vi "HandleObservationSync_001.vi"(8 "error in (no error)":errorcluster, 11 "S4ACS_GUI in":refnum<class "S4GUI.lvclass">) -> (0 "error out":errorcluster, 3 "S4ACS_GUI out":refnum<class "S4GUI.lvclass">)   [LabVIEW 2018, in "S4GUI.lvclass"]
uses:
  S4GUI.lvclass
  S4GUI.lvclass/S4GUI.ctl
  Instrument/Instrument.lvclass/Instrument.ctl
  Device/Optics/Optics.lvclass/Optics.ctl
  Server/Server.lvclass/Server.ctl
  Interface/Interface.lvclass/Interface.ctl
  Device/Optics/Opt_Selector/Opt_Selector.lvclass
  C:/Users/observer/Desktop/Sparc4GUI/SPARC4_GUI/Device/Optics/Optics.lvclass
  Acquisition/Acquisition.lvclass
  C:/Users/observer/Desktop/Sparc4GUI/SPARC4_GUI/Server/Server.lvclass
  SyncBox/Sync Box.lvclass
  Instrument/Instrument.lvclass
  Device/Optics/Opt_Continuous/Opt_Continuous.lvclass
  StateMachine/State Machine.lvclass
  Trigger/Trigger.lvclass
  Channel/Channel.lvclass
  Interface/Interface.lvclass
  Device/Optics/Optics.lvclass
  Server/Server.lvclass
panel:
  out "delay 3-4":u32
  out "time4":u32
  out "time3":u32
  out "time 2":u32
  out "time1":u32
  # "WAVEPLATE DURATION"
  # "ACS SETUP"
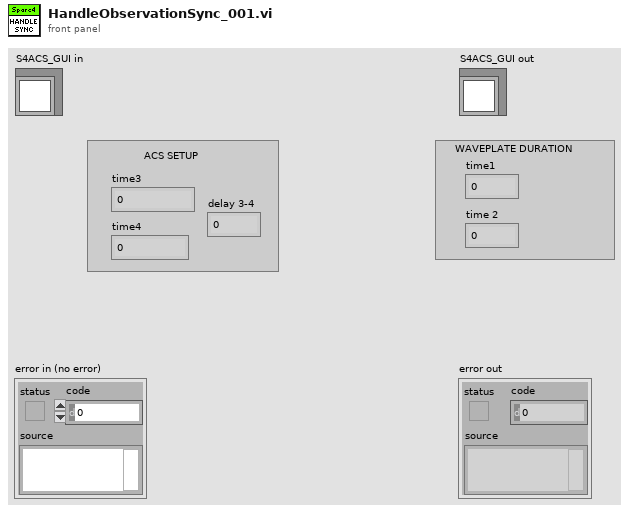
[diagram p1: front panel]
types:
  T1 = cluster{"ACQUISITION_MODE":u8, "TRIGGER_MODE":u8, "READ_MODE":u8, "PREAMP":u8, "READOUT_RATE":u8, "VERTICAL_SHIFT_SPEED":u8, "EM_MODE":u8, "EM_GAIN":u16, "SHUTTER_MODE":u8, "SHUTTER_TTL":u8, "SHUTTER_OPENING_TIME":u16, "SHUTTER_CLOSING_TIME":u16, "VBIN":u16, "HBIN":u16, "INITIAL_LINE":u16, "INITIAL_COLUMN":u16, "FINAL_LINE":u16, "FINAL_COLUMN":u16, "FRAME_TRANSFER":bool, "VERTICAL_CLOCK_VOLTAGE":u8, "AD_CHANNEL":u32}
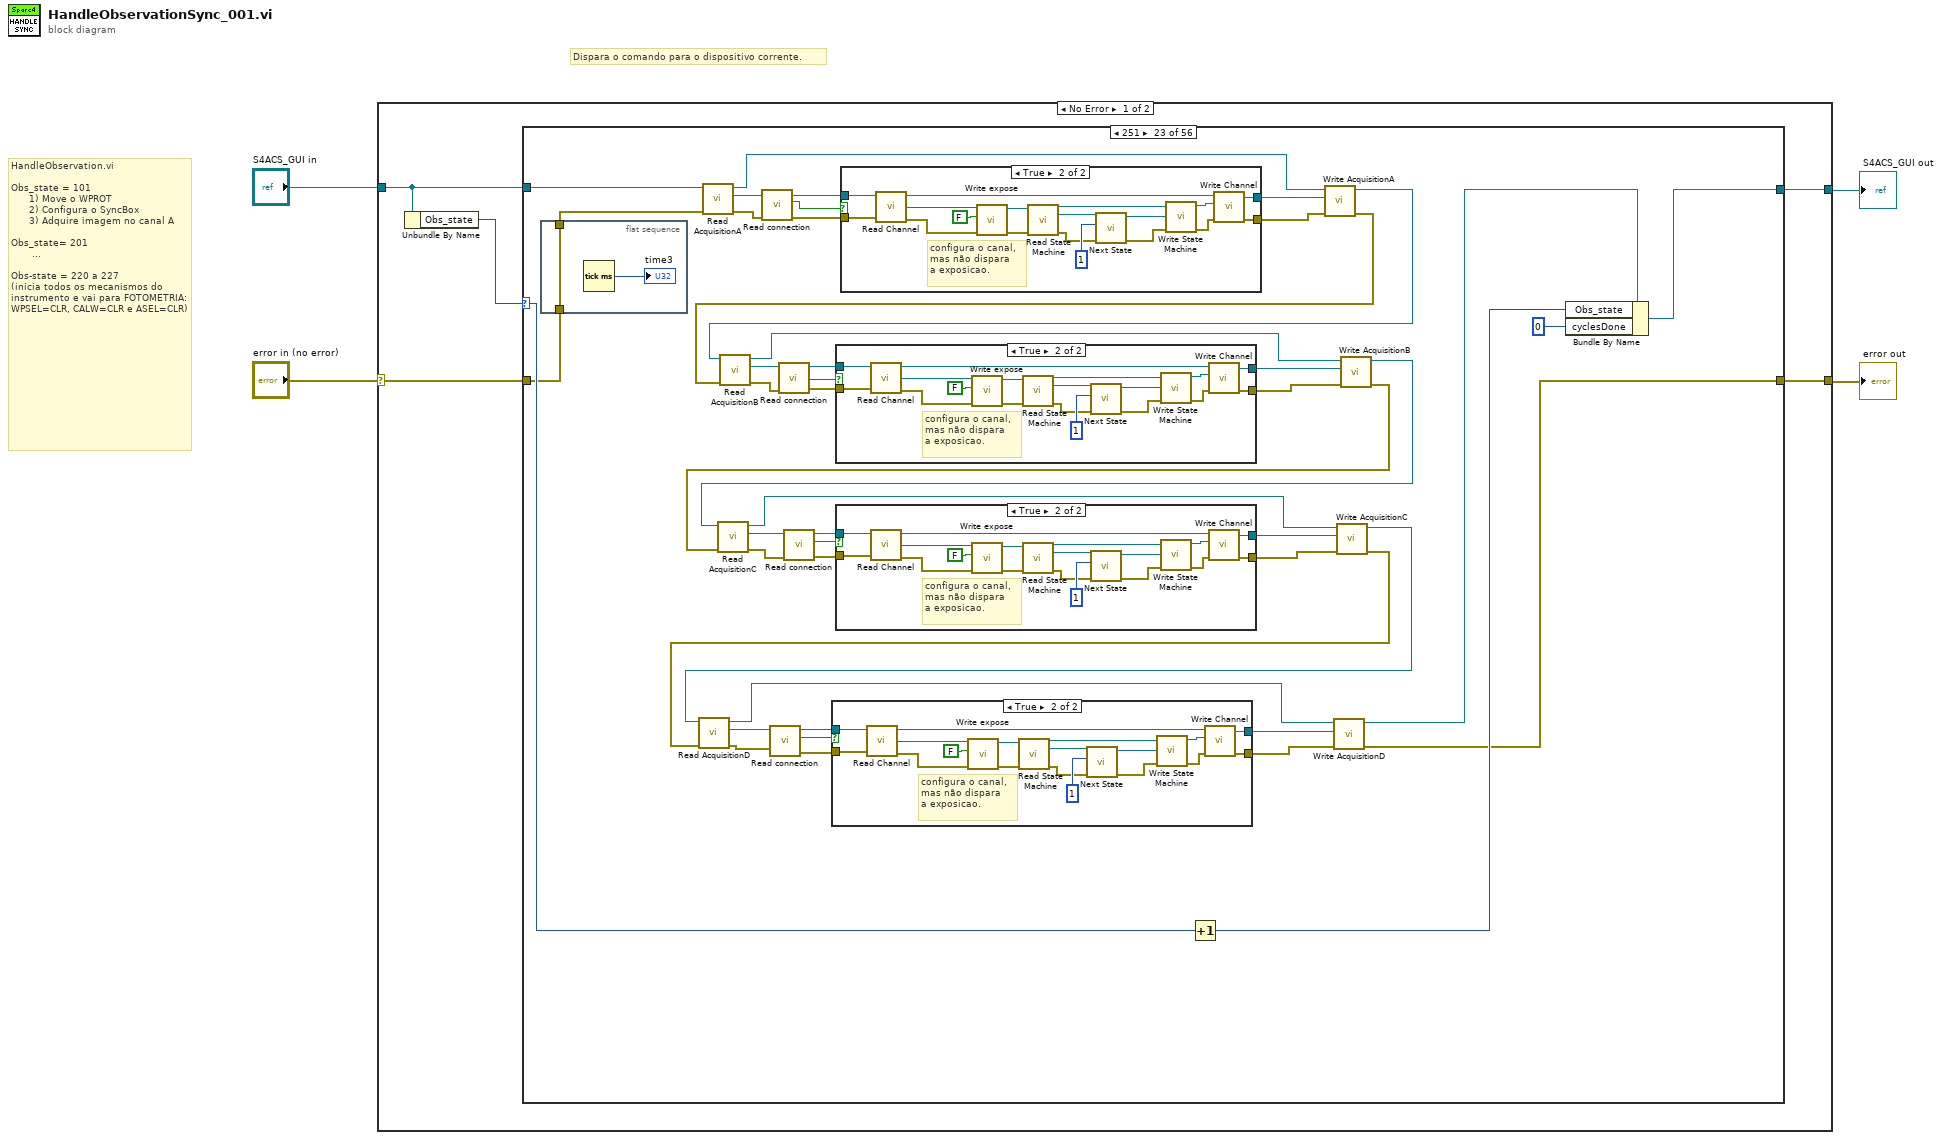
[diagram p0: block diagram]
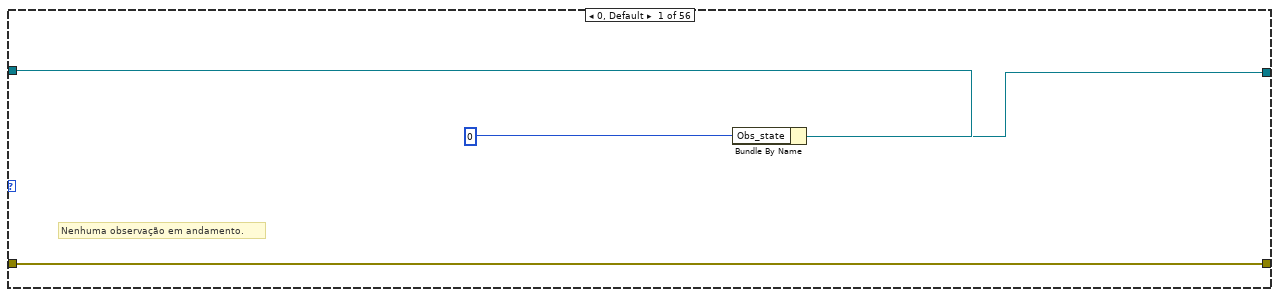
[diagram p2: hidden frame]
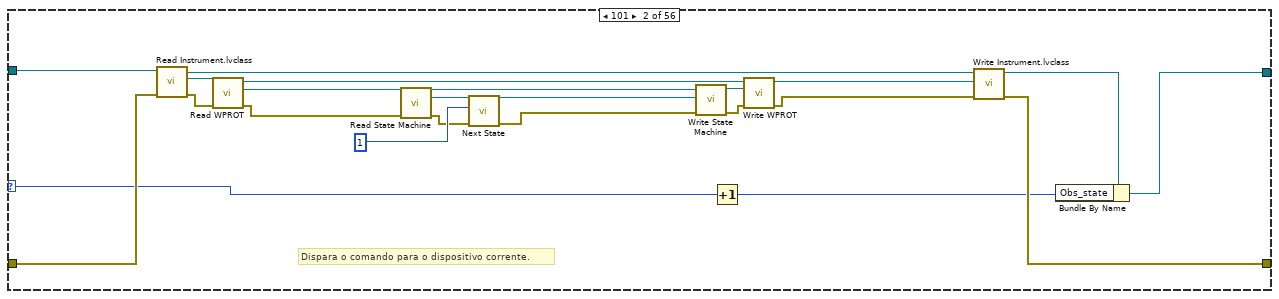
[diagram p3: hidden frame]
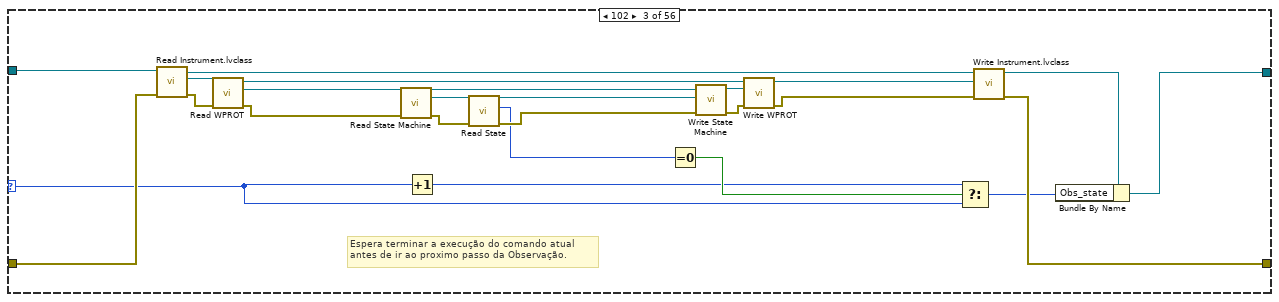
[diagram p4: hidden frame]
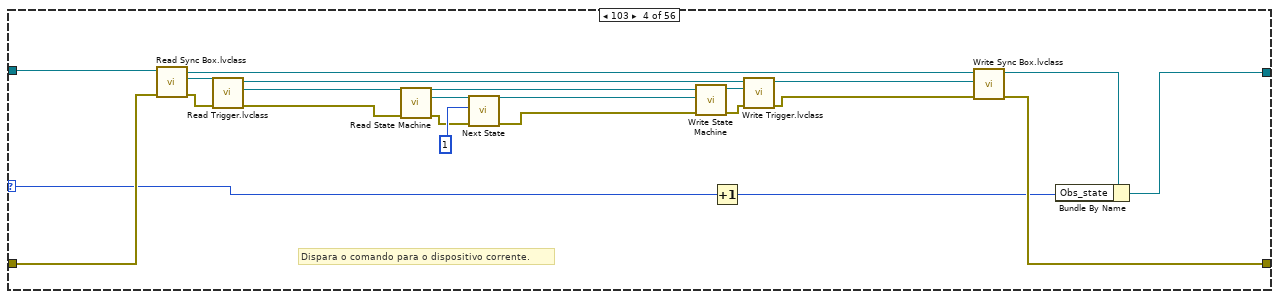
[diagram p5: hidden frame]
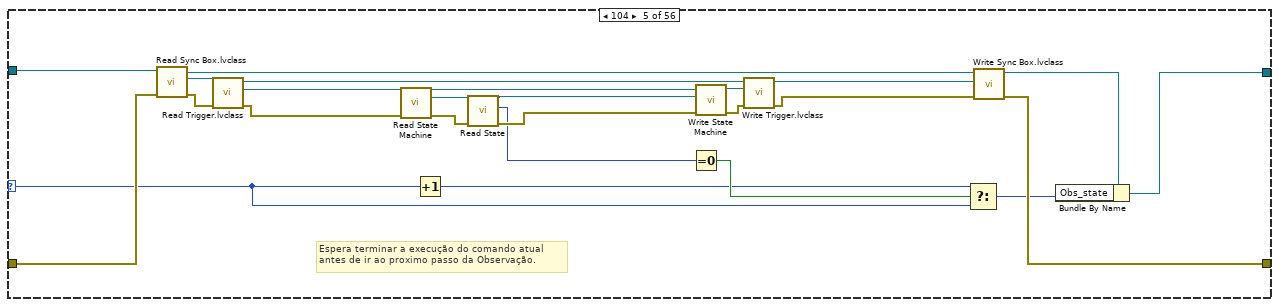
[diagram p6: hidden frame]
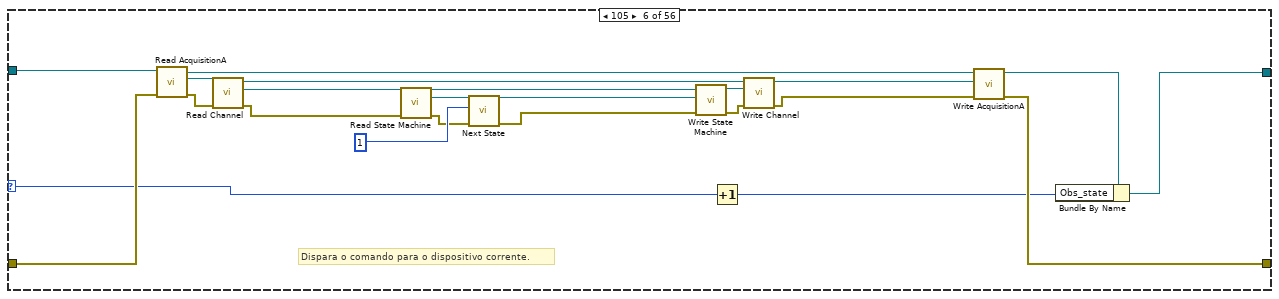
[diagram p7: hidden frame]
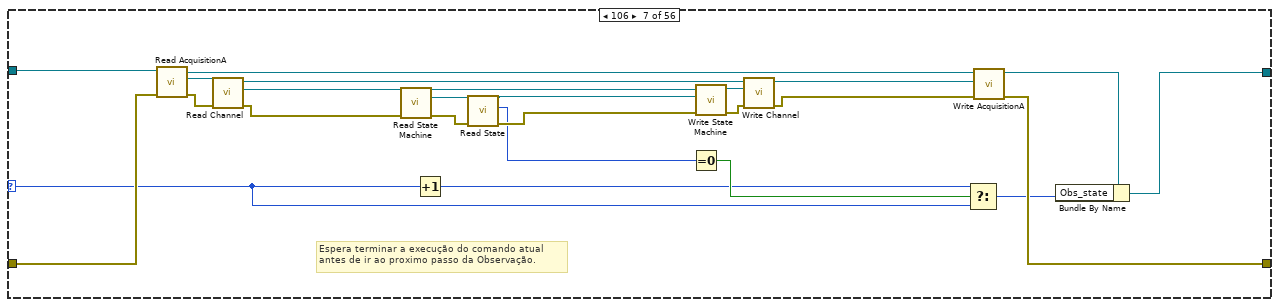
[diagram p8: hidden frame]
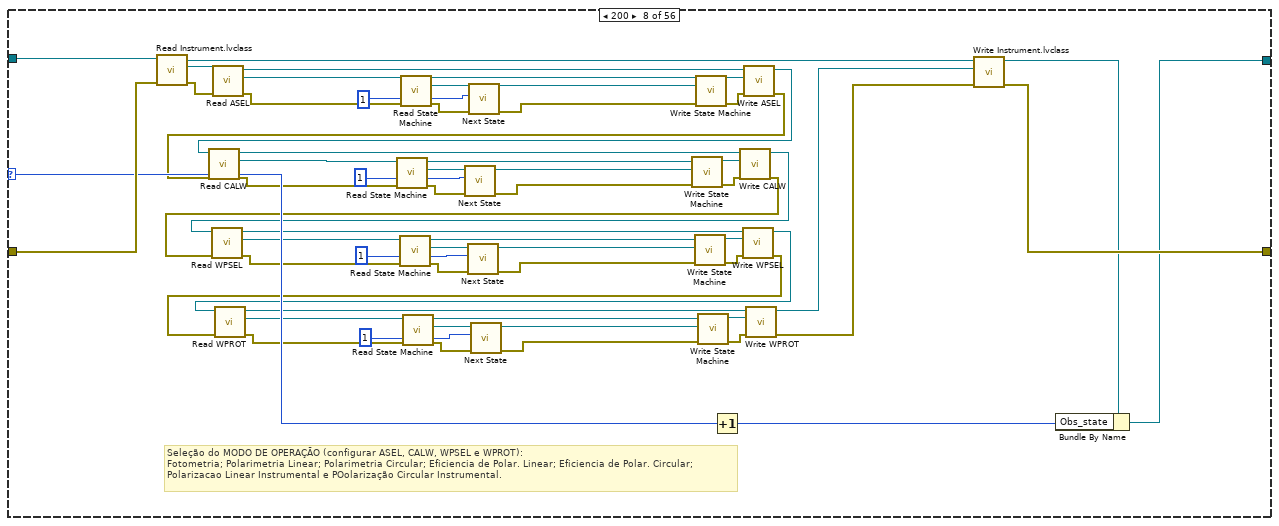
[diagram p9: hidden frame]
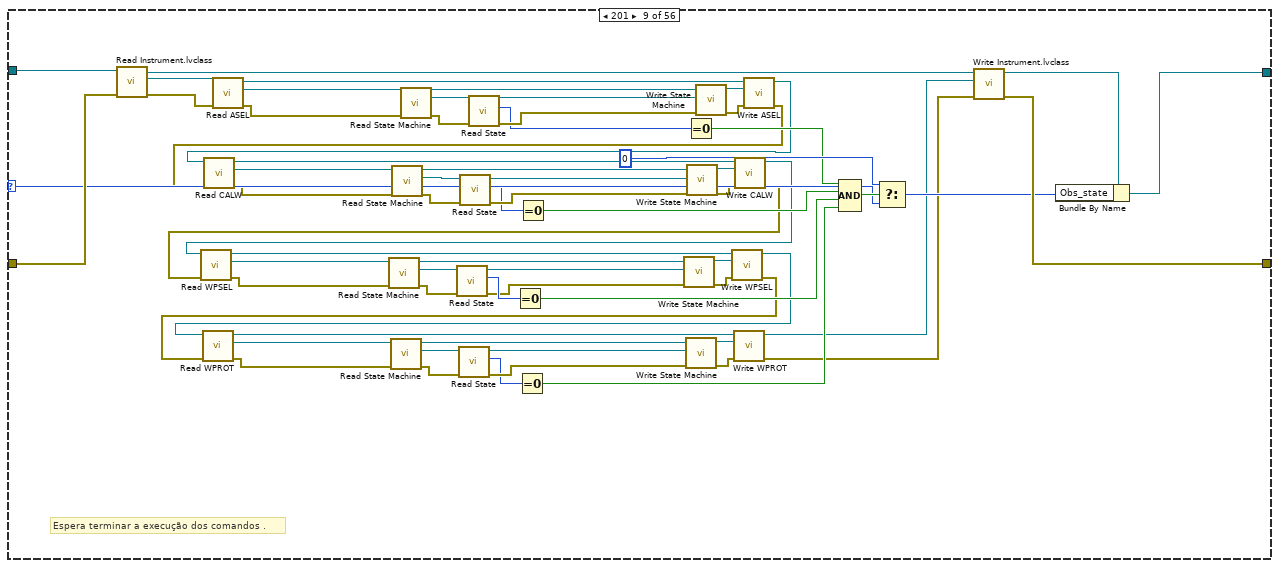
[diagram p10: hidden frame]
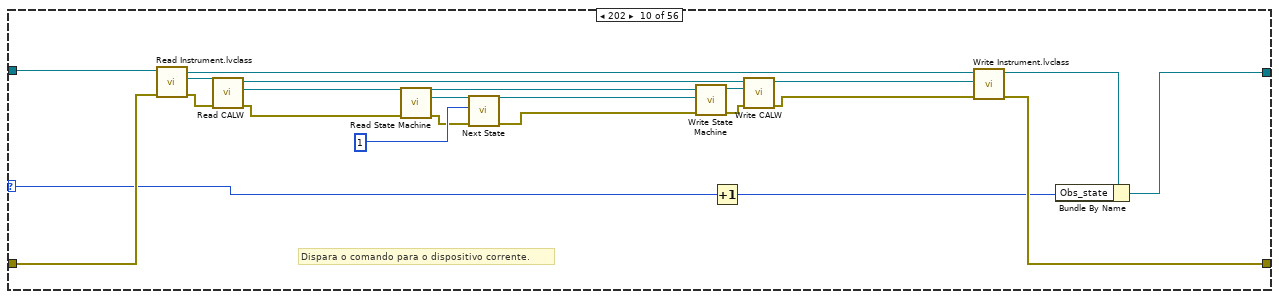
[diagram p11: hidden frame]
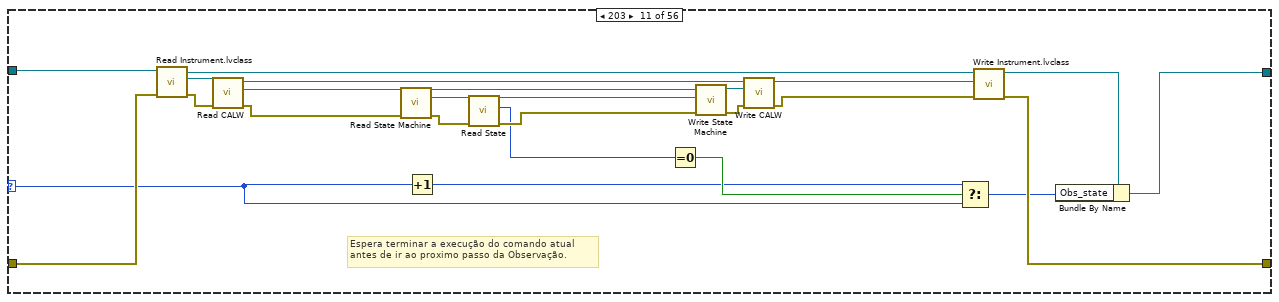
[diagram p12: hidden frame]
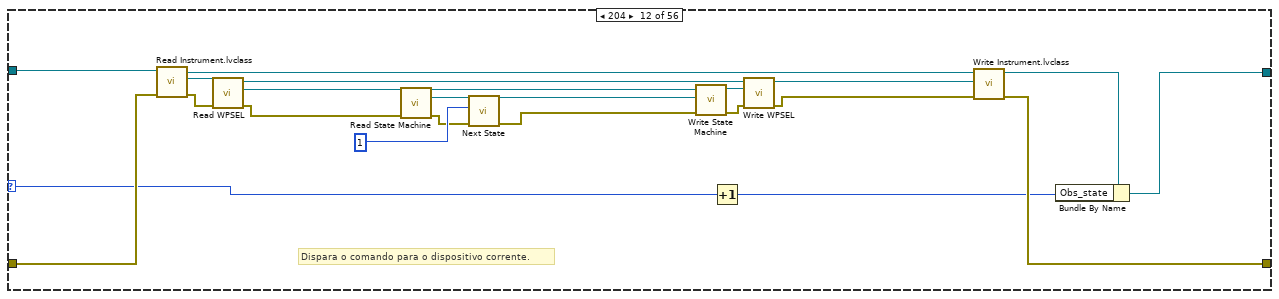
[diagram p13: hidden frame]
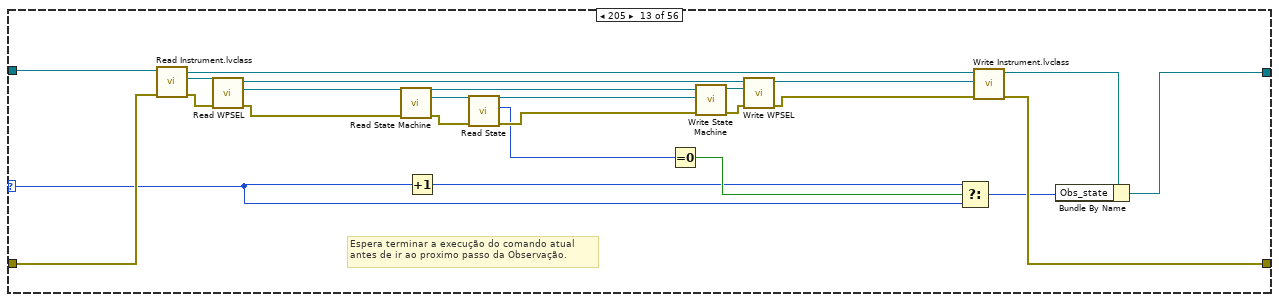
[diagram p14: hidden frame]
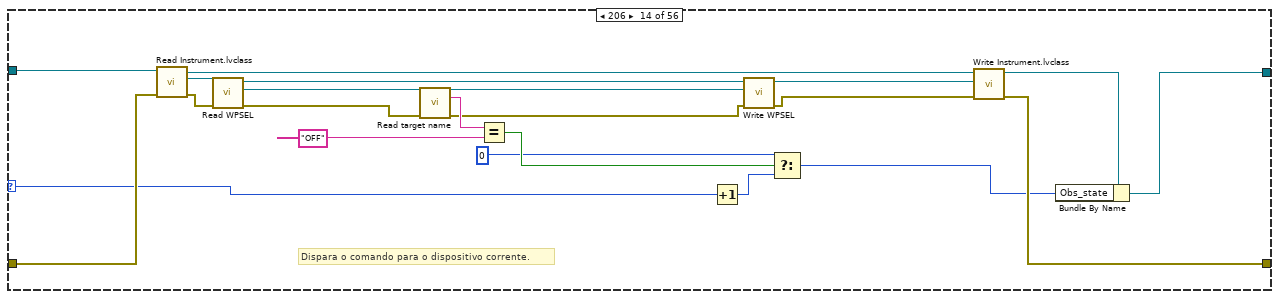
[diagram p15: hidden frame]
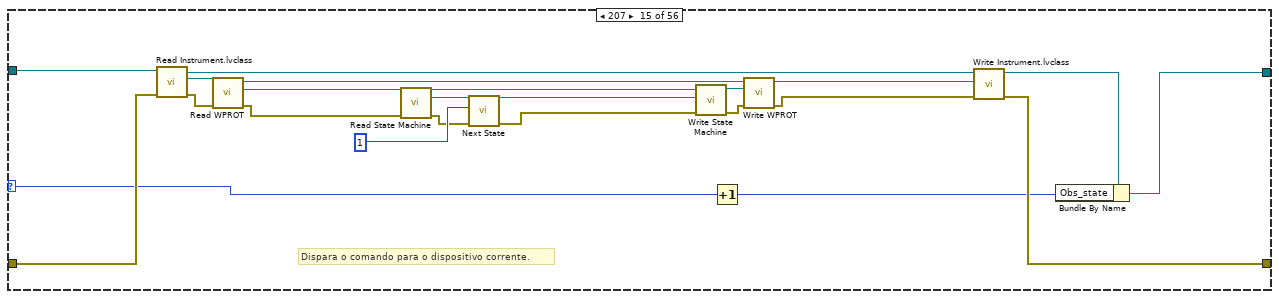
[diagram p16: hidden frame]
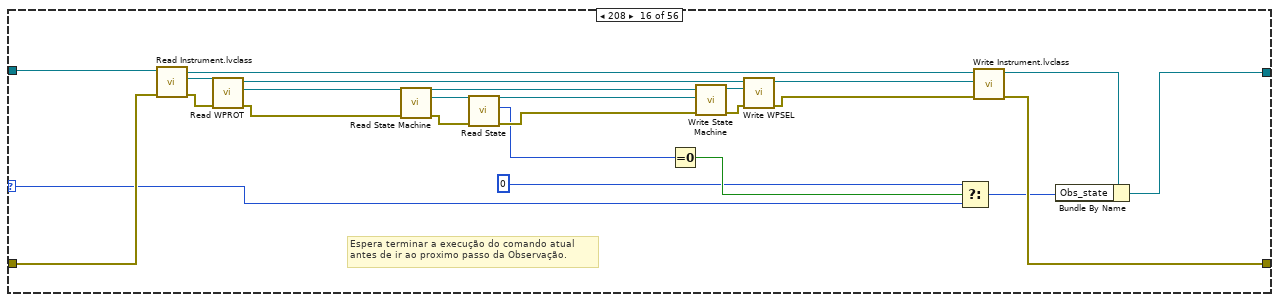
[diagram p17: hidden frame]
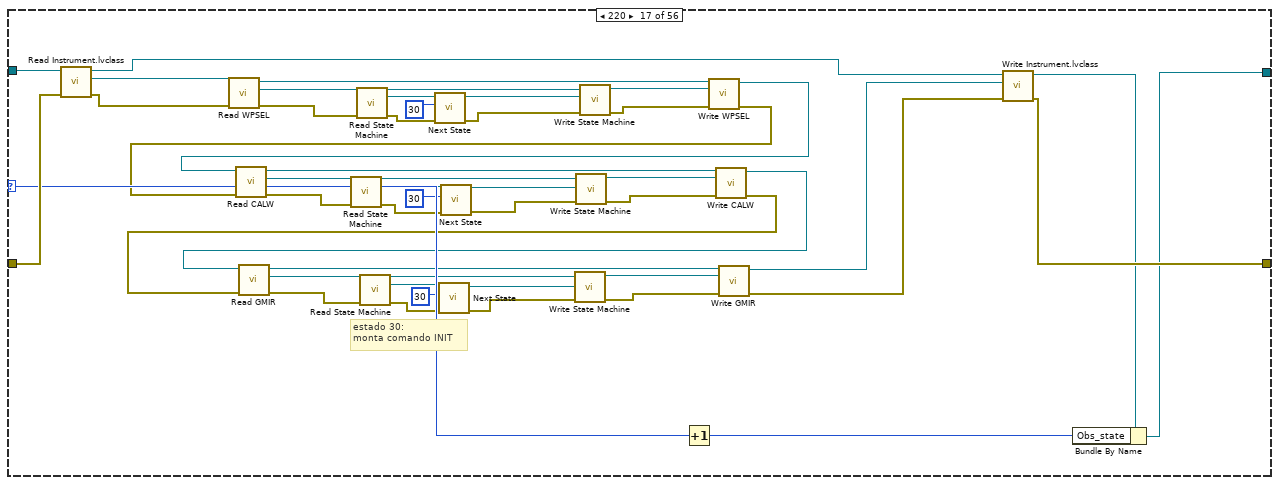
[diagram p18: hidden frame]
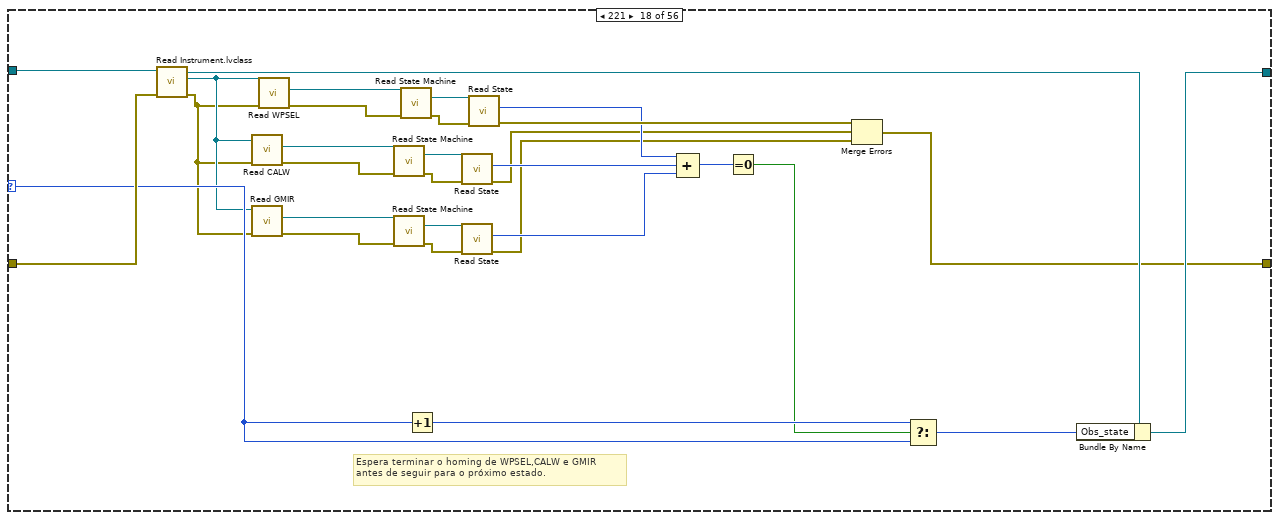
[diagram p19: hidden frame]
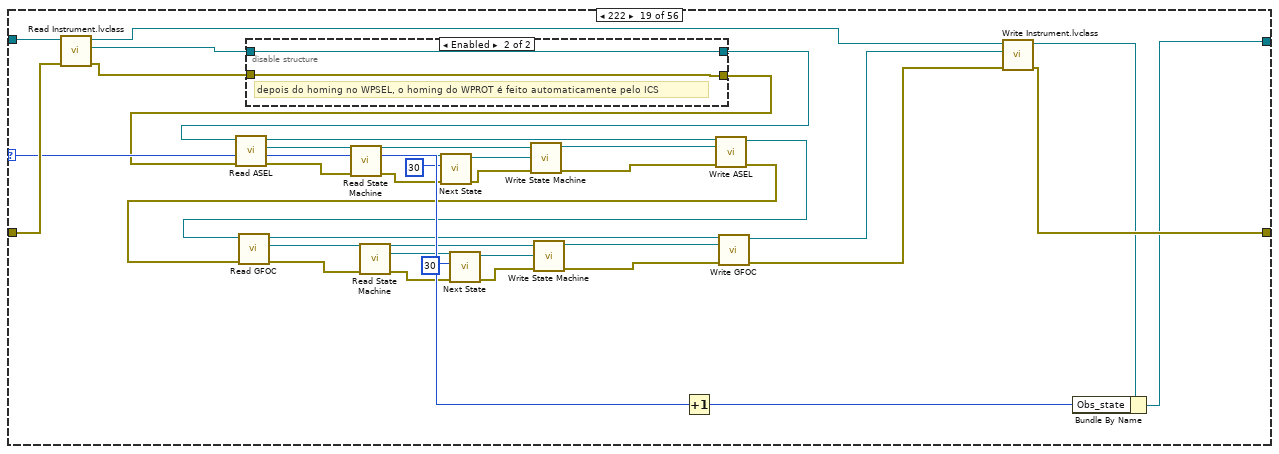
[diagram p20: hidden frame]
diagram:
  # "Dispara o comando para o dispositivo corrente."
  # "HandleObservation.vi\n\nObs_state = 101\n      1) Move o WPROT\n      2) Configura o SyncBox\n      3) Adquire imagem no canal A\n\nObs_state= 201\n       ...\n\nObs-state = 220 a 227 \n(inicia todos os mecanismos do instrumento e vai para FOTOMETRIA: WPSEL=CLR, CALW=CLR e ASEL=CLR)"
  n1 = case shown="No Error" "error in (no error)" {
    selector: "error in (no error)" -> [w8 w2964]
    tunnel: [w7 w2964] -> w3
    tunnel: [w9 w2963] -> w1
    tunnel: "S4ACS_GUI in" -> [w6 w2963]
    frame No Error {
      n2 = Unbundle By Name(w6) -> ("Obs_state"=w5:u32)
      n3 = case shown="251" w5 {
        selector: w5 -> [_ w16 w38 w64 w86 w112 w134 w202 w265 w290 w312 w338 w360 w395 w408 w430 w492 w524 w563 w609 w689 w721 w767 w904 w1029 w1032 w1067 w1103 w1175 w1179 w1210 w1246 w1318 w1322 w1353 w1385 w1455 w1459 _ w1536 w1581 w1653 w1733 w1867 w2024 _ _ w2263 _ w2411 w2523 w2620 w2770 w2841 _ _]
        tunnel: w6 -> [w12 w30 w55 w78 w103 w126 w151 w216 w283 w304 w329 w352 w377 w399 w422 w447 w501 w532 w569 w613 w698 w729 w773 w908 w1022 w1050 w1071 w1120 w1168 w1196 w1214 w1263 w1311 w1339 w1357 w1402 w1448 w1476 w1496 w1539 w1603 w1655 w1774 w1871 w2022 w2062 w2194 w2272 w2361 w2370 w2527 w2624 w2783 w2803 w2931 w2962]
        tunnel: [w10 w14 w42 w62 w94 w110 w142 w200 w270 w288 w316 w336 w364 w394 w406 w434 w496 w526 w564 w611 w693 w723 w772 w907 w1027 w1041 w1065 w1111 w1173 w1187 w1208 w1254 w1316 w1330 w1351 w1393 w1453 w1467 w1495 w1534 w1584 w1651 w1772 w1865 w2030 w2100 w2191 w2270 w2357 w2409 w2525 w2618 w2776 w2842 w2928 w2962] -> w9
        tunnel: w8 -> [w13 w29 w54 w77 w102 w125 w150 w215 w282 w303 w328 w351 w376 w398 w421 w446 w500 w531 w568 w612 w697 w728 w748 w890 w1023 w1049 w1070 w1119 w1169 w1195 w1213 w1262 w1312 w1338 w1356 w1401 w1449 w1475 w1486 w1504 w1594 w1654 w1773 w1870 w2020 w2101 w2193 w2271 w2360 w2369 w2526 w2623 w2782 w2843 w2930 w2961]
        tunnel: [w13 w28 w53 w76 w101 w124 w149 w214 w281 w302 w327 w350 w375 w397 w420 w445 w499 w505 w567 w590 w696 w703 w750 w892 w1020 w1048 w1069 w1118 w1166 w1194 w1212 w1261 w1309 w1337 w1355 w1400 w1446 w1474 w1487 w1538 w1580 w1635 w1755 w1869 w2012 w2083 w2192 w2245 w2359 w2367 w2505 w2622 w2765 w2824 w2929 w2961] -> w7
        frame 0, Default {
          # "Nenhuma observação em andamento."
          n4 = Bundle By Name(cluster=w12, "Obs_state"=u32 0) -> (w10:refnum<class "S4GUI.lvclass">)
        }
        frame 101 {
          # "Dispara o comando para o dispositivo corrente."
          n5 = call "Read Instrument.lvclass.vi"("error in (no error)"=w29, "S4ACS_GUI in"=w30) -> ("error out"=w35:errorcluster, "Instrument.lvclass"=w36:refnum<class "Instrument.lvclass">, "S4ACS_GUI out"=w32:refnum<class "S4GUI.lvclass">)  [unwired: 7 in]
          n6 = call "Read WPROT.vi"("error in (no error)"=w35, "Instrument in"=w36) -> ("error out"=w22:errorcluster, "Opt_Selector.lvclass"=w21:refnum<class "Opt_Selector.lvclass">, "Instrument out"=w34:refnum<class "Instrument.lvclass">)  [unwired: 7 in]
          n7 = call-dynamic "Read State Machine.vi"("error in (no error)"=w22, "Device in"=w21) -> ("error out"=w25:errorcluster, "State Machine.lvclass"=w27:refnum<class "State Machine.lvclass">, "Device out"=w19:refnum<class "Opt_Selector.lvclass">)  [unwired: 7 in]
          n8 = call "Next State.vi"("error in (no error)"=w25, "New_State"=1, "State Machine in"=w27) -> ("error out"=w24:errorcluster, "State Machine out"=w23:refnum<class "State Machine.lvclass">)  [unwired: 7 in]
          n9 = call-dynamic "Write State Machine.vi"("error in (no error)"=w24, "State Machine.lvclass"=w23, "Device in"=w19) -> ("error out"=w18:errorcluster, "Device out"=w20:refnum<class "Opt_Selector.lvclass">)  [unwired: 7 in]
          n10 = Increment(x=w16) -> (x+1=w15:u32)
          n11 = call "Write WPROT.vi"("error in (no error)"=w18, "Opt_Selector.lvclass"=w20, "Instrument in"=w34) -> ("error out"=w31:errorcluster, "Instrument out"=w33:refnum<class "Instrument.lvclass">)  [unwired: 7 in]
          n12 = call "Write Instrument.lvclass.vi"("error in (no error)"=w31, "Instrument.lvclass"=w33, "S4ACS_GUI in"=w32) -> ("error out"=w28:errorcluster, "S4ACS_GUI out"=w17:refnum<class "S4GUI.lvclass">)  [unwired: 7 in]
          n13 = Bundle By Name(cluster=w17, "Obs_state"=w15) -> (w14:refnum<class "S4GUI.lvclass">)
        }
        frame 102 {
          # "Espera terminar a execução do comando atual \nantes de ir ao proximo passo da Observação."
          n14 = call "Read Instrument.lvclass.vi"("error in (no error)"=w54, "S4ACS_GUI in"=w55) -> ("error out"=w60:errorcluster, "Instrument.lvclass"=w61:refnum<class "Instrument.lvclass">, "S4ACS_GUI out"=w57:refnum<class "S4GUI.lvclass">)  [unwired: 7 in]
          n15 = call "Read WPROT.vi"("error in (no error)"=w60, "Instrument in"=w61) -> ("error out"=w48:errorcluster, "Opt_Selector.lvclass"=w47:refnum<class "Opt_Selector.lvclass">, "Instrument out"=w59:refnum<class "Instrument.lvclass">)  [unwired: 7 in]
          n16 = call-dynamic "Read State Machine.vi"("error in (no error)"=w48, "Device in"=w47) -> ("error out"=w51:errorcluster, "State Machine.lvclass"=w52:refnum<class "State Machine.lvclass">, "Device out"=w45:refnum<class "Opt_Selector.lvclass">)  [unwired: 7 in]
          n17 = Increment(x=w38) -> (x+1=w37:u32)
          n18 = call-dynamic "Read State.vi"("error in (no error)"=w51, "State Machine in"=w52) -> ("error out"=w50:errorcluster, "State"=w40:i32, "State Machine out"=w49:refnum<class "State Machine.lvclass">)  [unwired: 7 in]
          n19 = Equal To 0?(x=w40) -> (x = 0?=w41:bool)
          n20 = call-dynamic "Write State Machine.vi"("error in (no error)"=w50, "State Machine.lvclass"=w49, "Device in"=w45) -> ("error out"=w44:errorcluster, "Device out"=w46:refnum<class "Opt_Selector.lvclass">)  [unwired: 7 in]
          n21 = call "Write WPROT.vi"("error in (no error)"=w44, "Opt_Selector.lvclass"=w46, "Instrument in"=w59) -> ("error out"=w56:errorcluster, "Instrument out"=w58:refnum<class "Instrument.lvclass">)  [unwired: 7 in]
          n22 = Select(t=w37, s=w41, f=w38) -> (s? t:f=w39:u32)
          n23 = call "Write Instrument.lvclass.vi"("error in (no error)"=w56, "Instrument.lvclass"=w58, "S4ACS_GUI in"=w57) -> ("error out"=w53:errorcluster, "S4ACS_GUI out"=w43:refnum<class "S4GUI.lvclass">)  [unwired: 7 in]
          n24 = Bundle By Name(cluster=w43, "Obs_state"=w39) -> (w42:refnum<class "S4GUI.lvclass">)
        }
        frame 103 {
          # "Dispara o comando para o dispositivo corrente."
          n25 = call-dynamic "Read Sync Box.lvclass.vi"("error in (no error)"=w77, "SPARC4_AC in"=w78) -> ("error out"=w83:errorcluster, "Sync Box.lvclass"=w84:refnum<class "Sync Box.lvclass">, "SPARC4_AC out"=w80:refnum<class "S4GUI.lvclass">)  [unwired: 7 in]
          n26 = call-dynamic "Read Trigger.lvclass.vi"("error in (no error)"=w83, "Sync Box in"=w84) -> ("error out"=w70:errorcluster, "Trigger.lvclass"=w69:refnum<class "Trigger.lvclass">, "Sync Box out"=w82:refnum<class "Sync Box.lvclass">)  [unwired: 7 in]
          n27 = call-dynamic "Read State Machine.vi"("error in (no error)"=w70, "Device in"=w69) -> ("error out"=w73:errorcluster, "State Machine.lvclass"=w75:refnum<class "State Machine.lvclass">, "Device out"=w67:refnum<class "Trigger.lvclass">)  [unwired: 7 in]
          n28 = call "Next State.vi"("error in (no error)"=w73, "New_State"=1, "State Machine in"=w75) -> ("error out"=w72:errorcluster, "State Machine out"=w71:refnum<class "State Machine.lvclass">)  [unwired: 7 in]
          n29 = call-dynamic "Write State Machine.vi"("error in (no error)"=w72, "State Machine.lvclass"=w71, "Device in"=w67) -> ("error out"=w66:errorcluster, "Device out"=w68:refnum<class "Trigger.lvclass">)  [unwired: 7 in]
          n30 = Increment(x=w64) -> (x+1=w63:u32)
          n31 = call-dynamic "Write Trigger.lvclass.vi"("error in (no error)"=w66, "Trigger.lvclass"=w68, "Sync Box in"=w82) -> ("error out"=w79:errorcluster, "Sync Box out"=w81:refnum<class "Sync Box.lvclass">)  [unwired: 7 in]
          n32 = call-dynamic "Write Sync Box.lvclass.vi"("error in (no error)"=w79, "Sync Box.lvclass"=w81, "SPARC4_AC in"=w80) -> ("error out"=w76:errorcluster, "SPARC4_AC out"=w65:refnum<class "S4GUI.lvclass">)  [unwired: 7 in]
          n33 = Bundle By Name(cluster=w65, "Obs_state"=w63) -> (w62:refnum<class "S4GUI.lvclass">)
        }
        frame 104 {
          # "Espera terminar a execução do comando atual \nantes de ir ao proximo passo da Observação."
          n34 = call-dynamic "Read Sync Box.lvclass.vi"("error in (no error)"=w102, "SPARC4_AC in"=w103) -> ("error out"=w108:errorcluster, "Sync Box.lvclass"=w109:refnum<class "Sync Box.lvclass">, "SPARC4_AC out"=w105:refnum<class "S4GUI.lvclass">)  [unwired: 7 in]
          n35 = call-dynamic "Read Trigger.lvclass.vi"("error in (no error)"=w108, "Sync Box in"=w109) -> ("error out"=w100:errorcluster, "Trigger.lvclass"=w99:refnum<class "Trigger.lvclass">, "Sync Box out"=w107:refnum<class "Sync Box.lvclass">)  [unwired: 7 in]
          n36 = call-dynamic "Read State Machine.vi"("error in (no error)"=w100, "Device in"=w99) -> ("error out"=w91:errorcluster, "State Machine.lvclass"=w93:refnum<class "State Machine.lvclass">, "Device out"=w97:refnum<class "Trigger.lvclass">)  [unwired: 7 in]
          n37 = Increment(x=w86) -> (x+1=w88:u32)
          n38 = call-dynamic "Read State.vi"("error in (no error)"=w91, "State Machine in"=w93) -> ("error out"=w90:errorcluster, "State"=w85:i32, "State Machine out"=w92:refnum<class "State Machine.lvclass">)  [unwired: 7 in]
          n39 = Equal To 0?(x=w85) -> (x = 0?=w89:bool)
          n40 = call-dynamic "Write State Machine.vi"("error in (no error)"=w90, "State Machine.lvclass"=w92, "Device in"=w97) -> ("error out"=w96:errorcluster, "Device out"=w98:refnum<class "Trigger.lvclass">)  [unwired: 7 in]
          n41 = call-dynamic "Write Trigger.lvclass.vi"("error in (no error)"=w96, "Trigger.lvclass"=w98, "Sync Box in"=w107) -> ("error out"=w104:errorcluster, "Sync Box out"=w106:refnum<class "Sync Box.lvclass">)  [unwired: 7 in]
          n42 = Select(t=w88, s=w89, f=w86) -> (s? t:f=w87:u32)
          n43 = call-dynamic "Write Sync Box.lvclass.vi"("error in (no error)"=w104, "Sync Box.lvclass"=w106, "SPARC4_AC in"=w105) -> ("error out"=w101:errorcluster, "SPARC4_AC out"=w95:refnum<class "S4GUI.lvclass">)  [unwired: 7 in]
          n44 = Bundle By Name(cluster=w95, "Obs_state"=w87) -> (w94:refnum<class "S4GUI.lvclass">)
        }
        frame 105 {
          # "Dispara o comando para o dispositivo corrente."
          n45 = call-dynamic "Read AcquisitionA.vi"("error in (no error)"=w125, "S4ACS_GUI in"=w126) -> ("error out"=w131:errorcluster, "Acquisition.lvclass"=w132:refnum<class "Acquisition.lvclass">, "S4ACS_GUI out"=w128:refnum<class "S4GUI.lvclass">)  [unwired: 7 in]
          n46 = call-dynamic "Read Channel.vi"("error in (no error)"=w131, "Acquisition in"=w132) -> ("error out"=w118:errorcluster, "Channel.lvclass"=w117:refnum<class "Channel.lvclass">, "Acquisition out"=w130:refnum<class "Acquisition.lvclass">)  [unwired: 7 in]
          n47 = call-dynamic "Read State Machine.vi"("error in (no error)"=w118, "Device in"=w117) -> ("error out"=w121:errorcluster, "State Machine.lvclass"=w123:refnum<class "State Machine.lvclass">, "Device out"=w115:refnum<class "Channel.lvclass">)  [unwired: 7 in]
          n48 = call "Next State.vi"("error in (no error)"=w121, "New_State"=1, "State Machine in"=w123) -> ("error out"=w120:errorcluster, "State Machine out"=w119:refnum<class "State Machine.lvclass">)  [unwired: 7 in]
          n49 = call-dynamic "Write State Machine.vi"("error in (no error)"=w120, "State Machine.lvclass"=w119, "Device in"=w115) -> ("error out"=w114:errorcluster, "Device out"=w116:refnum<class "Channel.lvclass">)  [unwired: 7 in]
          n50 = Increment(x=w112) -> (x+1=w111:u32)
          n51 = call-dynamic "Write Channel.vi"("error in (no error)"=w114, "Channel.lvclass"=w116, "Acquisition in"=w130) -> ("error out"=w127:errorcluster, "Acquisition out"=w129:refnum<class "Acquisition.lvclass">)  [unwired: 7 in]
          n52 = call-dynamic "Write AcquisitionA.vi"("error in (no error)"=w127, "Acquisition.lvclass"=w129, "S4ACS_GUI in"=w128) -> ("error out"=w124:errorcluster, "S4ACS_GUI out"=w113:refnum<class "S4GUI.lvclass">)  [unwired: 7 in]
          n53 = Bundle By Name(cluster=w113, "Obs_state"=w111) -> (w110:refnum<class "S4GUI.lvclass">)
        }
        frame 106 {
          # "Espera terminar a execução do comando atual \nantes de ir ao proximo passo da Observação."
          n54 = call-dynamic "Read AcquisitionA.vi"("error in (no error)"=w150, "S4ACS_GUI in"=w151) -> ("error out"=w156:errorcluster, "Acquisition.lvclass"=w157:refnum<class "Acquisition.lvclass">, "S4ACS_GUI out"=w153:refnum<class "S4GUI.lvclass">)  [unwired: 7 in]
          n55 = call-dynamic "Read Channel.vi"("error in (no error)"=w156, "Acquisition in"=w157) -> ("error out"=w148:errorcluster, "Channel.lvclass"=w147:refnum<class "Channel.lvclass">, "Acquisition out"=w155:refnum<class "Acquisition.lvclass">)  [unwired: 7 in]
          n56 = call-dynamic "Read State Machine.vi"("error in (no error)"=w148, "Device in"=w147) -> ("error out"=w139:errorcluster, "State Machine.lvclass"=w141:refnum<class "State Machine.lvclass">, "Device out"=w145:refnum<class "Channel.lvclass">)  [unwired: 7 in]
          n57 = Increment(x=w134) -> (x+1=w136:u32)
          n58 = call-dynamic "Read State.vi"("error in (no error)"=w139, "State Machine in"=w141) -> ("error out"=w138:errorcluster, "State"=w133:i32, "State Machine out"=w140:refnum<class "State Machine.lvclass">)  [unwired: 7 in]
          n59 = Equal To 0?(x=w133) -> (x = 0?=w137:bool)
          n60 = call-dynamic "Write State Machine.vi"("error in (no error)"=w138, "State Machine.lvclass"=w140, "Device in"=w145) -> ("error out"=w144:errorcluster, "Device out"=w146:refnum<class "Channel.lvclass">)  [unwired: 7 in]
          n61 = call-dynamic "Write Channel.vi"("error in (no error)"=w144, "Channel.lvclass"=w146, "Acquisition in"=w155) -> ("error out"=w152:errorcluster, "Acquisition out"=w154:refnum<class "Acquisition.lvclass">)  [unwired: 7 in]
          n62 = Select(t=w136, s=w137, f=w134) -> (s? t:f=w135:u32)
          n63 = call-dynamic "Write AcquisitionA.vi"("error in (no error)"=w152, "Acquisition.lvclass"=w154, "S4ACS_GUI in"=w153) -> ("error out"=w149:errorcluster, "S4ACS_GUI out"=w143:refnum<class "S4GUI.lvclass">)  [unwired: 7 in]
          n64 = Bundle By Name(cluster=w143, "Obs_state"=w135) -> (w142:refnum<class "S4GUI.lvclass">)
        }
        frame 200 {
          # "Seleção do MODO DE OPERAÇÃO (configurar ASEL, CALW, WPSEL e WPROT): \nFotometria; Polarimetria Linear; Polarimetria Circular; Eficiencia de Polar. Linear; Eficiencia de Polar. Circular;\nPolarizacao Linear Instrumental e POolarização Circular Instrumental."
          n65 = call "Read Instrument.lvclass.vi"("error in (no error)"=w215, "S4ACS_GUI in"=w216) -> ("error out"=w219:errorcluster, "Instrument.lvclass"=w179:refnum<class "Instrument.lvclass">, "S4ACS_GUI out"=w217:refnum<class "S4GUI.lvclass">)  [unwired: 7 in]
          n66 = call "Read ASEL.vi"("error in (no error)"=w219, "Instrument in"=w179) -> ("error out"=w208:errorcluster, "Opt_Selector.lvclass"=w207:refnum<class "Opt_Selector.lvclass">, "Instrument out"=w218:refnum<class "Instrument.lvclass">)  [unwired: 7 in]
          n67 = call-dynamic "Read State Machine.vi"("error in (no error)"=w208, "Device in"=w207) -> ("error out"=w211:errorcluster, "State Machine.lvclass"=w213:refnum<class "State Machine.lvclass">, "Device out"=w205:refnum<class "Opt_Selector.lvclass">)  [unwired: 7 in]
          n68 = call "Next State.vi"("error in (no error)"=w211, "New_State"=1, "State Machine in"=w213) -> ("error out"=w210:errorcluster, "State Machine out"=w209:refnum<class "State Machine.lvclass">)  [unwired: 7 in]
          n69 = call-dynamic "Write State Machine.vi"("error in (no error)"=w210, "State Machine.lvclass"=w209, "Device in"=w205) -> ("error out"=w204:errorcluster, "Device out"=w206:refnum<class "Opt_Selector.lvclass">)  [unwired: 7 in]
          n70 = Increment(x=w202) -> (x+1=w201:u32)
          n71 = call "Write ASEL.vi"("error in (no error)"=w204, "Opt_Selector.lvclass"=w206, "Instrument in"=w218) -> ("error out"=w160:errorcluster, "Instrument out"=w178:refnum<class "Instrument.lvclass">)  [unwired: 7 in]
          n72 = call "Read CALW.vi"("error in (no error)"=w160, "Instrument in"=w178) -> ("error out"=w195:errorcluster, "Opt_Selector.lvclass"=w196:refnum<class "Opt_Selector.lvclass">, "Instrument out"=w177:refnum<class "Instrument.lvclass">)  [unwired: 7 in]
          n73 = call-dynamic "Read State Machine.vi"("error in (no error)"=w195, "Device in"=w196) -> ("error out"=w192:errorcluster, "State Machine.lvclass"=w190:refnum<class "State Machine.lvclass">, "Device out"=w198:refnum<class "Opt_Selector.lvclass">)  [unwired: 7 in]
          n74 = call "Next State.vi"("error in (no error)"=w192, "New_State"=1, "State Machine in"=w190) -> ("error out"=w193:errorcluster, "State Machine out"=w194:refnum<class "State Machine.lvclass">)  [unwired: 7 in]
          n75 = call-dynamic "Write State Machine.vi"("error in (no error)"=w193, "State Machine.lvclass"=w194, "Device in"=w198) -> ("error out"=w199:errorcluster, "Device out"=w197:refnum<class "Opt_Selector.lvclass">)  [unwired: 7 in]
          n76 = call "Write CALW.vi"("error in (no error)"=w199, "Opt_Selector.lvclass"=w197, "Instrument in"=w177) -> ("error out"=w159:errorcluster, "Instrument out"=w176:refnum<class "Instrument.lvclass">)  [unwired: 7 in]
          n77 = call "Read WPSEL.vi"("error in (no error)"=w159, "Instrument in"=w176) -> ("error out"=w184:errorcluster, "Opt_Selector.lvclass"=w183:refnum<class "Opt_Selector.lvclass">, "Instrument out"=w175:refnum<class "Instrument.lvclass">)  [unwired: 7 in]
          n78 = call-dynamic "Read State Machine.vi"("error in (no error)"=w184, "Device in"=w183) -> ("error out"=w187:errorcluster, "State Machine.lvclass"=w189:refnum<class "State Machine.lvclass">, "Device out"=w181:refnum<class "Opt_Selector.lvclass">)  [unwired: 7 in]
          n79 = call "Next State.vi"("error in (no error)"=w187, "New_State"=1, "State Machine in"=w189) -> ("error out"=w186:errorcluster, "State Machine out"=w185:refnum<class "State Machine.lvclass">)  [unwired: 7 in]
          n80 = call-dynamic "Write State Machine.vi"("error in (no error)"=w186, "State Machine.lvclass"=w185, "Device in"=w181) -> ("error out"=w180:errorcluster, "Device out"=w182:refnum<class "Opt_Selector.lvclass">)  [unwired: 7 in]
          n81 = call "Write WPSEL.vi"("error in (no error)"=w180, "Opt_Selector.lvclass"=w182, "Instrument in"=w175) -> ("error out"=w158:errorcluster, "Instrument out"=w164:refnum<class "Instrument.lvclass">)  [unwired: 7 in]
          n82 = call "Read WPROT.vi"("error in (no error)"=w158, "Instrument in"=w164) -> ("error out"=w170:errorcluster, "Opt_Selector.lvclass"=w171:refnum<class "Opt_Selector.lvclass">, "Instrument out"=w163:refnum<class "Instrument.lvclass">)  [unwired: 7 in]
          n83 = call-dynamic "Read State Machine.vi"("error in (no error)"=w170, "Device in"=w171) -> ("error out"=w167:errorcluster, "State Machine.lvclass"=w165:refnum<class "State Machine.lvclass">, "Device out"=w173:refnum<class "Opt_Selector.lvclass">)  [unwired: 7 in]
          n84 = call "Next State.vi"("error in (no error)"=w167, "New_State"=1, "State Machine in"=w165) -> ("error out"=w168:errorcluster, "State Machine out"=w169:refnum<class "State Machine.lvclass">)  [unwired: 7 in]
          n85 = call-dynamic "Write State Machine.vi"("error in (no error)"=w168, "State Machine.lvclass"=w169, "Device in"=w173) -> ("error out"=w174:errorcluster, "Device out"=w172:refnum<class "Opt_Selector.lvclass">)  [unwired: 7 in]
          n86 = call "Write WPROT.vi"("error in (no error)"=w174, "Opt_Selector.lvclass"=w172, "Instrument in"=w163) -> ("error out"=w161:errorcluster, "Instrument out"=w162:refnum<class "Instrument.lvclass">)  [unwired: 7 in]
          n87 = call "Write Instrument.lvclass.vi"("error in (no error)"=w161, "Instrument.lvclass"=w162, "S4ACS_GUI in"=w217) -> ("error out"=w214:errorcluster, "S4ACS_GUI out"=w203:refnum<class "S4GUI.lvclass">)  [unwired: 7 in]
          n88 = Bundle By Name(cluster=w203, "Obs_state"=w201) -> (w200:refnum<class "S4GUI.lvclass">)
        }
        frame 201 {
          # "Espera terminar a execução dos comandos ."
          n89 = call "Read Instrument.lvclass.vi"("error in (no error)"=w282, "S4ACS_GUI in"=w283) -> ("error out"=w286:errorcluster, "Instrument.lvclass"=w287:refnum<class "Instrument.lvclass">, "S4ACS_GUI out"=w284:refnum<class "S4GUI.lvclass">)  [unwired: 7 in]
          n90 = call "Read ASEL.vi"("error in (no error)"=w286, "Instrument in"=w287) -> ("error out"=w276:errorcluster, "Opt_Selector.lvclass"=w275:refnum<class "Opt_Selector.lvclass">, "Instrument out"=w285:refnum<class "Instrument.lvclass">)  [unwired: 7 in]
          n91 = call-dynamic "Read State Machine.vi"("error in (no error)"=w276, "Device in"=w275) -> ("error out"=w279:errorcluster, "State Machine.lvclass"=w280:refnum<class "State Machine.lvclass">, "Device out"=w273:refnum<class "Opt_Selector.lvclass">)  [unwired: 7 in]
          n92 = call-dynamic "Read State.vi"("error in (no error)"=w279, "State Machine in"=w280) -> ("error out"=w278:errorcluster, "State"=w269:i32, "State Machine out"=w277:refnum<class "State Machine.lvclass">)  [unwired: 7 in]
          n93 = Equal To 0?(x=w269) -> (x = 0?=w264:bool)
          n94 = call-dynamic "Write State Machine.vi"("error in (no error)"=w278, "State Machine.lvclass"=w277, "Device in"=w273) -> ("error out"=w272:errorcluster, "Device out"=w274:refnum<class "Opt_Selector.lvclass">)  [unwired: 7 in]
          n95 = call "Write ASEL.vi"("error in (no error)"=w272, "Opt_Selector.lvclass"=w274, "Instrument in"=w285) -> ("error out"=w226:errorcluster, "Instrument out"=w227:refnum<class "Instrument.lvclass">)  [unwired: 7 in]
          n96 = call "Read CALW.vi"("error in (no error)"=w226, "Instrument in"=w227) -> ("error out"=w259:errorcluster, "Opt_Selector.lvclass"=w260:refnum<class "Opt_Selector.lvclass">, "Instrument out"=w230:refnum<class "Instrument.lvclass">)  [unwired: 7 in]
          n97 = call-dynamic "Read State Machine.vi"("error in (no error)"=w259, "Device in"=w260) -> ("error out"=w256:errorcluster, "State Machine.lvclass"=w255:refnum<class "State Machine.lvclass">, "Device out"=w262:refnum<class "Opt_Selector.lvclass">)  [unwired: 7 in]
          n98 = call-dynamic "Read State.vi"("error in (no error)"=w256, "State Machine in"=w255) -> ("error out"=w257:errorcluster, "State"=w254:i32, "State Machine out"=w258:refnum<class "State Machine.lvclass">)  [unwired: 7 in]
          n99 = Equal To 0?(x=w254) -> (x = 0?=w253:bool)
          n100 = call-dynamic "Write State Machine.vi"("error in (no error)"=w257, "State Machine.lvclass"=w258, "Device in"=w262) -> ("error out"=w263:errorcluster, "Device out"=w261:refnum<class "Opt_Selector.lvclass">)  [unwired: 7 in]
          n101 = call "Write CALW.vi"("error in (no error)"=w263, "Opt_Selector.lvclass"=w261, "Instrument in"=w230) -> ("error out"=w224:errorcluster, "Instrument out"=w225:refnum<class "Instrument.lvclass">)  [unwired: 7 in]
          n102 = call "Read WPSEL.vi"("error in (no error)"=w224, "Instrument in"=w225) -> ("error out"=w247:errorcluster, "Opt_Selector.lvclass"=w246:refnum<class "Opt_Selector.lvclass">, "Instrument out"=w229:refnum<class "Instrument.lvclass">)  [unwired: 7 in]
          n103 = call-dynamic "Read State Machine.vi"("error in (no error)"=w247, "Device in"=w246) -> ("error out"=w250:errorcluster, "State Machine.lvclass"=w251:refnum<class "State Machine.lvclass">, "Device out"=w244:refnum<class "Opt_Selector.lvclass">)  [unwired: 7 in]
          n104 = call-dynamic "Read State.vi"("error in (no error)"=w250, "State Machine in"=w251) -> ("error out"=w249:errorcluster, "State"=w252:i32, "State Machine out"=w248:refnum<class "State Machine.lvclass">)  [unwired: 7 in]
          n105 = Equal To 0?(x=w252) -> (x = 0?=w232:bool)
          n106 = call-dynamic "Write State Machine.vi"("error in (no error)"=w249, "State Machine.lvclass"=w248, "Device in"=w244) -> ("error out"=w243:errorcluster, "Device out"=w245:refnum<class "Opt_Selector.lvclass">)  [unwired: 7 in]
          n107 = call "Write WPSEL.vi"("error in (no error)"=w243, "Opt_Selector.lvclass"=w245, "Instrument in"=w229) -> ("error out"=w222:errorcluster, "Instrument out"=w223:refnum<class "Instrument.lvclass">)  [unwired: 7 in]
          n108 = call "Read WPROT.vi"("error in (no error)"=w222, "Instrument in"=w223) -> ("error out"=w238:errorcluster, "Opt_Selector.lvclass"=w239:refnum<class "Opt_Selector.lvclass">, "Instrument out"=w228:refnum<class "Instrument.lvclass">)  [unwired: 7 in]
          n109 = call-dynamic "Read State Machine.vi"("error in (no error)"=w238, "Device in"=w239) -> ("error out"=w235:errorcluster, "State Machine.lvclass"=w234:refnum<class "State Machine.lvclass">, "Device out"=w241:refnum<class "Opt_Selector.lvclass">)  [unwired: 7 in]
          n110 = call-dynamic "Read State.vi"("error in (no error)"=w235, "State Machine in"=w234) -> ("error out"=w236:errorcluster, "State"=w233:i32, "State Machine out"=w237:refnum<class "State Machine.lvclass">)  [unwired: 7 in]
          n111 = Equal To 0?(x=w233) -> (x = 0?=w231:bool)
          n112 = call-dynamic "Write State Machine.vi"("error in (no error)"=w236, "State Machine.lvclass"=w237, "Device in"=w241) -> ("error out"=w242:errorcluster, "Device out"=w240:refnum<class "Opt_Selector.lvclass">)  [unwired: 7 in]
          n113 = call "Write WPROT.vi"("error in (no error)"=w242, "Opt_Selector.lvclass"=w240, "Instrument in"=w228) -> ("error out"=w220:errorcluster, "Instrument out"=w221:refnum<class "Instrument.lvclass">)  [unwired: 7 in]
          n114 = Compound Arithmetic op=AND(w264, w253, w232, w231) -> (w266:bool)
          n115 = Select(t=u32 0, s=w266, f=w265) -> (s? t:f=w268:u32)
          n116 = call "Write Instrument.lvclass.vi"("error in (no error)"=w220, "Instrument.lvclass"=w221, "S4ACS_GUI in"=w284) -> ("error out"=w281:errorcluster, "S4ACS_GUI out"=w271:refnum<class "S4GUI.lvclass">)  [unwired: 7 in]
          n117 = Bundle By Name(cluster=w271, "Obs_state"=w268) -> (w270:refnum<class "S4GUI.lvclass">)
        }
        frame 202 {
          # "Dispara o comando para o dispositivo corrente."
          n118 = call "Read Instrument.lvclass.vi"("error in (no error)"=w303, "S4ACS_GUI in"=w304) -> ("error out"=w309:errorcluster, "Instrument.lvclass"=w310:refnum<class "Instrument.lvclass">, "S4ACS_GUI out"=w306:refnum<class "S4GUI.lvclass">)  [unwired: 7 in]
          n119 = call "Read CALW.vi"("error in (no error)"=w309, "Instrument in"=w310) -> ("error out"=w296:errorcluster, "Opt_Selector.lvclass"=w295:refnum<class "Opt_Selector.lvclass">, "Instrument out"=w308:refnum<class "Instrument.lvclass">)  [unwired: 7 in]
          n120 = call-dynamic "Read State Machine.vi"("error in (no error)"=w296, "Device in"=w295) -> ("error out"=w299:errorcluster, "State Machine.lvclass"=w301:refnum<class "State Machine.lvclass">, "Device out"=w293:refnum<class "Opt_Selector.lvclass">)  [unwired: 7 in]
          n121 = call "Next State.vi"("error in (no error)"=w299, "New_State"=1, "State Machine in"=w301) -> ("error out"=w298:errorcluster, "State Machine out"=w297:refnum<class "State Machine.lvclass">)  [unwired: 7 in]
          n122 = call-dynamic "Write State Machine.vi"("error in (no error)"=w298, "State Machine.lvclass"=w297, "Device in"=w293) -> ("error out"=w292:errorcluster, "Device out"=w294:refnum<class "Opt_Selector.lvclass">)  [unwired: 7 in]
          n123 = Increment(x=w290) -> (x+1=w289:u32)
          n124 = call "Write CALW.vi"("error in (no error)"=w292, "Opt_Selector.lvclass"=w294, "Instrument in"=w308) -> ("error out"=w305:errorcluster, "Instrument out"=w307:refnum<class "Instrument.lvclass">)  [unwired: 7 in]
          n125 = call "Write Instrument.lvclass.vi"("error in (no error)"=w305, "Instrument.lvclass"=w307, "S4ACS_GUI in"=w306) -> ("error out"=w302:errorcluster, "S4ACS_GUI out"=w291:refnum<class "S4GUI.lvclass">)  [unwired: 7 in]
          n126 = Bundle By Name(cluster=w291, "Obs_state"=w289) -> (w288:refnum<class "S4GUI.lvclass">)
        }
        frame 203 {
          # "Espera terminar a execução do comando atual \nantes de ir ao proximo passo da Observação."
          n127 = call "Read Instrument.lvclass.vi"("error in (no error)"=w328, "S4ACS_GUI in"=w329) -> ("error out"=w334:errorcluster, "Instrument.lvclass"=w335:refnum<class "Instrument.lvclass">, "S4ACS_GUI out"=w331:refnum<class "S4GUI.lvclass">)  [unwired: 7 in]
          n128 = call "Read CALW.vi"("error in (no error)"=w334, "Instrument in"=w335) -> ("error out"=w322:errorcluster, "Opt_Selector.lvclass"=w321:refnum<class "Opt_Selector.lvclass">, "Instrument out"=w333:refnum<class "Instrument.lvclass">)  [unwired: 7 in]
          n129 = call-dynamic "Read State Machine.vi"("error in (no error)"=w322, "Device in"=w321) -> ("error out"=w325:errorcluster, "State Machine.lvclass"=w326:refnum<class "State Machine.lvclass">, "Device out"=w319:refnum<class "Opt_Selector.lvclass">)  [unwired: 7 in]
          n130 = Increment(x=w312) -> (x+1=w311:u32)
          n131 = call-dynamic "Read State.vi"("error in (no error)"=w325, "State Machine in"=w326) -> ("error out"=w324:errorcluster, "State"=w314:i32, "State Machine out"=w323:refnum<class "State Machine.lvclass">)  [unwired: 7 in]
          n132 = Equal To 0?(x=w314) -> (x = 0?=w315:bool)
          n133 = call-dynamic "Write State Machine.vi"("error in (no error)"=w324, "State Machine.lvclass"=w323, "Device in"=w319) -> ("error out"=w318:errorcluster, "Device out"=w320:refnum<class "Opt_Selector.lvclass">)  [unwired: 7 in]
          n134 = call "Write CALW.vi"("error in (no error)"=w318, "Opt_Selector.lvclass"=w320, "Instrument in"=w333) -> ("error out"=w330:errorcluster, "Instrument out"=w332:refnum<class "Instrument.lvclass">)  [unwired: 7 in]
          n135 = Select(t=w311, s=w315, f=w312) -> (s? t:f=w313:u32)
          n136 = call "Write Instrument.lvclass.vi"("error in (no error)"=w330, "Instrument.lvclass"=w332, "S4ACS_GUI in"=w331) -> ("error out"=w327:errorcluster, "S4ACS_GUI out"=w317:refnum<class "S4GUI.lvclass">)  [unwired: 7 in]
          n137 = Bundle By Name(cluster=w317, "Obs_state"=w313) -> (w316:refnum<class "S4GUI.lvclass">)
        }
        frame 204 {
          # "Dispara o comando para o dispositivo corrente."
          n138 = call "Read Instrument.lvclass.vi"("error in (no error)"=w351, "S4ACS_GUI in"=w352) -> ("error out"=w357:errorcluster, "Instrument.lvclass"=w358:refnum<class "Instrument.lvclass">, "S4ACS_GUI out"=w354:refnum<class "S4GUI.lvclass">)  [unwired: 7 in]
          n139 = call "Read WPSEL.vi"("error in (no error)"=w357, "Instrument in"=w358) -> ("error out"=w344:errorcluster, "Opt_Selector.lvclass"=w343:refnum<class "Opt_Selector.lvclass">, "Instrument out"=w356:refnum<class "Instrument.lvclass">)  [unwired: 7 in]
          n140 = call-dynamic "Read State Machine.vi"("error in (no error)"=w344, "Device in"=w343) -> ("error out"=w347:errorcluster, "State Machine.lvclass"=w349:refnum<class "State Machine.lvclass">, "Device out"=w341:refnum<class "Opt_Selector.lvclass">)  [unwired: 7 in]
          n141 = call "Next State.vi"("error in (no error)"=w347, "New_State"=1, "State Machine in"=w349) -> ("error out"=w346:errorcluster, "State Machine out"=w345:refnum<class "State Machine.lvclass">)  [unwired: 7 in]
          n142 = call-dynamic "Write State Machine.vi"("error in (no error)"=w346, "State Machine.lvclass"=w345, "Device in"=w341) -> ("error out"=w340:errorcluster, "Device out"=w342:refnum<class "Opt_Selector.lvclass">)  [unwired: 7 in]
          n143 = Increment(x=w338) -> (x+1=w337:u32)
          n144 = call "Write WPSEL.vi"("error in (no error)"=w340, "Opt_Selector.lvclass"=w342, "Instrument in"=w356) -> ("error out"=w353:errorcluster, "Instrument out"=w355:refnum<class "Instrument.lvclass">)  [unwired: 7 in]
          n145 = call "Write Instrument.lvclass.vi"("error in (no error)"=w353, "Instrument.lvclass"=w355, "S4ACS_GUI in"=w354) -> ("error out"=w350:errorcluster, "S4ACS_GUI out"=w339:refnum<class "S4GUI.lvclass">)  [unwired: 7 in]
          n146 = Bundle By Name(cluster=w339, "Obs_state"=w337) -> (w336:refnum<class "S4GUI.lvclass">)
        }
        frame 205 {
          # "Espera terminar a execução do comando atual \nantes de ir ao proximo passo da Observação."
          n147 = call "Read Instrument.lvclass.vi"("error in (no error)"=w376, "S4ACS_GUI in"=w377) -> ("error out"=w382:errorcluster, "Instrument.lvclass"=w383:refnum<class "Instrument.lvclass">, "S4ACS_GUI out"=w379:refnum<class "S4GUI.lvclass">)  [unwired: 7 in]
          n148 = call "Read WPSEL.vi"("error in (no error)"=w382, "Instrument in"=w383) -> ("error out"=w370:errorcluster, "Opt_Selector.lvclass"=w369:refnum<class "Opt_Selector.lvclass">, "Instrument out"=w381:refnum<class "Instrument.lvclass">)  [unwired: 7 in]
          n149 = call-dynamic "Read State Machine.vi"("error in (no error)"=w370, "Device in"=w369) -> ("error out"=w373:errorcluster, "State Machine.lvclass"=w374:refnum<class "State Machine.lvclass">, "Device out"=w367:refnum<class "Opt_Selector.lvclass">)  [unwired: 7 in]
          n150 = Increment(x=w360) -> (x+1=w359:u32)
          n151 = call-dynamic "Read State.vi"("error in (no error)"=w373, "State Machine in"=w374) -> ("error out"=w372:errorcluster, "State"=w362:i32, "State Machine out"=w371:refnum<class "State Machine.lvclass">)  [unwired: 7 in]
          n152 = Equal To 0?(x=w362) -> (x = 0?=w363:bool)
          n153 = call-dynamic "Write State Machine.vi"("error in (no error)"=w372, "State Machine.lvclass"=w371, "Device in"=w367) -> ("error out"=w366:errorcluster, "Device out"=w368:refnum<class "Opt_Selector.lvclass">)  [unwired: 7 in]
          n154 = call "Write WPSEL.vi"("error in (no error)"=w366, "Opt_Selector.lvclass"=w368, "Instrument in"=w381) -> ("error out"=w378:errorcluster, "Instrument out"=w380:refnum<class "Instrument.lvclass">)  [unwired: 7 in]
          n155 = Select(t=w359, s=w363, f=w360) -> (s? t:f=w361:u32)
          n156 = call "Write Instrument.lvclass.vi"("error in (no error)"=w378, "Instrument.lvclass"=w380, "S4ACS_GUI in"=w379) -> ("error out"=w375:errorcluster, "S4ACS_GUI out"=w365:refnum<class "S4GUI.lvclass">)  [unwired: 7 in]
          n157 = Bundle By Name(cluster=w365, "Obs_state"=w361) -> (w364:refnum<class "S4GUI.lvclass">)
        }
        frame 206 {
          # "Dispara o comando para o dispositivo corrente."
          n158 = call "Read Instrument.lvclass.vi"("error in (no error)"=w398, "S4ACS_GUI in"=w399) -> ("error out"=w404:errorcluster, "Instrument.lvclass"=w405:refnum<class "Instrument.lvclass">, "S4ACS_GUI out"=w401:refnum<class "S4GUI.lvclass">)  [unwired: 7 in]
          n159 = call "Read WPSEL.vi"("error in (no error)"=w404, "Instrument in"=w405) -> ("error out"=w392:errorcluster, "Opt_Selector.lvclass"=w393:refnum<class "Opt_Selector.lvclass">, "Instrument out"=w403:refnum<class "Instrument.lvclass">)  [unwired: 7 in]
          n160 = call "Read target name.vi"("error in (no error)"=w392, "Optics in"=w393) -> ("error out"=w386:errorcluster, "target name"=w391:string, "Optics out"=w385:refnum<class "Opt_Selector.lvclass">)  [unwired: 7 in]
          n161 = Equal?(x=w391, y="OFF") -> (x = y?=w389:bool)
          n162 = Increment(x=w395) -> (x+1=w387:u32)
          n163 = call "Write WPSEL.vi"("error in (no error)"=w386, "Opt_Selector.lvclass"=w385, "Instrument in"=w403) -> ("error out"=w400:errorcluster, "Instrument out"=w402:refnum<class "Instrument.lvclass">)  [unwired: 7 in]
          n164 = Select(t=u32 0, s=w389, f=w387) -> (s? t:f=w384:u32)
          n165 = call "Write Instrument.lvclass.vi"("error in (no error)"=w400, "Instrument.lvclass"=w402, "S4ACS_GUI in"=w401) -> ("error out"=w397:errorcluster, "S4ACS_GUI out"=w396:refnum<class "S4GUI.lvclass">)  [unwired: 7 in]
          n166 = Bundle By Name(cluster=w396, "Obs_state"=w384) -> (w394:refnum<class "S4GUI.lvclass">)
        }
        frame 207 {
          # "Dispara o comando para o dispositivo corrente."
          n167 = call "Read Instrument.lvclass.vi"("error in (no error)"=w421, "S4ACS_GUI in"=w422) -> ("error out"=w427:errorcluster, "Instrument.lvclass"=w428:refnum<class "Instrument.lvclass">, "S4ACS_GUI out"=w424:refnum<class "S4GUI.lvclass">)  [unwired: 7 in]
          n168 = call "Read WPROT.vi"("error in (no error)"=w427, "Instrument in"=w428) -> ("error out"=w414:errorcluster, "Opt_Selector.lvclass"=w413:refnum<class "Opt_Selector.lvclass">, "Instrument out"=w426:refnum<class "Instrument.lvclass">)  [unwired: 7 in]
          n169 = call-dynamic "Read State Machine.vi"("error in (no error)"=w414, "Device in"=w413) -> ("error out"=w417:errorcluster, "State Machine.lvclass"=w419:refnum<class "State Machine.lvclass">, "Device out"=w411:refnum<class "Opt_Selector.lvclass">)  [unwired: 7 in]
          n170 = call "Next State.vi"("error in (no error)"=w417, "New_State"=1, "State Machine in"=w419) -> ("error out"=w416:errorcluster, "State Machine out"=w415:refnum<class "State Machine.lvclass">)  [unwired: 7 in]
          n171 = call-dynamic "Write State Machine.vi"("error in (no error)"=w416, "State Machine.lvclass"=w415, "Device in"=w411) -> ("error out"=w410:errorcluster, "Device out"=w412:refnum<class "Opt_Selector.lvclass">)  [unwired: 7 in]
          n172 = Increment(x=w408) -> (x+1=w407:u32)
          n173 = call "Write WPROT.vi"("error in (no error)"=w410, "Opt_Selector.lvclass"=w412, "Instrument in"=w426) -> ("error out"=w423:errorcluster, "Instrument out"=w425:refnum<class "Instrument.lvclass">)  [unwired: 7 in]
          n174 = call "Write Instrument.lvclass.vi"("error in (no error)"=w423, "Instrument.lvclass"=w425, "S4ACS_GUI in"=w424) -> ("error out"=w420:errorcluster, "S4ACS_GUI out"=w409:refnum<class "S4GUI.lvclass">)  [unwired: 7 in]
          n175 = Bundle By Name(cluster=w409, "Obs_state"=w407) -> (w406:refnum<class "S4GUI.lvclass">)
        }
        frame 208 {
          # "Espera terminar a execução do comando atual \nantes de ir ao proximo passo da Observação."
          n176 = call "Read Instrument.lvclass.vi"("error in (no error)"=w446, "S4ACS_GUI in"=w447) -> ("error out"=w452:errorcluster, "Instrument.lvclass"=w453:refnum<class "Instrument.lvclass">, "S4ACS_GUI out"=w449:refnum<class "S4GUI.lvclass">)  [unwired: 7 in]
          n177 = call "Read WPROT.vi"("error in (no error)"=w452, "Instrument in"=w453) -> ("error out"=w440:errorcluster, "Opt_Selector.lvclass"=w439:refnum<class "Opt_Selector.lvclass">, "Instrument out"=w451:refnum<class "Instrument.lvclass">)  [unwired: 7 in]
          n178 = call-dynamic "Read State Machine.vi"("error in (no error)"=w440, "Device in"=w439) -> ("error out"=w443:errorcluster, "State Machine.lvclass"=w444:refnum<class "State Machine.lvclass">, "Device out"=w437:refnum<class "Opt_Selector.lvclass">)  [unwired: 7 in]
          n179 = call-dynamic "Read State.vi"("error in (no error)"=w443, "State Machine in"=w444) -> ("error out"=w442:errorcluster, "State"=w432:i32, "State Machine out"=w441:refnum<class "State Machine.lvclass">)  [unwired: 7 in]
          n180 = Equal To 0?(x=w432) -> (x = 0?=w433:bool)
          n181 = call-dynamic "Write State Machine.vi"("error in (no error)"=w442, "State Machine.lvclass"=w441, "Device in"=w437) -> ("error out"=w436:errorcluster, "Device out"=w438:refnum<class "Opt_Selector.lvclass">)  [unwired: 7 in]
          n182 = call "Write WPSEL.vi"("error in (no error)"=w436, "Opt_Selector.lvclass"=w438, "Instrument in"=w451) -> ("error out"=w448:errorcluster, "Instrument out"=w450:refnum<class "Instrument.lvclass">)  [unwired: 7 in]
          n183 = Select(t=u32 0, s=w433, f=w430) -> (s? t:f=w431:u32)
          n184 = call "Write Instrument.lvclass.vi"("error in (no error)"=w448, "Instrument.lvclass"=w450, "S4ACS_GUI in"=w449) -> ("error out"=w445:errorcluster, "S4ACS_GUI out"=w435:refnum<class "S4GUI.lvclass">)  [unwired: 7 in]
          n185 = Bundle By Name(cluster=w435, "Obs_state"=w431) -> (w434:refnum<class "S4GUI.lvclass">)
        }
        frame 220 {
          # "estado 30:\nmonta comando INIT"
          n186 = call "Read Instrument.lvclass.vi"("error in (no error)"=w500, "S4ACS_GUI in"=w501) -> ("error out"=w466:errorcluster, "Instrument.lvclass"=w467:refnum<class "Instrument.lvclass">, "S4ACS_GUI out"=w502:refnum<class "S4GUI.lvclass">)  [unwired: 7 in]
          n187 = call "Read WPSEL.vi"("error in (no error)"=w466, "Instrument in"=w467) -> ("error out"=w486:errorcluster, "Opt_Selector.lvclass"=w487:refnum<class "Opt_Selector.lvclass">, "Instrument out"=w494:refnum<class "Instrument.lvclass">)  [unwired: 7 in]
          n188 = call-dynamic "Read State Machine.vi"("error in (no error)"=w486, "Device in"=w487) -> ("error out"=w489:errorcluster, "State Machine.lvclass"=w491:refnum<class "State Machine.lvclass">, "Device out"=w488:refnum<class "Opt_Selector.lvclass">)  [unwired: 7 in]
          n189 = call "Next State.vi"("error in (no error)"=w489, "New_State"=30, "State Machine in"=w491) -> ("error out"=w458:errorcluster, "State Machine out"=w459:refnum<class "State Machine.lvclass">)  [unwired: 7 in]
          n190 = call-dynamic "Write State Machine.vi"("error in (no error)"=w458, "State Machine.lvclass"=w459, "Device in"=w488) -> ("error out"=w493:errorcluster, "Device out"=w495:refnum<class "Opt_Selector.lvclass">)  [unwired: 7 in]
          n191 = Increment(x=w492) -> (x+1=w497:u32)
          n192 = call "Write WPSEL.vi"("error in (no error)"=w493, "Opt_Selector.lvclass"=w495, "Instrument in"=w494) -> ("error out"=w464:errorcluster, "Instrument out"=w465:refnum<class "Instrument.lvclass">)  [unwired: 7 in]
          n193 = call "Read CALW.vi"("error in (no error)"=w464, "Instrument in"=w465) -> ("error out"=w477:errorcluster, "Opt_Selector.lvclass"=w478:refnum<class "Opt_Selector.lvclass">, "Instrument out"=w484:refnum<class "Instrument.lvclass">)  [unwired: 7 in]
          n194 = call-dynamic "Read State Machine.vi"("error in (no error)"=w477, "Device in"=w478) -> ("error out"=w480:errorcluster, "State Machine.lvclass"=w482:refnum<class "State Machine.lvclass">, "Device out"=w479:refnum<class "Opt_Selector.lvclass">)  [unwired: 7 in]
          n195 = call "Next State.vi"("error in (no error)"=w480, "New_State"=30, "State Machine in"=w482) -> ("error out"=w456:errorcluster, "State Machine out"=w457:refnum<class "State Machine.lvclass">)  [unwired: 7 in]
          n196 = call-dynamic "Write State Machine.vi"("error in (no error)"=w456, "State Machine.lvclass"=w457, "Device in"=w479) -> ("error out"=w483:errorcluster, "Device out"=w485:refnum<class "Opt_Selector.lvclass">)  [unwired: 7 in]
          n197 = call "Write CALW.vi"("error in (no error)"=w483, "Opt_Selector.lvclass"=w485, "Instrument in"=w484) -> ("error out"=w462:errorcluster, "Instrument out"=w463:refnum<class "Instrument.lvclass">)  [unwired: 7 in]
          n198 = call "Read GMIR.vi"("error in (no error)"=w462, "Instrument in"=w463) -> ("error out"=w468:errorcluster, "Opt_Continuous.lvclass"=w469:refnum<class "Opt_Continuous.lvclass">, "Instrument out"=w475:refnum<class "Instrument.lvclass">)  [unwired: 7 in]
          n199 = call-dynamic "Read State Machine.vi"("error in (no error)"=w468, "Device in"=w469) -> ("error out"=w471:errorcluster, "State Machine.lvclass"=w473:refnum<class "State Machine.lvclass">, "Device out"=w470:refnum<class "Opt_Continuous.lvclass">)  [unwired: 7 in]
          n200 = call "Next State.vi"("error in (no error)"=w471, "New_State"=30, "State Machine in"=w473) -> ("error out"=w454:errorcluster, "State Machine out"=w455:refnum<class "State Machine.lvclass">)  [unwired: 7 in]
          n201 = call-dynamic "Write State Machine.vi"("error in (no error)"=w454, "State Machine.lvclass"=w455, "Device in"=w470) -> ("error out"=w474:errorcluster, "Device out"=w476:refnum<class "Opt_Continuous.lvclass">)  [unwired: 7 in]
          n202 = call "Write GMIR.vi"("error in (no error)"=w474, "Opt_Continuous.lvclass"=w476, "Instrument in"=w475) -> ("error out"=w461:errorcluster, "Instrument out"=w460:refnum<class "Instrument.lvclass">)  [unwired: 7 in]
          n203 = call "Write Instrument.lvclass.vi"("error in (no error)"=w461, "Instrument.lvclass"=w460, "S4ACS_GUI in"=w502) -> ("error out"=w499:errorcluster, "S4ACS_GUI out"=w498:refnum<class "S4GUI.lvclass">)  [unwired: 7 in]
          n204 = Bundle By Name(cluster=w498, "Obs_state"=w497) -> (w496:refnum<class "S4GUI.lvclass">)
        }
        frame 221 {
          # "Espera terminar o homing de WPSEL,CALW e GMIR\nantes de seguir para o próximo estado."
          n205 = call "Read Instrument.lvclass.vi"("error in (no error)"=w531, "S4ACS_GUI in"=w532) -> ("error out"=w513:errorcluster, "Instrument.lvclass"=w514:refnum<class "Instrument.lvclass">, "S4ACS_GUI out"=w522:refnum<class "S4GUI.lvclass">)  [unwired: 7 in]
          n206 = call "Read CALW.vi"("error in (no error)"=w513, "Instrument in"=w514) -> ("error out"=w518:errorcluster, "Opt_Selector.lvclass"=w504:refnum<class "Opt_Selector.lvclass">)  [unwired: 7 in, 1 out]
          n207 = call "Read GMIR.vi"("error in (no error)"=w513, "Instrument in"=w514) -> ("error out"=w515:errorcluster, "Opt_Continuous.lvclass"=w503:refnum<class "Opt_Continuous.lvclass">)  [unwired: 7 in, 1 out]
          n208 = call "Read WPSEL.vi"("error in (no error)"=w513, "Instrument in"=w514) -> ("error out"=w528:errorcluster, "Opt_Selector.lvclass"=w527:refnum<class "Opt_Selector.lvclass">)  [unwired: 7 in, 1 out]
          n209 = call-dynamic "Read State Machine.vi"("error in (no error)"=w518, "Device in"=w504) -> ("error out"=w519:errorcluster, "State Machine.lvclass"=w520:refnum<class "State Machine.lvclass">)  [unwired: 7 in, 1 out]
          n210 = call-dynamic "Read State Machine.vi"("error in (no error)"=w515, "Device in"=w503) -> ("error out"=w516:errorcluster, "State Machine.lvclass"=w517:refnum<class "State Machine.lvclass">)  [unwired: 7 in, 1 out]
          n211 = call-dynamic "Read State Machine.vi"("error in (no error)"=w528, "Device in"=w527) -> ("error out"=w529:errorcluster, "State Machine.lvclass"=w530:refnum<class "State Machine.lvclass">)  [unwired: 7 in, 1 out]
          n212 = Increment(x=w524) -> (x+1=w523:u32)
          n213 = call-dynamic "Read State.vi"("error in (no error)"=w519, "State Machine in"=w520) -> ("error out"=w507:errorcluster, "State"=w511:i32)  [unwired: 7 in, 1 out]
          n214 = call-dynamic "Read State.vi"("error in (no error)"=w516, "State Machine in"=w517) -> ("error out"=w506:errorcluster, "State"=w510:i32)  [unwired: 7 in, 1 out]
          n215 = call-dynamic "Read State.vi"("error in (no error)"=w529, "State Machine in"=w530) -> ("error out"=w521:errorcluster, "State"=w512:i32)  [unwired: 7 in, 1 out]
          n216 = Compound Arithmetic op=ADD(w512, w511, w510) -> (w509:i32)
          n217 = Equal To 0?(x=w509) -> (x = 0?=w508:bool)
          n218 = Merge Errors(w521, w507, w506) -> (w505:errorcluster)
          n219 = Select(t=w523, s=w508, f=w524) -> (s? t:f=w525:u32)
          n220 = Bundle By Name(cluster=w522, "Obs_state"=w525) -> (w526:refnum<class "S4GUI.lvclass">)
        }
        frame 222 {
          n221 = call "Read Instrument.lvclass.vi"("error in (no error)"=w568, "S4ACS_GUI in"=w569) -> ("error out"=w539:errorcluster, "Instrument.lvclass"=w540:refnum<class "Instrument.lvclass">, "S4ACS_GUI out"=w570:refnum<class "S4GUI.lvclass">)  [unwired: 7 in]
          n222 = disable-structure shown="Enabled" {
            disable-tunnel: w540 -> [w574 w587]
            disable-tunnel: w539 -> [w573 w586]
            disable-tunnel: [w572 w587] -> w538
            disable-tunnel: [w571 w586] -> w537
            frame Disabled {
              n223 = call "Read WPROT.vi"("error in (no error)"=w573, "Instrument in"=w574) -> ("error out"=w577:errorcluster, "Opt_Selector.lvclass"=w578:refnum<class "Opt_Selector.lvclass">, "Instrument out"=w584:refnum<class "Instrument.lvclass">)  [unwired: 7 in]
              n224 = call-dynamic "Read State Machine.vi"("error in (no error)"=w577, "Device in"=w578) -> ("error out"=w580:errorcluster, "State Machine.lvclass"=w582:refnum<class "State Machine.lvclass">, "Device out"=w579:refnum<class "Opt_Selector.lvclass">)  [unwired: 7 in]
              n225 = call "Next State.vi"("error in (no error)"=w580, "New_State"=30, "State Machine in"=w582) -> ("error out"=w576:errorcluster, "State Machine out"=w575:refnum<class "State Machine.lvclass">)  [unwired: 7 in]
              n226 = call-dynamic "Write State Machine.vi"("error in (no error)"=w576, "State Machine.lvclass"=w575, "Device in"=w579) -> ("error out"=w583:errorcluster, "Device out"=w585:refnum<class "Opt_Selector.lvclass">)  [unwired: 7 in]
              n227 = call "Write WPROT.vi"("error in (no error)"=w583, "Opt_Selector.lvclass"=w585, "Instrument in"=w584) -> ("error out"=w571:errorcluster, "Instrument out"=w572:refnum<class "Instrument.lvclass">)  [unwired: 7 in]
            }
            frame Enabled {
              # "depois do homing no WPSEL, o homing do WPROT é feito automaticamente pelo ICS"
            }
          }
          n228 = call "Read ASEL.vi"("error in (no error)"=w537, "Instrument in"=w538) -> ("error out"=w554:errorcluster, "Opt_Selector.lvclass"=w555:refnum<class "Opt_Selector.lvclass">, "Instrument out"=w561:refnum<class "Instrument.lvclass">)  [unwired: 7 in]
          n229 = call-dynamic "Read State Machine.vi"("error in (no error)"=w554, "Device in"=w555) -> ("error out"=w557:errorcluster, "State Machine.lvclass"=w559:refnum<class "State Machine.lvclass">, "Device out"=w556:refnum<class "Opt_Selector.lvclass">)  [unwired: 7 in]
          n230 = call "Next State.vi"("error in (no error)"=w557, "New_State"=30, "State Machine in"=w559) -> ("error out"=w553:errorcluster, "State Machine out"=w552:refnum<class "State Machine.lvclass">)  [unwired: 7 in]
          n231 = call-dynamic "Write State Machine.vi"("error in (no error)"=w553, "State Machine.lvclass"=w552, "Device in"=w556) -> ("error out"=w560:errorcluster, "Device out"=w562:refnum<class "Opt_Selector.lvclass">)  [unwired: 7 in]
          n232 = Increment(x=w563) -> (x+1=w565:u32)
          n233 = call "Write ASEL.vi"("error in (no error)"=w560, "Opt_Selector.lvclass"=w562, "Instrument in"=w561) -> ("error out"=w535:errorcluster, "Instrument out"=w536:refnum<class "Instrument.lvclass">)  [unwired: 7 in]
          n234 = call "Read GFOC.vi"("error in (no error)"=w535, "Instrument in"=w536) -> ("error out"=w543:errorcluster, "Opt_Continuous.lvclass"=w544:refnum<class "Opt_Continuous.lvclass">, "Instrument out"=w550:refnum<class "Instrument.lvclass">)  [unwired: 7 in]
          n235 = call-dynamic "Read State Machine.vi"("error in (no error)"=w543, "Device in"=w544) -> ("error out"=w546:errorcluster, "State Machine.lvclass"=w548:refnum<class "State Machine.lvclass">, "Device out"=w545:refnum<class "Opt_Continuous.lvclass">)  [unwired: 7 in]
          n236 = call "Next State.vi"("error in (no error)"=w546, "New_State"=30, "State Machine in"=w548) -> ("error out"=w542:errorcluster, "State Machine out"=w541:refnum<class "State Machine.lvclass">)  [unwired: 7 in]
          n237 = call-dynamic "Write State Machine.vi"("error in (no error)"=w542, "State Machine.lvclass"=w541, "Device in"=w545) -> ("error out"=w549:errorcluster, "Device out"=w551:refnum<class "Opt_Continuous.lvclass">)  [unwired: 7 in]
          n238 = call "Write GFOC.vi"("error in (no error)"=w549, "Opt_Continuous.lvclass"=w551, "Instrument in"=w550) -> ("error out"=w534:errorcluster, "Instrument out"=w533:refnum<class "Instrument.lvclass">)  [unwired: 7 in]
          n239 = call "Write Instrument.lvclass.vi"("error in (no error)"=w534, "Instrument.lvclass"=w533, "S4ACS_GUI in"=w570) -> ("error out"=w567:errorcluster, "S4ACS_GUI out"=w566:refnum<class "S4GUI.lvclass">)  [unwired: 7 in]
          n240 = Bundle By Name(cluster=w566, "Obs_state"=w565) -> (w564:refnum<class "S4GUI.lvclass">)
        }
        frame 223 {
          # "Espera terminar o homing de WPROT,ASEL e GFOC\nantes de seguir para o próximo estado."
          n241 = call "Read Instrument.lvclass.vi"("error in (no error)"=w612, "S4ACS_GUI in"=w613) -> ("error out"=w598:errorcluster, "Instrument.lvclass"=w599:refnum<class "Instrument.lvclass">, "S4ACS_GUI out"=w607:refnum<class "S4GUI.lvclass">)  [unwired: 7 in]
          n242 = call "Read ASEL.vi"("error in (no error)"=w598, "Instrument in"=w599) -> ("error out"=w603:errorcluster, "Opt_Selector.lvclass"=w589:refnum<class "Opt_Selector.lvclass">)  [unwired: 7 in, 1 out]
          n243 = call "Read GFOC.vi"("error in (no error)"=w598, "Instrument in"=w599) -> ("error out"=w600:errorcluster, "Opt_Continuous.lvclass"=w588:refnum<class "Opt_Continuous.lvclass">)  [unwired: 7 in, 1 out]
          n244 = disable-structure shown="Enabled" {
            disable-tunnel: [w617 w623] -> w606
            disable-tunnel: w599 -> [w616 _]
            disable-tunnel: w598 -> [w615 w623]
            disable-tunnel: [w614 0 ("State")] -> w597
            frame Disabled {
              n245 = call "Read WPROT.vi"("error in (no error)"=w615, "Instrument in"=w616) -> ("error out"=w619:errorcluster, "Opt_Selector.lvclass"=w618:refnum<class "Opt_Selector.lvclass">)  [unwired: 7 in, 1 out]
              n246 = call-dynamic "Read State Machine.vi"("error in (no error)"=w619, "Device in"=w618) -> ("error out"=w620:errorcluster, "State Machine.lvclass"=w621:refnum<class "State Machine.lvclass">)  [unwired: 7 in, 1 out]
              n247 = call-dynamic "Read State.vi"("error in (no error)"=w620, "State Machine in"=w621) -> ("error out"=w617:errorcluster, "State"=w614:i32)  [unwired: 7 in, 1 out]
            }
            frame Enabled {
            }
          }
          n248 = call-dynamic "Read State Machine.vi"("error in (no error)"=w603, "Device in"=w589) -> ("error out"=w604:errorcluster, "State Machine.lvclass"=w605:refnum<class "State Machine.lvclass">)  [unwired: 7 in, 1 out]
          n249 = call-dynamic "Read State Machine.vi"("error in (no error)"=w600, "Device in"=w588) -> ("error out"=w601:errorcluster, "State Machine.lvclass"=w602:refnum<class "State Machine.lvclass">)  [unwired: 7 in, 1 out]
          n250 = Increment(x=w609) -> (x+1=w608:u32)
          n251 = call-dynamic "Read State.vi"("error in (no error)"=w604, "State Machine in"=w605) -> ("error out"=w592:errorcluster, "State"=w596:i32)  [unwired: 7 in, 1 out]
          n252 = call-dynamic "Read State.vi"("error in (no error)"=w601, "State Machine in"=w602) -> ("error out"=w591:errorcluster, "State"=w595:i32)  [unwired: 7 in, 1 out]
          n253 = Compound Arithmetic op=ADD(w597, w596, w595) -> (w594:i32)
          n254 = Equal To 0?(x=w594) -> (x = 0?=w593:bool)
          n255 = Merge Errors(w606, w592, w591) -> (w590:errorcluster)
          n256 = Select(t=w608, s=w593, f=w609) -> (s? t:f=w610:u32)
          n257 = Bundle By Name(cluster=w607, "Obs_state"=w610) -> (w611:refnum<class "S4GUI.lvclass">)
        }
        frame 224 {
          # "40 x 0.25 = 10s"
          # "40 x 0.25 = 10s"
          # "40 x 0.25 = 10s"
          # "Manda WPSEL para OFF, CALW para OFF e ASEL para OFF"
          n258 = call "Read Instrument.lvclass.vi"("error in (no error)"=w697, "S4ACS_GUI in"=w698) -> ("error out"=w683:errorcluster, "Instrument.lvclass"=w684:refnum<class "Instrument.lvclass">, "S4ACS_GUI out"=w699:refnum<class "S4GUI.lvclass">)  [unwired: 7 in]
          n259 = call "Read WPSEL.vi"("error in (no error)"=w683, "Instrument in"=w684) -> ("error out"=w679:errorcluster, "Opt_Selector.lvclass"=w678:refnum<class "Opt_Selector.lvclass">, "Instrument out"=w691:refnum<class "Instrument.lvclass">)  [unwired: 7 in]
          n260 = call "Write target.vi"("error in (no error)"=w679, "target"=80.0, "Optics in"=w678) -> ("error out"=w682:errorcluster, "Optics out"=w677:refnum<class "Opt_Selector.lvclass">)  [unwired: 7 in]
          n261 = call "Write target name.vi"("error in (no error)"=w682, "target name"="OFF", "Optics in"=w677) -> ("error out"=w675:errorcluster, "Optics out"=w676:refnum<class "Opt_Selector.lvclass">)  [unwired: 7 in]
          n262 = call-dynamic "Read State Machine.vi"("error in (no error)"=w675, "Device in"=w676) -> ("error out"=w686:errorcluster, "State Machine.lvclass"=w688:refnum<class "State Machine.lvclass">, "Device out"=w685:refnum<class "Opt_Selector.lvclass">)  [unwired: 7 in]
          n263 = call "Next State.vi"("error in (no error)"=w686, "New_State"=1, "State Machine in"=w688) -> ("error out"=w636:errorcluster, "State Machine out"=w638:refnum<class "State Machine.lvclass">)  [unwired: 7 in]
          n264 = call-dynamic "Write Timer.vi"("error in (no error)"=w636, "Timer"=u32 40, "State Machine in"=w638) -> ("error out"=w635:errorcluster, "State Machine out"=w637:refnum<class "State Machine.lvclass">)  [unwired: 7 in]
          n265 = call-dynamic "Write State Machine.vi"("error in (no error)"=w635, "State Machine.lvclass"=w637, "Device in"=w685) -> ("error out"=w690:errorcluster, "Device out"=w692:refnum<class "Opt_Selector.lvclass">)  [unwired: 7 in]
          n266 = Increment(x=w689) -> (x+1=w694:u32)
          n267 = call "Write WPSEL.vi"("error in (no error)"=w690, "Opt_Selector.lvclass"=w692, "Instrument in"=w691) -> ("error out"=w650:errorcluster, "Instrument out"=w649:refnum<class "Instrument.lvclass">)  [unwired: 7 in]
          n268 = call "Read CALW.vi"("error in (no error)"=w650, "Instrument in"=w649) -> ("error out"=w666:errorcluster, "Opt_Selector.lvclass"=w648:refnum<class "Opt_Selector.lvclass">, "Instrument out"=w646:refnum<class "Instrument.lvclass">)  [unwired: 7 in]
          n269 = call "Write target.vi"("error in (no error)"=w666, "target"=0.0, "Optics in"=w648) -> ("error out"=w669:errorcluster, "Optics out"=w665:refnum<class "Opt_Selector.lvclass">)  [unwired: 7 in]
          n270 = call "Write target name.vi"("error in (no error)"=w669, "target name"="OFF", "Optics in"=w665) -> ("error out"=w663:errorcluster, "Optics out"=w664:refnum<class "Opt_Selector.lvclass">)  [unwired: 7 in]
          n271 = call-dynamic "Read State Machine.vi"("error in (no error)"=w663, "Device in"=w664) -> ("error out"=w671:errorcluster, "State Machine.lvclass"=w673:refnum<class "State Machine.lvclass">, "Device out"=w670:refnum<class "Opt_Selector.lvclass">)  [unwired: 7 in]
          n272 = call "Next State.vi"("error in (no error)"=w671, "New_State"=1, "State Machine in"=w673) -> ("error out"=w632:errorcluster, "State Machine out"=w633:refnum<class "State Machine.lvclass">)  [unwired: 7 in]
          n273 = call-dynamic "Write Timer.vi"("error in (no error)"=w632, "Timer"=u32 40, "State Machine in"=w633) -> ("error out"=w631:errorcluster, "State Machine out"=w630:refnum<class "State Machine.lvclass">)  [unwired: 7 in]
          n274 = call-dynamic "Write State Machine.vi"("error in (no error)"=w631, "State Machine.lvclass"=w630, "Device in"=w670) -> ("error out"=w674:errorcluster, "Device out"=w647:refnum<class "Opt_Selector.lvclass">)  [unwired: 7 in]
          n275 = call "Write CALW.vi"("error in (no error)"=w674, "Opt_Selector.lvclass"=w647, "Instrument in"=w646) -> ("error out"=w645:errorcluster, "Instrument out"=w644:refnum<class "Instrument.lvclass">)  [unwired: 7 in]
          n276 = call "Read ASEL.vi"("error in (no error)"=w645, "Instrument in"=w644) -> ("error out"=w654:errorcluster, "Opt_Selector.lvclass"=w643:refnum<class "Opt_Selector.lvclass">, "Instrument out"=w641:refnum<class "Instrument.lvclass">)  [unwired: 7 in]
          n277 = call "Write target.vi"("error in (no error)"=w654, "target"=0.0, "Optics in"=w643) -> ("error out"=w657:errorcluster, "Optics out"=w653:refnum<class "Opt_Selector.lvclass">)  [unwired: 7 in]
          n278 = call "Write target name.vi"("error in (no error)"=w657, "target name"="OFF", "Optics in"=w653) -> ("error out"=w651:errorcluster, "Optics out"=w652:refnum<class "Opt_Selector.lvclass">)  [unwired: 7 in]
          n279 = call-dynamic "Read State Machine.vi"("error in (no error)"=w651, "Device in"=w652) -> ("error out"=w659:errorcluster, "State Machine.lvclass"=w661:refnum<class "State Machine.lvclass">, "Device out"=w658:refnum<class "Opt_Selector.lvclass">)  [unwired: 7 in]
          n280 = call "Next State.vi"("error in (no error)"=w659, "New_State"=1, "State Machine in"=w661) -> ("error out"=w626:errorcluster, "State Machine out"=w627:refnum<class "State Machine.lvclass">)  [unwired: 7 in]
          n281 = call-dynamic "Write Timer.vi"("error in (no error)"=w626, "Timer"=u32 40, "State Machine in"=w627) -> ("error out"=w625:errorcluster, "State Machine out"=w624:refnum<class "State Machine.lvclass">)  [unwired: 7 in]
          n282 = call-dynamic "Write State Machine.vi"("error in (no error)"=w625, "State Machine.lvclass"=w624, "Device in"=w658) -> ("error out"=w662:errorcluster, "Device out"=w642:refnum<class "Opt_Selector.lvclass">)  [unwired: 7 in]
          n283 = call "Write ASEL.vi"("error in (no error)"=w662, "Opt_Selector.lvclass"=w642, "Instrument in"=w641) -> ("error out"=w639:errorcluster, "Instrument out"=w640:refnum<class "Instrument.lvclass">)  [unwired: 7 in]
          n284 = call "Write Instrument.lvclass.vi"("error in (no error)"=w639, "Instrument.lvclass"=w640, "S4ACS_GUI in"=w699) -> ("error out"=w696:errorcluster, "S4ACS_GUI out"=w695:refnum<class "S4GUI.lvclass">)  [unwired: 7 in]
          n285 = Bundle By Name(cluster=w695, "Obs_state"=w694) -> (w693:refnum<class "S4GUI.lvclass">)
        }
        frame 225 {
          # "Espera terminar o movimento de WPSEL, ASEL e CALW para CLEAR."
          n286 = call "Read Instrument.lvclass.vi"("error in (no error)"=w728, "S4ACS_GUI in"=w729) -> ("error out"=w711:errorcluster, "Instrument.lvclass"=w712:refnum<class "Instrument.lvclass">, "S4ACS_GUI out"=w720:refnum<class "S4GUI.lvclass">)  [unwired: 7 in]
          n287 = call "Read ASEL.vi"("error in (no error)"=w711, "Instrument in"=w712) -> ("error out"=w716:errorcluster, "Opt_Selector.lvclass"=w702:refnum<class "Opt_Selector.lvclass">)  [unwired: 7 in, 1 out]
          n288 = call "Read CALW.vi"("error in (no error)"=w711, "Instrument in"=w712) -> ("error out"=w713:errorcluster, "Opt_Selector.lvclass"=w701:refnum<class "Opt_Selector.lvclass">)  [unwired: 7 in, 1 out]
          n289 = call "Read WPSEL.vi"("error in (no error)"=w711, "Instrument in"=w712) -> ("error out"=w725:errorcluster, "Opt_Selector.lvclass"=w724:refnum<class "Opt_Selector.lvclass">)  [unwired: 7 in, 1 out]
          n290 = call-dynamic "Read State Machine.vi"("error in (no error)"=w716, "Device in"=w702) -> ("error out"=w717:errorcluster, "State Machine.lvclass"=w718:refnum<class "State Machine.lvclass">)  [unwired: 7 in, 1 out]
          n291 = call-dynamic "Read State Machine.vi"("error in (no error)"=w713, "Device in"=w701) -> ("error out"=w714:errorcluster, "State Machine.lvclass"=w715:refnum<class "State Machine.lvclass">)  [unwired: 7 in, 1 out]
          n292 = call-dynamic "Read State Machine.vi"("error in (no error)"=w725, "Device in"=w724) -> ("error out"=w726:errorcluster, "State Machine.lvclass"=w727:refnum<class "State Machine.lvclass">)  [unwired: 7 in, 1 out]
          n293 = call-dynamic "Read State.vi"("error in (no error)"=w717, "State Machine in"=w718) -> ("error out"=w705:errorcluster, "State"=w709:i32)  [unwired: 7 in, 1 out]
          n294 = call-dynamic "Read State.vi"("error in (no error)"=w714, "State Machine in"=w715) -> ("error out"=w704:errorcluster, "State"=w708:i32)  [unwired: 7 in, 1 out]
          n295 = call-dynamic "Read State.vi"("error in (no error)"=w726, "State Machine in"=w727) -> ("error out"=w719:errorcluster, "State"=w710:i32)  [unwired: 7 in, 1 out]
          n296 = Compound Arithmetic op=ADD(w710, w709, w708) -> (w707:i32)
          n297 = Equal To 0?(x=w707) -> (x = 0?=w706:bool)
          n298 = Merge Errors(w719, w705, w704) -> (w703:errorcluster)
          n299 = Select(t=u32 0, s=w706, f=w721) -> (s? t:f=w722:u32)
          n300 = Bundle By Name(cluster=w720, "Obs_state"=w722) -> (w723:refnum<class "S4GUI.lvclass">)
        }
        frame 251 {
          n301 = flat-sequence {
            tunnel: w748 -> [w857]
            tunnel: [w857] -> w747
            frame #0 {
              n302 = Tick Count (ms)() -> (millisecond timer value=→"time3":u32)
            }
          }
          n303 = call-dynamic "Read AcquisitionA.vi"("error in (no error)"=w747, "S4ACS_GUI in"=w773) -> ("error out"=w770:errorcluster, "Acquisition.lvclass"=w771:refnum<class "Acquisition.lvclass">, "S4ACS_GUI out"=w775:refnum<class "S4GUI.lvclass">)  [unwired: 7 in]
          n304 = call "Read connection.vi"("error in (no error)"=w770, "Server in"=w771) -> ("error out"=w769:errorcluster, "connection"=w745:bool, "Server out"=w768:refnum<class "Acquisition.lvclass">)  [unwired: 7 in]
          n305 = case shown="True" w745 {
            tunnel: [w838 w856] -> w776
            tunnel: [w837 w855] -> w774
            tunnel: w769 -> [w837 w854]
            tunnel: w768 -> [w838 w853]
            frame False {
            }
            frame True {
              # "configura o canal,\nmas não dispara\na exposicao."
              n306 = call-dynamic "Read Channel.vi"("error in (no error)"=w854, "Acquisition in"=w853) -> ("error out"=w843:errorcluster, "Channel.lvclass"=w845:refnum<class "Channel.lvclass">, "Acquisition out"=w852:refnum<class "Acquisition.lvclass">)  [unwired: 7 in]
              n307 = call-dynamic "Write expose.vi"("error in (no error)"=w843, "expose"=FALSE, "Channel in"=w845) -> ("error out"=w842:errorcluster, "Channel out"=w844:refnum<class "Channel.lvclass">)  [unwired: 7 in]
              n308 = call-dynamic "Read State Machine.vi"("error in (no error)"=w842, "Device in"=w844) -> ("error out"=w849:errorcluster, "State Machine.lvclass"=w851:refnum<class "State Machine.lvclass">, "Device out"=w847:refnum<class "Channel.lvclass">)  [unwired: 7 in]
              n309 = call "Next State.vi"("error in (no error)"=w849, "New_State"=1, "State Machine in"=w851) -> ("error out"=w839:errorcluster, "State Machine out"=w840:refnum<class "State Machine.lvclass">)  [unwired: 7 in]
              n310 = call-dynamic "Write State Machine.vi"("error in (no error)"=w839, "State Machine.lvclass"=w840, "Device in"=w847) -> ("error out"=w846:errorcluster, "Device out"=w848:refnum<class "Channel.lvclass">)  [unwired: 7 in]
              n311 = call-dynamic "Write Channel.vi"("error in (no error)"=w846, "Channel.lvclass"=w848, "Acquisition in"=w852) -> ("error out"=w855:errorcluster, "Acquisition out"=w856:refnum<class "Acquisition.lvclass">)  [unwired: 7 in]
            }
          }
          n312 = Increment(x=w767) -> (x+1=w766:u32)
          n313 = call-dynamic "Write AcquisitionA.vi"("error in (no error)"=w774, "Acquisition.lvclass"=w776, "S4ACS_GUI in"=w775) -> ("error out"=w762:errorcluster, "S4ACS_GUI out"=w761:refnum<class "S4GUI.lvclass">)  [unwired: 7 in]
          n314 = call "Read AcquisitionB.vi"("error in (no error)"=w762, "S4ACS_GUI in"=w761) -> ("error out"=w763:errorcluster, "Acquisition.lvclass"=w764:refnum<class "Acquisition.lvclass">, "S4ACS_GUI out"=w765:refnum<class "S4GUI.lvclass">)  [unwired: 7 in]
          n315 = call "Read connection.vi"("error in (no error)"=w763, "Server in"=w764) -> ("error out"=w743:errorcluster, "connection"=w742:bool, "Server out"=w744:refnum<class "Acquisition.lvclass">)  [unwired: 7 in]
          n316 = case shown="True" w742 {
            tunnel: [w818 w836] -> w741
            tunnel: [w817 w835] -> w740
            tunnel: w743 -> [w817 w834]
            tunnel: w744 -> [w818 w833]
            frame False {
            }
            frame True {
              # "configura o canal,\nmas não dispara\na exposicao."
              n317 = call-dynamic "Read Channel.vi"("error in (no error)"=w834, "Acquisition in"=w833) -> ("error out"=w823:errorcluster, "Channel.lvclass"=w825:refnum<class "Channel.lvclass">, "Acquisition out"=w832:refnum<class "Acquisition.lvclass">)  [unwired: 7 in]
              n318 = call-dynamic "Write expose.vi"("error in (no error)"=w823, "expose"=FALSE, "Channel in"=w825) -> ("error out"=w822:errorcluster, "Channel out"=w824:refnum<class "Channel.lvclass">)  [unwired: 7 in]
              n319 = call-dynamic "Read State Machine.vi"("error in (no error)"=w822, "Device in"=w824) -> ("error out"=w829:errorcluster, "State Machine.lvclass"=w831:refnum<class "State Machine.lvclass">, "Device out"=w827:refnum<class "Channel.lvclass">)  [unwired: 7 in]
              n320 = call "Next State.vi"("error in (no error)"=w829, "New_State"=1, "State Machine in"=w831) -> ("error out"=w819:errorcluster, "State Machine out"=w820:refnum<class "State Machine.lvclass">)  [unwired: 7 in]
              n321 = call-dynamic "Write State Machine.vi"("error in (no error)"=w819, "State Machine.lvclass"=w820, "Device in"=w827) -> ("error out"=w826:errorcluster, "Device out"=w828:refnum<class "Channel.lvclass">)  [unwired: 7 in]
              n322 = call-dynamic "Write Channel.vi"("error in (no error)"=w826, "Channel.lvclass"=w828, "Acquisition in"=w832) -> ("error out"=w835:errorcluster, "Acquisition out"=w836:refnum<class "Acquisition.lvclass">)  [unwired: 7 in]
            }
          }
          n323 = call "Write AcquisitionB.vi"("error in (no error)"=w740, "Acquisition.lvclass"=w741, "S4ACS_GUI in"=w765) -> ("error out"=w754:errorcluster, "S4ACS_GUI out"=w753:refnum<class "S4GUI.lvclass">)  [unwired: 7 in]
          n324 = call-dynamic "Read AcquisitionC.vi"("error in (no error)"=w754, "S4ACS_GUI in"=w753) -> ("error out"=w758:errorcluster, "Acquisition.lvclass"=w759:refnum<class "Acquisition.lvclass">, "S4ACS_GUI out"=w760:refnum<class "S4GUI.lvclass">)  [unwired: 7 in]
          n325 = call "Read connection.vi"("error in (no error)"=w758, "Server in"=w759) -> ("error out"=w737:errorcluster, "connection"=w738:bool, "Server out"=w739:refnum<class "Acquisition.lvclass">)  [unwired: 7 in]
          n326 = case shown="True" w738 {
            tunnel: [w798 w816] -> w736
            tunnel: [w797 w815] -> w735
            tunnel: w737 -> [w797 w814]
            tunnel: w739 -> [w798 w813]
            frame False {
            }
            frame True {
              # "configura o canal,\nmas não dispara\na exposicao."
              n327 = call-dynamic "Read Channel.vi"("error in (no error)"=w814, "Acquisition in"=w813) -> ("error out"=w803:errorcluster, "Channel.lvclass"=w805:refnum<class "Channel.lvclass">, "Acquisition out"=w812:refnum<class "Acquisition.lvclass">)  [unwired: 7 in]
              n328 = call-dynamic "Write expose.vi"("error in (no error)"=w803, "expose"=FALSE, "Channel in"=w805) -> ("error out"=w802:errorcluster, "Channel out"=w804:refnum<class "Channel.lvclass">)  [unwired: 7 in]
              n329 = call-dynamic "Read State Machine.vi"("error in (no error)"=w802, "Device in"=w804) -> ("error out"=w809:errorcluster, "State Machine.lvclass"=w811:refnum<class "State Machine.lvclass">, "Device out"=w807:refnum<class "Channel.lvclass">)  [unwired: 7 in]
              n330 = call "Next State.vi"("error in (no error)"=w809, "New_State"=1, "State Machine in"=w811) -> ("error out"=w799:errorcluster, "State Machine out"=w800:refnum<class "State Machine.lvclass">)  [unwired: 7 in]
              n331 = call-dynamic "Write State Machine.vi"("error in (no error)"=w799, "State Machine.lvclass"=w800, "Device in"=w807) -> ("error out"=w806:errorcluster, "Device out"=w808:refnum<class "Channel.lvclass">)  [unwired: 7 in]
              n332 = call-dynamic "Write Channel.vi"("error in (no error)"=w806, "Channel.lvclass"=w808, "Acquisition in"=w812) -> ("error out"=w815:errorcluster, "Acquisition out"=w816:refnum<class "Acquisition.lvclass">)  [unwired: 7 in]
            }
          }
          n333 = call-dynamic "Write AcquisitionC.vi"("error in (no error)"=w735, "Acquisition.lvclass"=w736, "S4ACS_GUI in"=w760) -> ("error out"=w752:errorcluster, "S4ACS_GUI out"=w751:refnum<class "S4GUI.lvclass">)  [unwired: 7 in]
          n334 = call-dynamic "Read AcquisitionD.vi"("error in (no error)"=w752, "S4ACS_GUI in"=w751) -> ("error out"=w755:errorcluster, "Acquisition.lvclass"=w756:refnum<class "Acquisition.lvclass">, "S4ACS_GUI out"=w757:refnum<class "S4GUI.lvclass">)  [unwired: 7 in]
          n335 = call "Read connection.vi"("error in (no error)"=w755, "Server in"=w756) -> ("error out"=w732:errorcluster, "connection"=w734:bool, "Server out"=w733:refnum<class "Acquisition.lvclass">)  [unwired: 7 in]
          n336 = case shown="True" w734 {
            tunnel: [w778 w796] -> w731
            tunnel: [w777 w795] -> w730
            tunnel: w732 -> [w777 w794]
            tunnel: w733 -> [w778 w793]
            frame False {
            }
            frame True {
              # "configura o canal,\nmas não dispara\na exposicao."
              n337 = call-dynamic "Read Channel.vi"("error in (no error)"=w794, "Acquisition in"=w793) -> ("error out"=w783:errorcluster, "Channel.lvclass"=w785:refnum<class "Channel.lvclass">, "Acquisition out"=w792:refnum<class "Acquisition.lvclass">)  [unwired: 7 in]
              n338 = call-dynamic "Write expose.vi"("error in (no error)"=w783, "expose"=FALSE, "Channel in"=w785) -> ("error out"=w782:errorcluster, "Channel out"=w784:refnum<class "Channel.lvclass">)  [unwired: 7 in]
              n339 = call-dynamic "Read State Machine.vi"("error in (no error)"=w782, "Device in"=w784) -> ("error out"=w789:errorcluster, "State Machine.lvclass"=w791:refnum<class "State Machine.lvclass">, "Device out"=w787:refnum<class "Channel.lvclass">)  [unwired: 7 in]
              n340 = call "Next State.vi"("error in (no error)"=w789, "New_State"=1, "State Machine in"=w791) -> ("error out"=w779:errorcluster, "State Machine out"=w780:refnum<class "State Machine.lvclass">)  [unwired: 7 in]
              n341 = call-dynamic "Write State Machine.vi"("error in (no error)"=w779, "State Machine.lvclass"=w780, "Device in"=w787) -> ("error out"=w786:errorcluster, "Device out"=w788:refnum<class "Channel.lvclass">)  [unwired: 7 in]
              n342 = call-dynamic "Write Channel.vi"("error in (no error)"=w786, "Channel.lvclass"=w788, "Acquisition in"=w792) -> ("error out"=w795:errorcluster, "Acquisition out"=w796:refnum<class "Acquisition.lvclass">)  [unwired: 7 in]
            }
          }
          n343 = call-dynamic "Write AcquisitionD.vi"("error in (no error)"=w730, "Acquisition.lvclass"=w731, "S4ACS_GUI in"=w757) -> ("error out"=w750:errorcluster, "S4ACS_GUI out"=w749:refnum<class "S4GUI.lvclass">)  [unwired: 7 in]
          n344 = Bundle By Name(cluster=w749, "Obs_state"=w766, "cyclesDone"=u32 0) -> (w772:refnum<class "S4GUI.lvclass">)
        }
        frame 252 {
          # "Espera terminar a execução da preparação\ndos 4 canais antes de ir ao proximo passo \nda Observação."
          n345 = flat-sequence {
            tunnel: w890 -> [w984]
            tunnel: [w984] -> w889
            frame #0 {
              n346 = Tick Count (ms)() -> (millisecond timer value=→"time4":u32)
            }
          }
          n347 = call-dynamic "Read AcquisitionA.vi"("error in (no error)"=w889, "S4ACS_GUI in"=w908) -> ("error out"=w887:errorcluster, "Acquisition.lvclass"=w888:refnum<class "Acquisition.lvclass">, "S4ACS_GUI out"=w910:refnum<class "S4GUI.lvclass">)  [unwired: 7 in]
          n348 = call "Read connection.vi"("error in (no error)"=w887, "Server in"=w888) -> ("error out"=w885:errorcluster, "connection"=w884:bool, "Server out"=w886:refnum<class "Acquisition.lvclass">)  [unwired: 7 in]
          n349 = case shown="True" w884 {
            tunnel: w886 -> [w967 w983]
            tunnel: w885 -> [w966 w982]
            tunnel: [w967 w980] -> w911
            tunnel: [w966 w979] -> w909
            tunnel: [0 ("State") w969] -> w901
            frame False {
            }
            frame True {
              n350 = call-dynamic "Read Channel.vi"("error in (no error)"=w982, "Acquisition in"=w983) -> ("error out"=w978:errorcluster, "Channel.lvclass"=w977:refnum<class "Channel.lvclass">, "Acquisition out"=w981:refnum<class "Acquisition.lvclass">)  [unwired: 7 in]
              n351 = call-dynamic "Read State Machine.vi"("error in (no error)"=w978, "Device in"=w977) -> ("error out"=w971:errorcluster, "State Machine.lvclass"=w973:refnum<class "State Machine.lvclass">, "Device out"=w975:refnum<class "Channel.lvclass">)  [unwired: 7 in]
              n352 = call-dynamic "Read State.vi"("error in (no error)"=w971, "State Machine in"=w973) -> ("error out"=w970:errorcluster, "State"=w969:i32, "State Machine out"=w972:refnum<class "State Machine.lvclass">)  [unwired: 7 in]
              n353 = call-dynamic "Write State Machine.vi"("error in (no error)"=w970, "State Machine.lvclass"=w972, "Device in"=w975) -> ("error out"=w974:errorcluster, "Device out"=w976:refnum<class "Channel.lvclass">)  [unwired: 7 in]
              n354 = call-dynamic "Write Channel.vi"("error in (no error)"=w974, "Channel.lvclass"=w976, "Acquisition in"=w981) -> ("error out"=w979:errorcluster, "Acquisition out"=w980:refnum<class "Acquisition.lvclass">)  [unwired: 7 in]
            }
          }
          n355 = call-dynamic "Write AcquisitionA.vi"("error in (no error)"=w909, "Acquisition.lvclass"=w911, "S4ACS_GUI in"=w910) -> ("error out"=w898:errorcluster, "S4ACS_GUI out"=w897:refnum<class "S4GUI.lvclass">)  [unwired: 7 in]
          n356 = call "Read AcquisitionB.vi"("error in (no error)"=w898, "S4ACS_GUI in"=w897) -> ("error out"=w879:errorcluster, "Acquisition.lvclass"=w882:refnum<class "Acquisition.lvclass">, "S4ACS_GUI out"=w883:refnum<class "S4GUI.lvclass">)  [unwired: 7 in]
          n357 = call "Read connection.vi"("error in (no error)"=w879, "Server in"=w882) -> ("error out"=w878:errorcluster, "connection"=w880:bool, "Server out"=w881:refnum<class "Acquisition.lvclass">)  [unwired: 7 in]
          n358 = case shown="True" w880 {
            tunnel: w881 -> [w949 w965]
            tunnel: w878 -> [w948 w964]
            tunnel: [w949 w962] -> w877
            tunnel: [w948 w961] -> w876
            tunnel: [0 ("State") w951] -> w875
            frame False {
            }
            frame True {
              n359 = call-dynamic "Read Channel.vi"("error in (no error)"=w964, "Acquisition in"=w965) -> ("error out"=w960:errorcluster, "Channel.lvclass"=w959:refnum<class "Channel.lvclass">, "Acquisition out"=w963:refnum<class "Acquisition.lvclass">)  [unwired: 7 in]
              n360 = call-dynamic "Read State Machine.vi"("error in (no error)"=w960, "Device in"=w959) -> ("error out"=w953:errorcluster, "State Machine.lvclass"=w955:refnum<class "State Machine.lvclass">, "Device out"=w957:refnum<class "Channel.lvclass">)  [unwired: 7 in]
              n361 = call-dynamic "Read State.vi"("error in (no error)"=w953, "State Machine in"=w955) -> ("error out"=w952:errorcluster, "State"=w951:i32, "State Machine out"=w954:refnum<class "State Machine.lvclass">)  [unwired: 7 in]
              n362 = call-dynamic "Write State Machine.vi"("error in (no error)"=w952, "State Machine.lvclass"=w954, "Device in"=w957) -> ("error out"=w956:errorcluster, "Device out"=w958:refnum<class "Channel.lvclass">)  [unwired: 7 in]
              n363 = call-dynamic "Write Channel.vi"("error in (no error)"=w956, "Channel.lvclass"=w958, "Acquisition in"=w963) -> ("error out"=w961:errorcluster, "Acquisition out"=w962:refnum<class "Acquisition.lvclass">)  [unwired: 7 in]
            }
          }
          n364 = call "Write AcquisitionB.vi"("error in (no error)"=w876, "Acquisition.lvclass"=w877, "S4ACS_GUI in"=w883) -> ("error out"=w896:errorcluster, "S4ACS_GUI out"=w895:refnum<class "S4GUI.lvclass">)  [unwired: 7 in]
          n365 = call-dynamic "Read AcquisitionC.vi"("error in (no error)"=w896, "S4ACS_GUI in"=w895) -> ("error out"=w873:errorcluster, "Acquisition.lvclass"=w874:refnum<class "Acquisition.lvclass">, "S4ACS_GUI out"=w903:refnum<class "S4GUI.lvclass">)  [unwired: 7 in]
          n366 = call "Read connection.vi"("error in (no error)"=w873, "Server in"=w874) -> ("error out"=w872:errorcluster, "connection"=w870:bool, "Server out"=w871:refnum<class "Acquisition.lvclass">)  [unwired: 7 in]
          n367 = case shown="True" w870 {
            tunnel: w871 -> [w931 w947]
            tunnel: w872 -> [w930 w946]
            tunnel: [w931 w944] -> w869
            tunnel: [w930 w943] -> w868
            tunnel: [0 ("State") w933] -> w867
            frame False {
            }
            frame True {
              n368 = call-dynamic "Read Channel.vi"("error in (no error)"=w946, "Acquisition in"=w947) -> ("error out"=w942:errorcluster, "Channel.lvclass"=w941:refnum<class "Channel.lvclass">, "Acquisition out"=w945:refnum<class "Acquisition.lvclass">)  [unwired: 7 in]
              n369 = call-dynamic "Read State Machine.vi"("error in (no error)"=w942, "Device in"=w941) -> ("error out"=w935:errorcluster, "State Machine.lvclass"=w937:refnum<class "State Machine.lvclass">, "Device out"=w939:refnum<class "Channel.lvclass">)  [unwired: 7 in]
              n370 = call-dynamic "Read State.vi"("error in (no error)"=w935, "State Machine in"=w937) -> ("error out"=w934:errorcluster, "State"=w933:i32, "State Machine out"=w936:refnum<class "State Machine.lvclass">)  [unwired: 7 in]
              n371 = call-dynamic "Write State Machine.vi"("error in (no error)"=w934, "State Machine.lvclass"=w936, "Device in"=w939) -> ("error out"=w938:errorcluster, "Device out"=w940:refnum<class "Channel.lvclass">)  [unwired: 7 in]
              n372 = call-dynamic "Write Channel.vi"("error in (no error)"=w938, "Channel.lvclass"=w940, "Acquisition in"=w945) -> ("error out"=w943:errorcluster, "Acquisition out"=w944:refnum<class "Acquisition.lvclass">)  [unwired: 7 in]
            }
          }
          n373 = call-dynamic "Write AcquisitionC.vi"("error in (no error)"=w868, "Acquisition.lvclass"=w869, "S4ACS_GUI in"=w903) -> ("error out"=w894:errorcluster, "S4ACS_GUI out"=w893:refnum<class "S4GUI.lvclass">)  [unwired: 7 in]
          n374 = call-dynamic "Read AcquisitionD.vi"("error in (no error)"=w894, "S4ACS_GUI in"=w893) -> ("error out"=w864:errorcluster, "Acquisition.lvclass"=w866:refnum<class "Acquisition.lvclass">, "S4ACS_GUI out"=w902:refnum<class "S4GUI.lvclass">)  [unwired: 7 in]
          n375 = call "Read connection.vi"("error in (no error)"=w864, "Server in"=w866) -> ("error out"=w863:errorcluster, "connection"=w862:bool, "Server out"=w865:refnum<class "Acquisition.lvclass">)  [unwired: 7 in]
          n376 = case shown="True" w862 {
            tunnel: w865 -> [w913 w929]
            tunnel: w863 -> [w912 w928]
            tunnel: [w913 w926] -> w861
            tunnel: [w912 w925] -> w860
            tunnel: [0 ("State") w915] -> w859
            frame False {
            }
            frame True {
              n377 = call-dynamic "Read Channel.vi"("error in (no error)"=w928, "Acquisition in"=w929) -> ("error out"=w924:errorcluster, "Channel.lvclass"=w923:refnum<class "Channel.lvclass">, "Acquisition out"=w927:refnum<class "Acquisition.lvclass">)  [unwired: 7 in]
              n378 = call-dynamic "Read State Machine.vi"("error in (no error)"=w924, "Device in"=w923) -> ("error out"=w917:errorcluster, "State Machine.lvclass"=w919:refnum<class "State Machine.lvclass">, "Device out"=w921:refnum<class "Channel.lvclass">)  [unwired: 7 in]
              n379 = call-dynamic "Read State.vi"("error in (no error)"=w917, "State Machine in"=w919) -> ("error out"=w916:errorcluster, "State"=w915:i32, "State Machine out"=w918:refnum<class "State Machine.lvclass">)  [unwired: 7 in]
              n380 = call-dynamic "Write State Machine.vi"("error in (no error)"=w916, "State Machine.lvclass"=w918, "Device in"=w921) -> ("error out"=w920:errorcluster, "Device out"=w922:refnum<class "Channel.lvclass">)  [unwired: 7 in]
              n381 = call-dynamic "Write Channel.vi"("error in (no error)"=w920, "Channel.lvclass"=w922, "Acquisition in"=w927) -> ("error out"=w925:errorcluster, "Acquisition out"=w926:refnum<class "Acquisition.lvclass">)  [unwired: 7 in]
            }
          }
          n382 = call-dynamic "Write AcquisitionD.vi"("error in (no error)"=w860, "Acquisition.lvclass"=w861, "S4ACS_GUI in"=w902) -> ("error out"=w892:errorcluster, "S4ACS_GUI out"=w891:refnum<class "S4GUI.lvclass">)  [unwired: 7 in]
          n383 = Compound Arithmetic op=ADD(w901, w875, w867, w859) -> (w900:i32)
          n384 = Equal To 0?(x=w900) -> (x = 0?=w899:bool)
          n385 = Select(t=u32 299, s=w899, f=w904) -> (s? t:f=w906:u32)
          n386 = Bundle By Name(cluster=w891, "Obs_state"=w906) -> (w907:refnum<class "S4GUI.lvclass">)
        }
        frame 253 {
          # "Sem SyncBox, \ntrigger mode = 0 (internal)\nCom SyncBox\ntrigger mode = 6 (ext. start)"
          n387 = call-dynamic "Read Sync Box.lvclass.vi"("error in (no error)"=w1023, "SPARC4_AC in"=w1022) -> ("error out"=w1025:errorcluster, "Sync Box.lvclass"=w1026:refnum<class "Sync Box.lvclass">, "SPARC4_AC out"=w1021:refnum<class "S4GUI.lvclass">)  [unwired: 7 in]
          n388 = call "Read connection.vi"("error in (no error)"=w1025, "Server in"=w1026) -> ("error out"=w1024:errorcluster, "connection"=w986:bool)  [unwired: 7 in, 1 out]
          n389 = case shown="True" w986 {
            tunnel: [u8 6 ("TRIGGER_MODE") u8 0 ("TRIGGER_MODE")] -> w1003
            frame True {
            }
            frame False {
            }
          }
          n390 = call-dynamic "Read AcquisitionA.vi"("error in (no error)"=w1024, "S4ACS_GUI in"=w1021) -> ("error out"=w1008:errorcluster, "Acquisition.lvclass"=w1009:refnum<class "Acquisition.lvclass">, "S4ACS_GUI out"=w1007:refnum<class "S4GUI.lvclass">)  [unwired: 7 in]
          n391 = call-dynamic "Read Channel.vi"("error in (no error)"=w1008, "Acquisition in"=w1009) -> ("error out"=w991:errorcluster, "Channel.lvclass"=w990:refnum<class "Channel.lvclass">, "Acquisition out"=w1018:refnum<class "Acquisition.lvclass">)  [unwired: 7 in]
          n392 = call-dynamic "Read Interface.vi"("error in (no error)"=w991, "Channel in"=w990) -> ("error out"=w989:errorcluster, "Interface.lvclass"=w995:refnum<class "Interface.lvclass">, "Channel out"=w994:refnum<class "Channel.lvclass">)  [unwired: 7 in]
          n393 = call-dynamic "Get CCD_Config.vi"("error in (no error)"=w989, "Interface in"=w995) -> ("error out"=w1002:errorcluster, "output cluster"=w1004:T1, "Interface out"=w1001:refnum<class "Interface.lvclass">)  [unwired: 7 in]
          n394 = Bundle By Name(cluster=w1004, "TRIGGER_MODE"=w1003) -> (w1000:T1)
          n395 = call-dynamic "Set CCD_Config.vi"("error in (no error)"=w1002, "input cluster"=w1000, "Interface in"=w1001) -> ("error out"=w998:errorcluster, "Interface out"=w996:refnum<class "Interface.lvclass">)  [unwired: 7 in]
          n396 = Flatten To String(anything=w1000, error in (no error)=w998) -> (data string=w999:string, error out=w997:errorcluster)  [unwired: 2 in, 1 out]
          n397 = call "Write flatted cluster.vi"("error in (no error)"=w997, "flatted cluster"=w999, "Interface in"=w996) -> ("error out"=w992:errorcluster, "Interface out"=w993:refnum<class "Interface.lvclass">)  [unwired: 7 in]
          n398 = Increment(x=w1029) -> (x+1=w1028:u32)
          n399 = call-dynamic "Write Interface.vi"("error in (no error)"=w992, "Interface.lvclass"=w993, "Channel in"=w994) -> ("error out"=w988:errorcluster, "Channel out"=w987:refnum<class "Channel.lvclass">)  [unwired: 7 in]
          n400 = call-dynamic "Read State Machine.vi"("error in (no error)"=w988, "Device in"=w987) -> ("error out"=w1015:errorcluster, "State Machine.lvclass"=w1017:refnum<class "State Machine.lvclass">, "Device out"=w1013:refnum<class "Channel.lvclass">)  [unwired: 7 in]
          n401 = call "Next State.vi"("error in (no error)"=w1015, "New_State"=60, "State Machine in"=w1017) -> ("error out"=w1010:errorcluster, "State Machine out"=w1011:refnum<class "State Machine.lvclass">)  [unwired: 7 in]
          n402 = call-dynamic "Write State Machine.vi"("error in (no error)"=w1010, "State Machine.lvclass"=w1011, "Device in"=w1013) -> ("error out"=w1012:errorcluster, "Device out"=w1014:refnum<class "Channel.lvclass">)  [unwired: 7 in]
          n403 = call-dynamic "Write Channel.vi"("error in (no error)"=w1012, "Channel.lvclass"=w1014, "Acquisition in"=w1018) -> ("error out"=w1005:errorcluster, "Acquisition out"=w1006:refnum<class "Acquisition.lvclass">)  [unwired: 7 in]
          n404 = call-dynamic "Write AcquisitionA.vi"("error in (no error)"=w1005, "Acquisition.lvclass"=w1006, "S4ACS_GUI in"=w1007) -> ("error out"=w1020:errorcluster, "S4ACS_GUI out"=w1019:refnum<class "S4GUI.lvclass">)  [unwired: 7 in]
          n405 = Bundle By Name(cluster=w1019, "Obs_state"=w1028) -> (w1027:refnum<class "S4GUI.lvclass">)
        }
        frame 254 {
          # "Espera terminar a execução do comando atual \nantes de ir ao proximo passo da Observação."
          n406 = call-dynamic "Read AcquisitionA.vi"("error in (no error)"=w1049, "S4ACS_GUI in"=w1050) -> ("error out"=w1055:errorcluster, "Acquisition.lvclass"=w1056:refnum<class "Acquisition.lvclass">, "S4ACS_GUI out"=w1052:refnum<class "S4GUI.lvclass">)  [unwired: 7 in]
          n407 = call-dynamic "Read Channel.vi"("error in (no error)"=w1055, "Acquisition in"=w1056) -> ("error out"=w1047:errorcluster, "Channel.lvclass"=w1046:refnum<class "Channel.lvclass">, "Acquisition out"=w1054:refnum<class "Acquisition.lvclass">)  [unwired: 7 in]
          n408 = call-dynamic "Read State Machine.vi"("error in (no error)"=w1047, "Device in"=w1046) -> ("error out"=w1038:errorcluster, "State Machine.lvclass"=w1040:refnum<class "State Machine.lvclass">, "Device out"=w1044:refnum<class "Channel.lvclass">)  [unwired: 7 in]
          n409 = call-dynamic "Read State.vi"("error in (no error)"=w1038, "State Machine in"=w1040) -> ("error out"=w1037:errorcluster, "State"=w1034:i32, "State Machine out"=w1039:refnum<class "State Machine.lvclass">)  [unwired: 7 in]
          n410 = Equal To 0?(x=w1034) -> (x = 0?=w1036:bool)
          n411 = call-dynamic "Write State Machine.vi"("error in (no error)"=w1037, "State Machine.lvclass"=w1039, "Device in"=w1044) -> ("error out"=w1043:errorcluster, "Device out"=w1045:refnum<class "Channel.lvclass">)  [unwired: 7 in]
          n412 = call-dynamic "Write Channel.vi"("error in (no error)"=w1043, "Channel.lvclass"=w1045, "Acquisition in"=w1054) -> ("error out"=w1051:errorcluster, "Acquisition out"=w1053:refnum<class "Acquisition.lvclass">)  [unwired: 7 in]
          n413 = disable-structure shown="Enabled" {
            disable-tunnel: [u32 299 ("t") w1058] -> w1033
            disable-tunnel: w1032 -> [_ w1059]
            frame Disabled {
            }
            frame Enabled {
              n414 = Increment(x=w1059) -> (x+1=w1058:u32)
            }
          }
          n415 = Select(t=w1033, s=w1036, f=w1032) -> (s? t:f=w1035:u32)
          n416 = call-dynamic "Write AcquisitionA.vi"("error in (no error)"=w1051, "Acquisition.lvclass"=w1053, "S4ACS_GUI in"=w1052) -> ("error out"=w1048:errorcluster, "S4ACS_GUI out"=w1042:refnum<class "S4GUI.lvclass">)  [unwired: 7 in]
          n417 = Bundle By Name(cluster=w1042, "Obs_state"=w1035) -> (w1041:refnum<class "S4GUI.lvclass">)
        }
        frame 255 {
          n418 = call "Read AcquisitionB.vi"("error in (no error)"=w1070, "S4ACS_GUI in"=w1071) -> ("error out"=w1063:errorcluster, "Acquisition.lvclass"=w1064:refnum<class "Acquisition.lvclass">, "S4ACS_GUI out"=w1073:refnum<class "S4GUI.lvclass">)  [unwired: 7 in]
          n419 = call "Read connection.vi"("error in (no error)"=w1063, "Server in"=w1064) -> ("error out"=w1062:errorcluster, "connection"=w1060:bool, "Server out"=w1061:refnum<class "Acquisition.lvclass">)  [unwired: 7 in]
          n420 = case shown="False" w1060 {
            tunnel: w1061 -> [w1081 w1101]
            tunnel: w1062 -> [w1080 w1100]
            tunnel: [w1081 w1098] -> w1074
            tunnel: [w1080 w1097] -> w1072
            tunnel: w1067 -> [w1079 w1090]
            tunnel: [w1075 w1089] -> w1066
            frame False {
              n421 = Increment(x=w1079) -> (x+1=w1078:u32)
              n422 = Increment(x=w1078) -> (x+1=w1077:u32)
              n423 = Increment(x=w1077) -> (x+1=w1076:u32)
              n424 = Increment(x=w1076) -> (x+1=w1075:u32)
            }
            frame True {
              # "configura o canal,\nmas não dispara\na exposicao."
              n425 = call-dynamic "Read Channel.vi"("error in (no error)"=w1100, "Acquisition in"=w1101) -> ("error out"=w1086:errorcluster, "Channel.lvclass"=w1088:refnum<class "Channel.lvclass">, "Acquisition out"=w1099:refnum<class "Acquisition.lvclass">)  [unwired: 7 in]
              n426 = call-dynamic "Write expose.vi"("error in (no error)"=w1086, "expose"=FALSE, "Channel in"=w1088) -> ("error out"=w1085:errorcluster, "Channel out"=w1087:refnum<class "Channel.lvclass">)  [unwired: 7 in]
              n427 = call-dynamic "Read State Machine.vi"("error in (no error)"=w1085, "Device in"=w1087) -> ("error out"=w1094:errorcluster, "State Machine.lvclass"=w1096:refnum<class "State Machine.lvclass">, "Device out"=w1092:refnum<class "Channel.lvclass">)  [unwired: 7 in]
              n428 = call "Next State.vi"("error in (no error)"=w1094, "New_State"=1, "State Machine in"=w1096) -> ("error out"=w1082:errorcluster, "State Machine out"=w1083:refnum<class "State Machine.lvclass">)  [unwired: 7 in]
              n429 = Increment(x=w1090) -> (x+1=w1089:u32)
              n430 = call-dynamic "Write State Machine.vi"("error in (no error)"=w1082, "State Machine.lvclass"=w1083, "Device in"=w1092) -> ("error out"=w1091:errorcluster, "Device out"=w1093:refnum<class "Channel.lvclass">)  [unwired: 7 in]
              n431 = call-dynamic "Write Channel.vi"("error in (no error)"=w1091, "Channel.lvclass"=w1093, "Acquisition in"=w1099) -> ("error out"=w1097:errorcluster, "Acquisition out"=w1098:refnum<class "Acquisition.lvclass">)  [unwired: 7 in]
            }
          }
          n432 = call "Write AcquisitionB.vi"("error in (no error)"=w1072, "Acquisition.lvclass"=w1074, "S4ACS_GUI in"=w1073) -> ("error out"=w1069:errorcluster, "S4ACS_GUI out"=w1068:refnum<class "S4GUI.lvclass">)  [unwired: 7 in]
          n433 = Bundle By Name(cluster=w1068, "Obs_state"=w1066) -> (w1065:refnum<class "S4GUI.lvclass">)
        }
        frame 256 {
          # "Espera terminar a execução do comando atual \nantes de ir ao proximo passo da Observação."
          n434 = call "Read AcquisitionB.vi"("error in (no error)"=w1119, "S4ACS_GUI in"=w1120) -> ("error out"=w1125:errorcluster, "Acquisition.lvclass"=w1126:refnum<class "Acquisition.lvclass">, "S4ACS_GUI out"=w1122:refnum<class "S4GUI.lvclass">)  [unwired: 7 in]
          n435 = call-dynamic "Read Channel.vi"("error in (no error)"=w1125, "Acquisition in"=w1126) -> ("error out"=w1117:errorcluster, "Channel.lvclass"=w1116:refnum<class "Channel.lvclass">, "Acquisition out"=w1124:refnum<class "Acquisition.lvclass">)  [unwired: 7 in]
          n436 = call-dynamic "Read State Machine.vi"("error in (no error)"=w1117, "Device in"=w1116) -> ("error out"=w1108:errorcluster, "State Machine.lvclass"=w1110:refnum<class "State Machine.lvclass">, "Device out"=w1114:refnum<class "Channel.lvclass">)  [unwired: 7 in]
          n437 = call-dynamic "Read State.vi"("error in (no error)"=w1108, "State Machine in"=w1110) -> ("error out"=w1107:errorcluster, "State"=w1104:i32, "State Machine out"=w1109:refnum<class "State Machine.lvclass">)  [unwired: 7 in]
          n438 = call-dynamic "Write State Machine.vi"("error in (no error)"=w1107, "State Machine.lvclass"=w1109, "Device in"=w1114) -> ("error out"=w1113:errorcluster, "Device out"=w1115:refnum<class "Channel.lvclass">)  [unwired: 7 in]
          n439 = call-dynamic "Write Channel.vi"("error in (no error)"=w1113, "Channel.lvclass"=w1115, "Acquisition in"=w1124) -> ("error out"=w1121:errorcluster, "Acquisition out"=w1123:refnum<class "Acquisition.lvclass">)  [unwired: 7 in]
          n440 = Equal To 0?(x=w1104) -> (x = 0?=w1106:bool)
          n441 = disable-structure shown="Enabled" {
            disable-tunnel: [u32 299 ("t") w1128] -> w1102
            disable-tunnel: w1103 -> [_ w1131]
            frame Disabled {
            }
            frame Enabled {
              n442 = Increment(x=w1131) -> (x+1=w1130:u32)
              n443 = Increment(x=w1130) -> (x+1=w1129:u32)
              n444 = Increment(x=w1129) -> (x+1=w1128:u32)
            }
          }
          n445 = Select(t=w1102, s=w1106, f=w1103) -> (s? t:f=w1105:u32)
          n446 = call "Write AcquisitionB.vi"("error in (no error)"=w1121, "Acquisition.lvclass"=w1123, "S4ACS_GUI in"=w1122) -> ("error out"=w1118:errorcluster, "S4ACS_GUI out"=w1112:refnum<class "S4GUI.lvclass">)  [unwired: 7 in]
          n447 = Bundle By Name(cluster=w1112, "Obs_state"=w1105) -> (w1111:refnum<class "S4GUI.lvclass">)
        }
        frame 257 {
          # "Sem SyncBox, \ntrigger mode = 0 (internal)\nCom SyncBox\ntrigger mode = 6 (ext. start)"
          n448 = call-dynamic "Read Sync Box.lvclass.vi"("error in (no error)"=w1169, "SPARC4_AC in"=w1168) -> ("error out"=w1171:errorcluster, "Sync Box.lvclass"=w1172:refnum<class "Sync Box.lvclass">, "SPARC4_AC out"=w1167:refnum<class "S4GUI.lvclass">)  [unwired: 7 in]
          n449 = call "Read connection.vi"("error in (no error)"=w1171, "Server in"=w1172) -> ("error out"=w1170:errorcluster, "connection"=w1133:bool)  [unwired: 7 in, 1 out]
          n450 = case shown="False" w1133 {
            tunnel: [u8 6 ("TRIGGER_MODE") u8 0 ("TRIGGER_MODE")] -> w1132
            frame True {
            }
            frame False {
            }
          }
          n451 = call "Read AcquisitionB.vi"("error in (no error)"=w1170, "S4ACS_GUI in"=w1167) -> ("error out"=w1154:errorcluster, "Acquisition.lvclass"=w1155:refnum<class "Acquisition.lvclass">, "S4ACS_GUI out"=w1153:refnum<class "S4GUI.lvclass">)  [unwired: 7 in]
          n452 = call-dynamic "Read Channel.vi"("error in (no error)"=w1154, "Acquisition in"=w1155) -> ("error out"=w1138:errorcluster, "Channel.lvclass"=w1137:refnum<class "Channel.lvclass">, "Acquisition out"=w1164:refnum<class "Acquisition.lvclass">)  [unwired: 7 in]
          n453 = call-dynamic "Read Interface.vi"("error in (no error)"=w1138, "Channel in"=w1137) -> ("error out"=w1136:errorcluster, "Interface.lvclass"=w1142:refnum<class "Interface.lvclass">, "Channel out"=w1141:refnum<class "Channel.lvclass">)  [unwired: 7 in]
          n454 = call-dynamic "Get CCD_Config.vi"("error in (no error)"=w1136, "Interface in"=w1142) -> ("error out"=w1149:errorcluster, "output cluster"=w1150:T1, "Interface out"=w1148:refnum<class "Interface.lvclass">)  [unwired: 7 in]
          n455 = Bundle By Name(cluster=w1150, "TRIGGER_MODE"=w1132) -> (w1147:T1)
          n456 = call-dynamic "Set CCD_Config.vi"("error in (no error)"=w1149, "input cluster"=w1147, "Interface in"=w1148) -> ("error out"=w1145:errorcluster, "Interface out"=w1143:refnum<class "Interface.lvclass">)  [unwired: 7 in]
          n457 = Flatten To String(anything=w1147, error in (no error)=w1145) -> (data string=w1146:string, error out=w1144:errorcluster)  [unwired: 2 in, 1 out]
          n458 = call "Write flatted cluster.vi"("error in (no error)"=w1144, "flatted cluster"=w1146, "Interface in"=w1143) -> ("error out"=w1139:errorcluster, "Interface out"=w1140:refnum<class "Interface.lvclass">)  [unwired: 7 in]
          n459 = Increment(x=w1175) -> (x+1=w1174:u32)
          n460 = call-dynamic "Write Interface.vi"("error in (no error)"=w1139, "Interface.lvclass"=w1140, "Channel in"=w1141) -> ("error out"=w1135:errorcluster, "Channel out"=w1134:refnum<class "Channel.lvclass">)  [unwired: 7 in]
          n461 = call-dynamic "Read State Machine.vi"("error in (no error)"=w1135, "Device in"=w1134) -> ("error out"=w1161:errorcluster, "State Machine.lvclass"=w1163:refnum<class "State Machine.lvclass">, "Device out"=w1159:refnum<class "Channel.lvclass">)  [unwired: 7 in]
          n462 = call "Next State.vi"("error in (no error)"=w1161, "New_State"=60, "State Machine in"=w1163) -> ("error out"=w1156:errorcluster, "State Machine out"=w1157:refnum<class "State Machine.lvclass">)  [unwired: 7 in]
          n463 = call-dynamic "Write State Machine.vi"("error in (no error)"=w1156, "State Machine.lvclass"=w1157, "Device in"=w1159) -> ("error out"=w1158:errorcluster, "Device out"=w1160:refnum<class "Channel.lvclass">)  [unwired: 7 in]
          n464 = call-dynamic "Write Channel.vi"("error in (no error)"=w1158, "Channel.lvclass"=w1160, "Acquisition in"=w1164) -> ("error out"=w1151:errorcluster, "Acquisition out"=w1152:refnum<class "Acquisition.lvclass">)  [unwired: 7 in]
          n465 = call "Write AcquisitionB.vi"("error in (no error)"=w1151, "Acquisition.lvclass"=w1152, "S4ACS_GUI in"=w1153) -> ("error out"=w1166:errorcluster, "S4ACS_GUI out"=w1165:refnum<class "S4GUI.lvclass">)  [unwired: 7 in]
          n466 = Bundle By Name(cluster=w1165, "Obs_state"=w1174) -> (w1173:refnum<class "S4GUI.lvclass">)
        }
        frame 258 {
          # "Espera terminar a execução do comando atual \nantes de ir ao proximo passo da Observação."
          n467 = call "Read AcquisitionB.vi"("error in (no error)"=w1195, "S4ACS_GUI in"=w1196) -> ("error out"=w1201:errorcluster, "Acquisition.lvclass"=w1202:refnum<class "Acquisition.lvclass">, "S4ACS_GUI out"=w1198:refnum<class "S4GUI.lvclass">)  [unwired: 7 in]
          n468 = call-dynamic "Read Channel.vi"("error in (no error)"=w1201, "Acquisition in"=w1202) -> ("error out"=w1193:errorcluster, "Channel.lvclass"=w1192:refnum<class "Channel.lvclass">, "Acquisition out"=w1200:refnum<class "Acquisition.lvclass">)  [unwired: 7 in]
          n469 = call-dynamic "Read State Machine.vi"("error in (no error)"=w1193, "Device in"=w1192) -> ("error out"=w1184:errorcluster, "State Machine.lvclass"=w1186:refnum<class "State Machine.lvclass">, "Device out"=w1190:refnum<class "Channel.lvclass">)  [unwired: 7 in]
          n470 = call-dynamic "Read State.vi"("error in (no error)"=w1184, "State Machine in"=w1186) -> ("error out"=w1183:errorcluster, "State"=w1180:i32, "State Machine out"=w1185:refnum<class "State Machine.lvclass">)  [unwired: 7 in]
          n471 = call-dynamic "Write State Machine.vi"("error in (no error)"=w1183, "State Machine.lvclass"=w1185, "Device in"=w1190) -> ("error out"=w1189:errorcluster, "Device out"=w1191:refnum<class "Channel.lvclass">)  [unwired: 7 in]
          n472 = call-dynamic "Write Channel.vi"("error in (no error)"=w1189, "Channel.lvclass"=w1191, "Acquisition in"=w1200) -> ("error out"=w1197:errorcluster, "Acquisition out"=w1199:refnum<class "Acquisition.lvclass">)  [unwired: 7 in]
          n473 = Equal To 0?(x=w1180) -> (x = 0?=w1182:bool)
          n474 = Increment(x=w1179) -> (x+1=w1178:u32)
          n475 = Select(t=w1178, s=w1182, f=w1179) -> (s? t:f=w1181:u32)
          n476 = call "Write AcquisitionB.vi"("error in (no error)"=w1197, "Acquisition.lvclass"=w1199, "S4ACS_GUI in"=w1198) -> ("error out"=w1194:errorcluster, "S4ACS_GUI out"=w1188:refnum<class "S4GUI.lvclass">)  [unwired: 7 in]
          n477 = Bundle By Name(cluster=w1188, "Obs_state"=w1181) -> (w1187:refnum<class "S4GUI.lvclass">)
        }
        frame 259 {
          n478 = call-dynamic "Read AcquisitionC.vi"("error in (no error)"=w1213, "S4ACS_GUI in"=w1214) -> ("error out"=w1205:errorcluster, "Acquisition.lvclass"=w1207:refnum<class "Acquisition.lvclass">, "S4ACS_GUI out"=w1216:refnum<class "S4GUI.lvclass">)  [unwired: 7 in]
          n479 = call "Read connection.vi"("error in (no error)"=w1205, "Server in"=w1207) -> ("error out"=w1204:errorcluster, "connection"=w1203:bool, "Server out"=w1206:refnum<class "Acquisition.lvclass">)  [unwired: 7 in]
          n480 = case shown="True" w1203 {
            tunnel: w1206 -> [w1223 w1244]
            tunnel: w1204 -> [w1224 w1243]
            tunnel: [w1223 w1241] -> w1217
            tunnel: [w1224 w1240] -> w1215
            tunnel: w1210 -> [w1222 w1233]
            tunnel: [w1218 w1232] -> w1209
            frame False {
              n481 = Increment(x=w1222) -> (x+1=w1221:u32)
              n482 = Increment(x=w1221) -> (x+1=w1220:u32)
              n483 = Increment(x=w1220) -> (x+1=w1219:u32)
              n484 = Increment(x=w1219) -> (x+1=w1218:u32)
            }
            frame True {
              # "configura o canal,\nmas não dispara\na exposicao."
              n485 = call-dynamic "Read Channel.vi"("error in (no error)"=w1243, "Acquisition in"=w1244) -> ("error out"=w1229:errorcluster, "Channel.lvclass"=w1231:refnum<class "Channel.lvclass">, "Acquisition out"=w1242:refnum<class "Acquisition.lvclass">)  [unwired: 7 in]
              n486 = call-dynamic "Write expose.vi"("error in (no error)"=w1229, "expose"=FALSE, "Channel in"=w1231) -> ("error out"=w1228:errorcluster, "Channel out"=w1230:refnum<class "Channel.lvclass">)  [unwired: 7 in]
              n487 = call-dynamic "Read State Machine.vi"("error in (no error)"=w1228, "Device in"=w1230) -> ("error out"=w1237:errorcluster, "State Machine.lvclass"=w1239:refnum<class "State Machine.lvclass">, "Device out"=w1235:refnum<class "Channel.lvclass">)  [unwired: 7 in]
              n488 = call "Next State.vi"("error in (no error)"=w1237, "New_State"=1, "State Machine in"=w1239) -> ("error out"=w1225:errorcluster, "State Machine out"=w1226:refnum<class "State Machine.lvclass">)  [unwired: 7 in]
              n489 = Increment(x=w1233) -> (x+1=w1232:u32)
              n490 = call-dynamic "Write State Machine.vi"("error in (no error)"=w1225, "State Machine.lvclass"=w1226, "Device in"=w1235) -> ("error out"=w1234:errorcluster, "Device out"=w1236:refnum<class "Channel.lvclass">)  [unwired: 7 in]
              n491 = call-dynamic "Write Channel.vi"("error in (no error)"=w1234, "Channel.lvclass"=w1236, "Acquisition in"=w1242) -> ("error out"=w1240:errorcluster, "Acquisition out"=w1241:refnum<class "Acquisition.lvclass">)  [unwired: 7 in]
            }
          }
          n492 = call-dynamic "Write AcquisitionC.vi"("error in (no error)"=w1215, "Acquisition.lvclass"=w1217, "S4ACS_GUI in"=w1216) -> ("error out"=w1212:errorcluster, "S4ACS_GUI out"=w1211:refnum<class "S4GUI.lvclass">)  [unwired: 7 in]
          n493 = Bundle By Name(cluster=w1211, "Obs_state"=w1209) -> (w1208:refnum<class "S4GUI.lvclass">)
        }
        frame 260 {
          # "Espera terminar a execução do comando atual \nantes de ir ao proximo passo da Observação."
          n494 = call-dynamic "Read AcquisitionC.vi"("error in (no error)"=w1262, "S4ACS_GUI in"=w1263) -> ("error out"=w1268:errorcluster, "Acquisition.lvclass"=w1269:refnum<class "Acquisition.lvclass">, "S4ACS_GUI out"=w1265:refnum<class "S4GUI.lvclass">)  [unwired: 7 in]
          n495 = call-dynamic "Read Channel.vi"("error in (no error)"=w1268, "Acquisition in"=w1269) -> ("error out"=w1260:errorcluster, "Channel.lvclass"=w1259:refnum<class "Channel.lvclass">, "Acquisition out"=w1267:refnum<class "Acquisition.lvclass">)  [unwired: 7 in]
          n496 = call-dynamic "Read State Machine.vi"("error in (no error)"=w1260, "Device in"=w1259) -> ("error out"=w1251:errorcluster, "State Machine.lvclass"=w1253:refnum<class "State Machine.lvclass">, "Device out"=w1257:refnum<class "Channel.lvclass">)  [unwired: 7 in]
          n497 = call-dynamic "Read State.vi"("error in (no error)"=w1251, "State Machine in"=w1253) -> ("error out"=w1250:errorcluster, "State"=w1247:i32, "State Machine out"=w1252:refnum<class "State Machine.lvclass">)  [unwired: 7 in]
          n498 = Equal To 0?(x=w1247) -> (x = 0?=w1249:bool)
          n499 = call-dynamic "Write State Machine.vi"("error in (no error)"=w1250, "State Machine.lvclass"=w1252, "Device in"=w1257) -> ("error out"=w1256:errorcluster, "Device out"=w1258:refnum<class "Channel.lvclass">)  [unwired: 7 in]
          n500 = call-dynamic "Write Channel.vi"("error in (no error)"=w1256, "Channel.lvclass"=w1258, "Acquisition in"=w1267) -> ("error out"=w1264:errorcluster, "Acquisition out"=w1266:refnum<class "Acquisition.lvclass">)  [unwired: 7 in]
          n501 = disable-structure shown="Enabled" {
            disable-tunnel: [u32 299 ("t") w1271] -> w1245
            disable-tunnel: w1246 -> [_ w1274]
            frame Disabled {
            }
            frame Enabled {
              n502 = Increment(x=w1274) -> (x+1=w1273:u32)
              n503 = Increment(x=w1273) -> (x+1=w1272:u32)
              n504 = Increment(x=w1272) -> (x+1=w1271:u32)
            }
          }
          n505 = Select(t=w1245, s=w1249, f=w1246) -> (s? t:f=w1248:u32)
          n506 = call-dynamic "Write AcquisitionC.vi"("error in (no error)"=w1264, "Acquisition.lvclass"=w1266, "S4ACS_GUI in"=w1265) -> ("error out"=w1261:errorcluster, "S4ACS_GUI out"=w1255:refnum<class "S4GUI.lvclass">)  [unwired: 7 in]
          n507 = Bundle By Name(cluster=w1255, "Obs_state"=w1248) -> (w1254:refnum<class "S4GUI.lvclass">)
        }
        frame 261 {
          # "Sem SyncBox, \ntrigger mode = 0 (internal)\nCom SyncBox\ntrigger mode = 6 (ext. start)"
          n508 = call-dynamic "Read Sync Box.lvclass.vi"("error in (no error)"=w1312, "SPARC4_AC in"=w1311) -> ("error out"=w1314:errorcluster, "Sync Box.lvclass"=w1315:refnum<class "Sync Box.lvclass">, "SPARC4_AC out"=w1310:refnum<class "S4GUI.lvclass">)  [unwired: 7 in]
          n509 = call "Read connection.vi"("error in (no error)"=w1314, "Server in"=w1315) -> ("error out"=w1313:errorcluster, "connection"=w1276:bool)  [unwired: 7 in, 1 out]
          n510 = case shown="False" w1276 {
            tunnel: [u8 6 ("TRIGGER_MODE") u8 0 ("TRIGGER_MODE")] -> w1275
            frame True {
            }
            frame False {
            }
          }
          n511 = call-dynamic "Read AcquisitionC.vi"("error in (no error)"=w1313, "S4ACS_GUI in"=w1310) -> ("error out"=w1297:errorcluster, "Acquisition.lvclass"=w1298:refnum<class "Acquisition.lvclass">, "S4ACS_GUI out"=w1296:refnum<class "S4GUI.lvclass">)  [unwired: 7 in]
          n512 = call-dynamic "Read Channel.vi"("error in (no error)"=w1297, "Acquisition in"=w1298) -> ("error out"=w1281:errorcluster, "Channel.lvclass"=w1280:refnum<class "Channel.lvclass">, "Acquisition out"=w1307:refnum<class "Acquisition.lvclass">)  [unwired: 7 in]
          n513 = call-dynamic "Read Interface.vi"("error in (no error)"=w1281, "Channel in"=w1280) -> ("error out"=w1279:errorcluster, "Interface.lvclass"=w1285:refnum<class "Interface.lvclass">, "Channel out"=w1284:refnum<class "Channel.lvclass">)  [unwired: 7 in]
          n514 = call-dynamic "Get CCD_Config.vi"("error in (no error)"=w1279, "Interface in"=w1285) -> ("error out"=w1292:errorcluster, "output cluster"=w1293:T1, "Interface out"=w1291:refnum<class "Interface.lvclass">)  [unwired: 7 in]
          n515 = Bundle By Name(cluster=w1293, "TRIGGER_MODE"=w1275) -> (w1290:T1)
          n516 = call-dynamic "Set CCD_Config.vi"("error in (no error)"=w1292, "input cluster"=w1290, "Interface in"=w1291) -> ("error out"=w1288:errorcluster, "Interface out"=w1286:refnum<class "Interface.lvclass">)  [unwired: 7 in]
          n517 = Flatten To String(anything=w1290, error in (no error)=w1288) -> (data string=w1289:string, error out=w1287:errorcluster)  [unwired: 2 in, 1 out]
          n518 = call "Write flatted cluster.vi"("error in (no error)"=w1287, "flatted cluster"=w1289, "Interface in"=w1286) -> ("error out"=w1282:errorcluster, "Interface out"=w1283:refnum<class "Interface.lvclass">)  [unwired: 7 in]
          n519 = Increment(x=w1318) -> (x+1=w1317:u32)
          n520 = call-dynamic "Write Interface.vi"("error in (no error)"=w1282, "Interface.lvclass"=w1283, "Channel in"=w1284) -> ("error out"=w1278:errorcluster, "Channel out"=w1277:refnum<class "Channel.lvclass">)  [unwired: 7 in]
          n521 = call-dynamic "Read State Machine.vi"("error in (no error)"=w1278, "Device in"=w1277) -> ("error out"=w1304:errorcluster, "State Machine.lvclass"=w1306:refnum<class "State Machine.lvclass">, "Device out"=w1302:refnum<class "Channel.lvclass">)  [unwired: 7 in]
          n522 = call "Next State.vi"("error in (no error)"=w1304, "New_State"=60, "State Machine in"=w1306) -> ("error out"=w1299:errorcluster, "State Machine out"=w1300:refnum<class "State Machine.lvclass">)  [unwired: 7 in]
          n523 = call-dynamic "Write State Machine.vi"("error in (no error)"=w1299, "State Machine.lvclass"=w1300, "Device in"=w1302) -> ("error out"=w1301:errorcluster, "Device out"=w1303:refnum<class "Channel.lvclass">)  [unwired: 7 in]
          n524 = call-dynamic "Write Channel.vi"("error in (no error)"=w1301, "Channel.lvclass"=w1303, "Acquisition in"=w1307) -> ("error out"=w1294:errorcluster, "Acquisition out"=w1295:refnum<class "Acquisition.lvclass">)  [unwired: 7 in]
          n525 = call-dynamic "Write AcquisitionC.vi"("error in (no error)"=w1294, "Acquisition.lvclass"=w1295, "S4ACS_GUI in"=w1296) -> ("error out"=w1309:errorcluster, "S4ACS_GUI out"=w1308:refnum<class "S4GUI.lvclass">)  [unwired: 7 in]
          n526 = Bundle By Name(cluster=w1308, "Obs_state"=w1317) -> (w1316:refnum<class "S4GUI.lvclass">)
        }
        frame 262 {
          # "Espera terminar a execução do comando atual \nantes de ir ao proximo passo da Observação."
          n527 = call-dynamic "Read AcquisitionC.vi"("error in (no error)"=w1338, "S4ACS_GUI in"=w1339) -> ("error out"=w1344:errorcluster, "Acquisition.lvclass"=w1345:refnum<class "Acquisition.lvclass">, "S4ACS_GUI out"=w1341:refnum<class "S4GUI.lvclass">)  [unwired: 7 in]
          n528 = call-dynamic "Read Channel.vi"("error in (no error)"=w1344, "Acquisition in"=w1345) -> ("error out"=w1336:errorcluster, "Channel.lvclass"=w1335:refnum<class "Channel.lvclass">, "Acquisition out"=w1343:refnum<class "Acquisition.lvclass">)  [unwired: 7 in]
          n529 = call-dynamic "Read State Machine.vi"("error in (no error)"=w1336, "Device in"=w1335) -> ("error out"=w1327:errorcluster, "State Machine.lvclass"=w1329:refnum<class "State Machine.lvclass">, "Device out"=w1333:refnum<class "Channel.lvclass">)  [unwired: 7 in]
          n530 = call-dynamic "Read State.vi"("error in (no error)"=w1327, "State Machine in"=w1329) -> ("error out"=w1326:errorcluster, "State"=w1323:i32, "State Machine out"=w1328:refnum<class "State Machine.lvclass">)  [unwired: 7 in]
          n531 = Equal To 0?(x=w1323) -> (x = 0?=w1325:bool)
          n532 = call-dynamic "Write State Machine.vi"("error in (no error)"=w1326, "State Machine.lvclass"=w1328, "Device in"=w1333) -> ("error out"=w1332:errorcluster, "Device out"=w1334:refnum<class "Channel.lvclass">)  [unwired: 7 in]
          n533 = call-dynamic "Write Channel.vi"("error in (no error)"=w1332, "Channel.lvclass"=w1334, "Acquisition in"=w1343) -> ("error out"=w1340:errorcluster, "Acquisition out"=w1342:refnum<class "Acquisition.lvclass">)  [unwired: 7 in]
          n534 = Increment(x=w1322) -> (x+1=w1321:u32)
          n535 = Select(t=w1321, s=w1325, f=w1322) -> (s? t:f=w1324:u32)
          n536 = call-dynamic "Write AcquisitionC.vi"("error in (no error)"=w1340, "Acquisition.lvclass"=w1342, "S4ACS_GUI in"=w1341) -> ("error out"=w1337:errorcluster, "S4ACS_GUI out"=w1331:refnum<class "S4GUI.lvclass">)  [unwired: 7 in]
          n537 = Bundle By Name(cluster=w1331, "Obs_state"=w1324) -> (w1330:refnum<class "S4GUI.lvclass">)
        }
        frame 263 {
          # "Dispara o comando para o dispositivo corrente."
          n538 = call-dynamic "Read AcquisitionD.vi"("error in (no error)"=w1356, "S4ACS_GUI in"=w1357) -> ("error out"=w1349:errorcluster, "Acquisition.lvclass"=w1350:refnum<class "Acquisition.lvclass">, "S4ACS_GUI out"=w1359:refnum<class "S4GUI.lvclass">)  [unwired: 7 in]
          n539 = call "Read connection.vi"("error in (no error)"=w1349, "Server in"=w1350) -> ("error out"=w1347:errorcluster, "connection"=w1346:bool, "Server out"=w1348:refnum<class "Acquisition.lvclass">)  [unwired: 7 in]
          n540 = case shown="True" w1346 {
            tunnel: w1348 -> [w1363 w1383]
            tunnel: w1347 -> [w1362 w1382]
            tunnel: [w1363 w1380] -> w1360
            tunnel: [w1362 w1379] -> w1358
            tunnel: w1353 -> [_ w1372]
            tunnel: [u32 299 w1371] -> w1352
            frame False {
            }
            frame True {
              # "configura o canal,\nmas não dispara\na exposicao."
              n541 = call-dynamic "Read Channel.vi"("error in (no error)"=w1382, "Acquisition in"=w1383) -> ("error out"=w1368:errorcluster, "Channel.lvclass"=w1370:refnum<class "Channel.lvclass">, "Acquisition out"=w1381:refnum<class "Acquisition.lvclass">)  [unwired: 7 in]
              n542 = call-dynamic "Write expose.vi"("error in (no error)"=w1368, "expose"=FALSE, "Channel in"=w1370) -> ("error out"=w1367:errorcluster, "Channel out"=w1369:refnum<class "Channel.lvclass">)  [unwired: 7 in]
              n543 = call-dynamic "Read State Machine.vi"("error in (no error)"=w1367, "Device in"=w1369) -> ("error out"=w1376:errorcluster, "State Machine.lvclass"=w1378:refnum<class "State Machine.lvclass">, "Device out"=w1374:refnum<class "Channel.lvclass">)  [unwired: 7 in]
              n544 = call "Next State.vi"("error in (no error)"=w1376, "New_State"=1, "State Machine in"=w1378) -> ("error out"=w1364:errorcluster, "State Machine out"=w1365:refnum<class "State Machine.lvclass">)  [unwired: 7 in]
              n545 = Increment(x=w1372) -> (x+1=w1371:u32)
              n546 = call-dynamic "Write State Machine.vi"("error in (no error)"=w1364, "State Machine.lvclass"=w1365, "Device in"=w1374) -> ("error out"=w1373:errorcluster, "Device out"=w1375:refnum<class "Channel.lvclass">)  [unwired: 7 in]
              n547 = call-dynamic "Write Channel.vi"("error in (no error)"=w1373, "Channel.lvclass"=w1375, "Acquisition in"=w1381) -> ("error out"=w1379:errorcluster, "Acquisition out"=w1380:refnum<class "Acquisition.lvclass">)  [unwired: 7 in]
            }
          }
          n548 = call-dynamic "Write AcquisitionD.vi"("error in (no error)"=w1358, "Acquisition.lvclass"=w1360, "S4ACS_GUI in"=w1359) -> ("error out"=w1355:errorcluster, "S4ACS_GUI out"=w1354:refnum<class "S4GUI.lvclass">)  [unwired: 7 in]
          n549 = Bundle By Name(cluster=w1354, "Obs_state"=w1352) -> (w1351:refnum<class "S4GUI.lvclass">)
        }
        frame 264 {
          # "Espera terminar a execução do comando atual \nantes de ir ao proximo passo da Observação."
          n550 = call-dynamic "Read AcquisitionD.vi"("error in (no error)"=w1401, "S4ACS_GUI in"=w1402) -> ("error out"=w1407:errorcluster, "Acquisition.lvclass"=w1408:refnum<class "Acquisition.lvclass">, "S4ACS_GUI out"=w1404:refnum<class "S4GUI.lvclass">)  [unwired: 7 in]
          n551 = call-dynamic "Read Channel.vi"("error in (no error)"=w1407, "Acquisition in"=w1408) -> ("error out"=w1399:errorcluster, "Channel.lvclass"=w1398:refnum<class "Channel.lvclass">, "Acquisition out"=w1406:refnum<class "Acquisition.lvclass">)  [unwired: 7 in]
          n552 = call-dynamic "Read State Machine.vi"("error in (no error)"=w1399, "Device in"=w1398) -> ("error out"=w1390:errorcluster, "State Machine.lvclass"=w1392:refnum<class "State Machine.lvclass">, "Device out"=w1396:refnum<class "Channel.lvclass">)  [unwired: 7 in]
          n553 = call-dynamic "Read State.vi"("error in (no error)"=w1390, "State Machine in"=w1392) -> ("error out"=w1389:errorcluster, "State"=w1386:i32, "State Machine out"=w1391:refnum<class "State Machine.lvclass">)  [unwired: 7 in]
          n554 = Equal To 0?(x=w1386) -> (x = 0?=w1388:bool)
          n555 = call-dynamic "Write State Machine.vi"("error in (no error)"=w1389, "State Machine.lvclass"=w1391, "Device in"=w1396) -> ("error out"=w1395:errorcluster, "Device out"=w1397:refnum<class "Channel.lvclass">)  [unwired: 7 in]
          n556 = call-dynamic "Write Channel.vi"("error in (no error)"=w1395, "Channel.lvclass"=w1397, "Acquisition in"=w1406) -> ("error out"=w1403:errorcluster, "Acquisition out"=w1405:refnum<class "Acquisition.lvclass">)  [unwired: 7 in]
          n557 = disable-structure shown="Enabled" {
            disable-tunnel: w1385 -> [w1410 _]
            disable-tunnel: [w1409 u32 299] -> w1384
            frame Disabled {
              n558 = Increment(x=w1410) -> (x+1=w1409:u32)
            }
            frame Enabled {
            }
          }
          n559 = Select(t=w1384, s=w1388, f=w1385) -> (s? t:f=w1387:u32)
          n560 = call-dynamic "Write AcquisitionD.vi"("error in (no error)"=w1403, "Acquisition.lvclass"=w1405, "S4ACS_GUI in"=w1404) -> ("error out"=w1400:errorcluster, "S4ACS_GUI out"=w1394:refnum<class "S4GUI.lvclass">)  [unwired: 7 in]
          n561 = Bundle By Name(cluster=w1394, "Obs_state"=w1387) -> (w1393:refnum<class "S4GUI.lvclass">)
        }
        frame 265 {
          # "Sem SyncBox, \ntrigger mode = 0 (internal)\nCom SyncBox\ntrigger mode = 6 (ext. start)"
          n562 = call-dynamic "Read Sync Box.lvclass.vi"("error in (no error)"=w1449, "SPARC4_AC in"=w1448) -> ("error out"=w1451:errorcluster, "Sync Box.lvclass"=w1452:refnum<class "Sync Box.lvclass">, "SPARC4_AC out"=w1447:refnum<class "S4GUI.lvclass">)  [unwired: 7 in]
          n563 = call "Read connection.vi"("error in (no error)"=w1451, "Server in"=w1452) -> ("error out"=w1450:errorcluster, "connection"=w1413:bool)  [unwired: 7 in, 1 out]
          n564 = case shown="False" w1413 {
            tunnel: [u8 6 ("TRIGGER_MODE") u8 0 ("TRIGGER_MODE")] -> w1412
            frame True {
            }
            frame False {
            }
          }
          n565 = call-dynamic "Read AcquisitionD.vi"("error in (no error)"=w1450, "S4ACS_GUI in"=w1447) -> ("error out"=w1434:errorcluster, "Acquisition.lvclass"=w1435:refnum<class "Acquisition.lvclass">, "S4ACS_GUI out"=w1433:refnum<class "S4GUI.lvclass">)  [unwired: 7 in]
          n566 = call-dynamic "Read Channel.vi"("error in (no error)"=w1434, "Acquisition in"=w1435) -> ("error out"=w1418:errorcluster, "Channel.lvclass"=w1417:refnum<class "Channel.lvclass">, "Acquisition out"=w1444:refnum<class "Acquisition.lvclass">)  [unwired: 7 in]
          n567 = call-dynamic "Read Interface.vi"("error in (no error)"=w1418, "Channel in"=w1417) -> ("error out"=w1416:errorcluster, "Interface.lvclass"=w1422:refnum<class "Interface.lvclass">, "Channel out"=w1421:refnum<class "Channel.lvclass">)  [unwired: 7 in]
          n568 = call-dynamic "Get CCD_Config.vi"("error in (no error)"=w1416, "Interface in"=w1422) -> ("error out"=w1429:errorcluster, "output cluster"=w1430:T1, "Interface out"=w1428:refnum<class "Interface.lvclass">)  [unwired: 7 in]
          n569 = Bundle By Name(cluster=w1430, "TRIGGER_MODE"=w1412) -> (w1427:T1)
          n570 = call-dynamic "Set CCD_Config.vi"("error in (no error)"=w1429, "input cluster"=w1427, "Interface in"=w1428) -> ("error out"=w1425:errorcluster, "Interface out"=w1423:refnum<class "Interface.lvclass">)  [unwired: 7 in]
          n571 = Flatten To String(anything=w1427, error in (no error)=w1425) -> (data string=w1426:string, error out=w1424:errorcluster)  [unwired: 2 in, 1 out]
          n572 = call "Write flatted cluster.vi"("error in (no error)"=w1424, "flatted cluster"=w1426, "Interface in"=w1423) -> ("error out"=w1419:errorcluster, "Interface out"=w1420:refnum<class "Interface.lvclass">)  [unwired: 7 in]
          n573 = call-dynamic "Write Interface.vi"("error in (no error)"=w1419, "Interface.lvclass"=w1420, "Channel in"=w1421) -> ("error out"=w1415:errorcluster, "Channel out"=w1414:refnum<class "Channel.lvclass">)  [unwired: 7 in]
          n574 = call-dynamic "Read State Machine.vi"("error in (no error)"=w1415, "Device in"=w1414) -> ("error out"=w1441:errorcluster, "State Machine.lvclass"=w1443:refnum<class "State Machine.lvclass">, "Device out"=w1439:refnum<class "Channel.lvclass">)  [unwired: 7 in]
          n575 = Increment(x=w1455) -> (x+1=w1454:u32)
          n576 = call "Next State.vi"("error in (no error)"=w1441, "New_State"=60, "State Machine in"=w1443) -> ("error out"=w1436:errorcluster, "State Machine out"=w1437:refnum<class "State Machine.lvclass">)  [unwired: 7 in]
          n577 = call-dynamic "Write State Machine.vi"("error in (no error)"=w1436, "State Machine.lvclass"=w1437, "Device in"=w1439) -> ("error out"=w1438:errorcluster, "Device out"=w1440:refnum<class "Channel.lvclass">)  [unwired: 7 in]
          n578 = call-dynamic "Write Channel.vi"("error in (no error)"=w1438, "Channel.lvclass"=w1440, "Acquisition in"=w1444) -> ("error out"=w1431:errorcluster, "Acquisition out"=w1432:refnum<class "Acquisition.lvclass">)  [unwired: 7 in]
          n579 = call-dynamic "Write AcquisitionD.vi"("error in (no error)"=w1431, "Acquisition.lvclass"=w1432, "S4ACS_GUI in"=w1433) -> ("error out"=w1446:errorcluster, "S4ACS_GUI out"=w1445:refnum<class "S4GUI.lvclass">)  [unwired: 7 in]
          n580 = Bundle By Name(cluster=w1445, "Obs_state"=w1454) -> (w1453:refnum<class "S4GUI.lvclass">)
        }
        frame 266 {
          # "Espera terminar a execução do comando atual \nantes de ir ao proximo passo da Observação."
          n581 = call-dynamic "Read AcquisitionD.vi"("error in (no error)"=w1475, "S4ACS_GUI in"=w1476) -> ("error out"=w1481:errorcluster, "Acquisition.lvclass"=w1482:refnum<class "Acquisition.lvclass">, "S4ACS_GUI out"=w1478:refnum<class "S4GUI.lvclass">)  [unwired: 7 in]
          n582 = call-dynamic "Read Channel.vi"("error in (no error)"=w1481, "Acquisition in"=w1482) -> ("error out"=w1473:errorcluster, "Channel.lvclass"=w1472:refnum<class "Channel.lvclass">, "Acquisition out"=w1480:refnum<class "Acquisition.lvclass">)  [unwired: 7 in]
          n583 = call-dynamic "Read State Machine.vi"("error in (no error)"=w1473, "Device in"=w1472) -> ("error out"=w1464:errorcluster, "State Machine.lvclass"=w1466:refnum<class "State Machine.lvclass">, "Device out"=w1470:refnum<class "Channel.lvclass">)  [unwired: 7 in]
          n584 = call-dynamic "Read State.vi"("error in (no error)"=w1464, "State Machine in"=w1466) -> ("error out"=w1463:errorcluster, "State"=w1460:i32, "State Machine out"=w1465:refnum<class "State Machine.lvclass">)  [unwired: 7 in]
          n585 = Equal To 0?(x=w1460) -> (x = 0?=w1462:bool)
          n586 = call-dynamic "Write State Machine.vi"("error in (no error)"=w1463, "State Machine.lvclass"=w1465, "Device in"=w1470) -> ("error out"=w1469:errorcluster, "Device out"=w1471:refnum<class "Channel.lvclass">)  [unwired: 7 in]
          n587 = call-dynamic "Write Channel.vi"("error in (no error)"=w1469, "Channel.lvclass"=w1471, "Acquisition in"=w1480) -> ("error out"=w1477:errorcluster, "Acquisition out"=w1479:refnum<class "Acquisition.lvclass">)  [unwired: 7 in]
          n588 = Select(t=u32 299, s=w1462, f=w1459) -> (s? t:f=w1461:u32)
          n589 = call-dynamic "Write AcquisitionD.vi"("error in (no error)"=w1477, "Acquisition.lvclass"=w1479, "S4ACS_GUI in"=w1478) -> ("error out"=w1474:errorcluster, "S4ACS_GUI out"=w1468:refnum<class "S4GUI.lvclass">)  [unwired: 7 in]
          n590 = Bundle By Name(cluster=w1468, "Obs_state"=w1461) -> (w1467:refnum<class "S4GUI.lvclass">)
        }
        frame 299 {
          # "Verifica se é modo fotometria ou polarimetria:\nTrue = polarimetria\nFalse = fotometria"
          n591 = flat-sequence {
            tunnel: w1486 -> [w1498]
            tunnel: [w1498] -> w1485
            frame #0 {
              n592 = local read "time3"() -> (w1500:u32)
              n593 = local read "time4"() -> (w1497:u32)
              n594 = Subtract(x=w1497, y=w1500) -> (x-y=→"delay 3-4":u32)
            }
          }
          n595 = call "Read Instrument.lvclass.vi"("error in (no error)"=w1485, "S4ACS_GUI in"=w1496) -> ("error out"=w1491:errorcluster, "Instrument.lvclass"=w1492:refnum<class "Instrument.lvclass">, "S4ACS_GUI out"=w1490:refnum<class "S4GUI.lvclass">)  [unwired: 7 in]
          n596 = call-dynamic "Read mode.vi"("error in (no error)"=w1491, "Instrument in"=w1492) -> ("error out"=w1487:errorcluster, "mode"=w1489:bool)  [unwired: 7 in, 1 out]
          n597 = disable-structure shown="Enabled" {
            disable-tunnel: [u32 321 ("t") u32 323 ("t")] -> w1488
            frame Disabled {
            }
            frame Enabled {
              # "\"Pula\" a configuração dos\ndelays e widths do SyncBox"
            }
          }
          n598 = Select(t=u32 301, s=w1489, f=w1488) -> (s? t:f=w1494:u32)
          n599 = Bundle By Name(cluster=w1490, "Obs_state"=w1494, "cyclesDone"=u32 0, "sequesDone"=u32 0) -> (w1495:refnum<class "S4GUI.lvclass">)
        }
        frame 301 {
          n600 = flat-sequence {
            tunnel: w1504 -> [w1544]
            tunnel: [w1544] -> w1503
            frame #0 {
              n601 = Tick Count (ms)() -> (millisecond timer value=→"time1":u32)
            }
          }
          n602 = call "Read Instrument.lvclass.vi"("error in (no error)"=w1503, "S4ACS_GUI in"=w1539) -> ("error out"=w1542:errorcluster, "Instrument.lvclass"=w1543:refnum<class "Instrument.lvclass">, "S4ACS_GUI out"=w1540:refnum<class "S4GUI.lvclass">)  [unwired: 7 in]
          n603 = call "Read WPROT.vi"("error in (no error)"=w1542, "Instrument in"=w1543) -> ("error out"=w1532:errorcluster, "Opt_Selector.lvclass"=w1533:refnum<class "Opt_Selector.lvclass">, "Instrument out"=w1541:refnum<class "Instrument.lvclass">)  [unwired: 7 in]
          n604 = call-dynamic "getTargetPos.vi"("error in (no error)"=w1532, "Opt_Selector in"=w1533) -> ("error out"=w1531:errorcluster, "Target Pos"=w1511:u16, "Opt_Selector out"=w1530:refnum<class "Opt_Selector.lvclass">)  [unwired: 7 in]
          n605 = Build Array(-1.0 ("element"), 0.0 ("element"), 22.5 ("element"), 45.0 ("element"), 67.5 ("element"), 90.0 ("element"), 112.5 ("element"), 135.0 ("element"), 157.5 ("element"), 180.0 ("element"), 202.5 ("element"), 225.0 ("element"), 247.5 ("element"), 270.0 ("element"), 292.5 ("element"), 315.0 ("element"), 337.5 ("element")) -> (w1523:dbl[])
          n606 = Index Array(array=w1523, index=w1511) -> (element=w1510:dbl)
          n607 = case shown="0, Default" w1511 {
            selector: w1511 -> [_ w1573]
            tunnel: w1541 -> [w1553 w1561]
            tunnel: [w1553 w1561] -> w1506
            tunnel: [w1550 w1560] -> w1505
            tunnel: w1536 -> [_ w1575]
            tunnel: [u32 311 w1574] -> w1535
            tunnel: w1531 -> [w1551 w1569]
            tunnel: w1530 -> [w1552 w1568]
            tunnel: w1510 -> [_ w1563]
            tunnel: [w1548 w1562] -> w1507
            frame 0, Default {
              # "Terminou uma sequência.\nRecupera as posições em SEQ e desvia para 311 para verificar se há mais ciclos."
              # "Recupera a sequencia anterior para o caso \nde repetição da sequencia (sem precisar clicar \nnas posicoes desejadas novamente)."
              n608 = call-dynamic "Read sequencia_ant.vi"("error in (no error)"=w1551, "Opt_Selector in"=w1552) -> ("error out"=w1547:errorcluster, "sequencia_ant"=w1546:u16, "Opt_Selector out"=w1549:refnum<class "Opt_Selector.lvclass">)  [unwired: 7 in]
              n609 = call-dynamic "Write sequencia.vi"("error in (no error)"=w1547, "sequencia"=w1546, "Opt_Selector in"=w1549) -> ("error out"=w1550:errorcluster, "Opt_Selector out"=w1548:refnum<class "Opt_Selector.lvclass">)  [unwired: 7 in]
            }
            frame 1..16 {
              # "Espera até 40 x 0.25s (= 10s) para\nmecanismo entrar em READY"
              n610 = Number To Decimal String(number=w1573) -> (decimal integer string=w1572:string)  [unwired: 1 in]
              n611 = Concatenate Strings("WP" ("string"), w1572) -> (w1570:string)
              n612 = call "Write target name.vi"("error in (no error)"=w1569, "target name"=w1570, "Optics in"=w1568) -> ("error out"=w1566:errorcluster, "Optics out"=w1567:refnum<class "Opt_Selector.lvclass">)  [unwired: 7 in]
              n613 = call "Write target.vi"("error in (no error)"=w1566, "target"=w1563, "Optics in"=w1567) -> ("error out"=w1565:errorcluster, "Optics out"=w1564:refnum<class "Opt_Selector.lvclass">)  [unwired: 7 in]
              n614 = call-dynamic "Read State Machine.vi"("error in (no error)"=w1565, "Device in"=w1564) -> ("error out"=w1577:errorcluster, "State Machine.lvclass"=w1579:refnum<class "State Machine.lvclass">, "Device out"=w1576:refnum<class "Opt_Selector.lvclass">)  [unwired: 7 in]
              n615 = Increment(x=w1575) -> (x+1=w1574:u32)
              n616 = call "Next State.vi"("error in (no error)"=w1577, "New_State"=1, "State Machine in"=w1579) -> ("error out"=w1557:errorcluster, "State Machine out"=w1559:refnum<class "State Machine.lvclass">)  [unwired: 7 in]
              n617 = call-dynamic "Write Timer.vi"("error in (no error)"=w1557, "Timer"=u32 40, "State Machine in"=w1559) -> ("error out"=w1556:errorcluster, "State Machine out"=w1558:refnum<class "State Machine.lvclass">)  [unwired: 7 in]
              n618 = call-dynamic "Write State Machine.vi"("error in (no error)"=w1556, "State Machine.lvclass"=w1558, "Device in"=w1576) -> ("error out"=w1560:errorcluster, "Device out"=w1562:refnum<class "Opt_Selector.lvclass">)  [unwired: 7 in]
            }
          }
          n619 = call "Write WPROT.vi"("error in (no error)"=w1505, "Opt_Selector.lvclass"=w1507, "Instrument in"=w1506) -> ("error out"=w1509:errorcluster, "Instrument out"=w1508:refnum<class "Instrument.lvclass">)  [unwired: 7 in]
          n620 = call "Write Instrument.lvclass.vi"("error in (no error)"=w1509, "Instrument.lvclass"=w1508, "S4ACS_GUI in"=w1540) -> ("error out"=w1538:errorcluster, "S4ACS_GUI out"=w1537:refnum<class "S4GUI.lvclass">)  [unwired: 7 in]
          n621 = Bundle By Name(cluster=w1537, "Obs_state"=w1535) -> (w1534:refnum<class "S4GUI.lvclass">)
        }
        frame 302 {
          # "Espera terminar o movimento da lamina para disparar a aquisição\ndos canais ativos.\n\nOV 20230424: Não precisa mais atualizar o valor de WPPOS com o\ncomando WRITE_HEADER porque o ACS já recebeu a sequência de\nposições da lâmina."
          n622 = flat-sequence {
            tunnel: w1594 -> [w1612]
            tunnel: [w1612] -> w1593
            frame #0 {
              n623 = Tick Count (ms)() -> (millisecond timer value=→"time 2":u32)
            }
          }
          n624 = call "Read Instrument.lvclass.vi"("error in (no error)"=w1593, "S4ACS_GUI in"=w1603) -> ("error out"=w1608:errorcluster, "Instrument.lvclass"=w1609:refnum<class "Instrument.lvclass">, "S4ACS_GUI out"=w1605:refnum<class "S4GUI.lvclass">)  [unwired: 7 in]
          n625 = call "Read WPROT.vi"("error in (no error)"=w1608, "Instrument in"=w1609) -> ("error out"=w1600:errorcluster, "Opt_Selector.lvclass"=w1599:refnum<class "Opt_Selector.lvclass">, "Instrument out"=w1607:refnum<class "Instrument.lvclass">)  [unwired: 7 in]
          n626 = call-dynamic "Read State Machine.vi"("error in (no error)"=w1600, "Device in"=w1599) -> ("error out"=w1601:errorcluster, "State Machine.lvclass"=w1602:refnum<class "State Machine.lvclass">, "Device out"=w1597:refnum<class "Opt_Selector.lvclass">)  [unwired: 7 in]
          n627 = call-dynamic "Read State.vi"("error in (no error)"=w1601, "State Machine in"=w1602) -> ("error out"=w1591:errorcluster, "State"=w1595:i32, "State Machine out"=w1592:refnum<class "State Machine.lvclass">)  [unwired: 7 in]
          n628 = Equal To 0?(x=w1595) -> (x = 0?=w1582:bool)
          n629 = call-dynamic "Write State Machine.vi"("error in (no error)"=w1591, "State Machine.lvclass"=w1592, "Device in"=w1597) -> ("error out"=w1596:errorcluster, "Device out"=w1598:refnum<class "Opt_Selector.lvclass">)  [unwired: 7 in]
          n630 = call "Write WPROT.vi"("error in (no error)"=w1596, "Opt_Selector.lvclass"=w1598, "Instrument in"=w1607) -> ("error out"=w1604:errorcluster, "Instrument out"=w1606:refnum<class "Instrument.lvclass">)  [unwired: 7 in]
          n631 = call "Write Instrument.lvclass.vi"("error in (no error)"=w1604, "Instrument.lvclass"=w1606, "S4ACS_GUI in"=w1605) -> ("error out"=w1580:errorcluster, "S4ACS_GUI out"=w1583:refnum<class "S4GUI.lvclass">)  [unwired: 7 in]
          n632 = Unbundle By Name(w1583) -> ("cyclesDone"=w1587:u32, "sequesDone"=w1586:u32)
          n633 = Add(x=w1587, y=w1586) -> (x+y=w1585:u32)
          n634 = Equal To 0?(x=w1585) -> (x = 0?=w1588:bool)
          n635 = case shown="False" w1588 {
            tunnel: [u32 308 ("t") u32 306 ("t")] -> w1589
            frame False {
              # "Não é 1a seq:\nvai direto para\nenvio do trigger"
            }
            frame True {
              # "1a sequencia:\nenvia EXPOSE"
            }
          }
          n636 = Select(t=w1589, s=w1582, f=w1581) -> (s? t:f=w1590:u32)
          n637 = Bundle By Name(cluster=w1583, "Obs_state"=w1590) -> (w1584:refnum<class "S4GUI.lvclass">)
        }
        frame 306 {
          n638 = call-dynamic "Read AcquisitionA.vi"("error in (no error)"=w1654, "S4ACS_GUI in"=w1655) -> ("error out"=w1630:errorcluster, "Acquisition.lvclass"=w1633:refnum<class "Acquisition.lvclass">, "S4ACS_GUI out"=w1657:refnum<class "S4GUI.lvclass">)  [unwired: 7 in]
          n639 = call "Read connection.vi"("error in (no error)"=w1630, "Server in"=w1633) -> ("error out"=w1629:errorcluster, "connection"=w1631:bool, "Server out"=w1632:refnum<class "Acquisition.lvclass">)  [unwired: 7 in]
          n640 = case shown="True" w1631 {
            tunnel: w1632 -> [w1711 w1726]
            tunnel: w1629 -> [w1710 w1725]
            tunnel: [w1711 w1723] -> w1658
            tunnel: [w1710 w1722] -> w1656
            frame False {
            }
            frame True {
              n641 = call-dynamic "Read Channel.vi"("error in (no error)"=w1725, "Acquisition in"=w1726) -> ("error out"=w1718:errorcluster, "Channel.lvclass"=w1717:refnum<class "Channel.lvclass">, "Acquisition out"=w1724:refnum<class "Acquisition.lvclass">)  [unwired: 7 in]
              n642 = call-dynamic "Read State Machine.vi"("error in (no error)"=w1718, "Device in"=w1717) -> ("error out"=w1719:errorcluster, "State Machine.lvclass"=w1721:refnum<class "State Machine.lvclass">, "Device out"=w1715:refnum<class "Channel.lvclass">)  [unwired: 7 in]
              n643 = call "Next State.vi"("error in (no error)"=w1719, "New_State"=50, "State Machine in"=w1721) -> ("error out"=w1712:errorcluster, "State Machine out"=w1713:refnum<class "State Machine.lvclass">)  [unwired: 7 in]
              n644 = call-dynamic "Write State Machine.vi"("error in (no error)"=w1712, "State Machine.lvclass"=w1713, "Device in"=w1715) -> ("error out"=w1714:errorcluster, "Device out"=w1716:refnum<class "Channel.lvclass">)  [unwired: 7 in]
              n645 = call-dynamic "Write Channel.vi"("error in (no error)"=w1714, "Channel.lvclass"=w1716, "Acquisition in"=w1724) -> ("error out"=w1722:errorcluster, "Acquisition out"=w1723:refnum<class "Acquisition.lvclass">)  [unwired: 7 in]
            }
          }
          n646 = call-dynamic "Write AcquisitionA.vi"("error in (no error)"=w1656, "Acquisition.lvclass"=w1658, "S4ACS_GUI in"=w1657) -> ("error out"=w1649:errorcluster, "S4ACS_GUI out"=w1650:refnum<class "S4GUI.lvclass">)  [unwired: 7 in]
          n647 = call "Read AcquisitionB.vi"("error in (no error)"=w1649, "S4ACS_GUI in"=w1650) -> ("error out"=w1626:errorcluster, "Acquisition.lvclass"=w1628:refnum<class "Acquisition.lvclass">, "S4ACS_GUI out"=w1647:refnum<class "S4GUI.lvclass">)  [unwired: 7 in]
          n648 = call "Read connection.vi"("error in (no error)"=w1626, "Server in"=w1628) -> ("error out"=w1625:errorcluster, "connection"=w1624:bool, "Server out"=w1627:refnum<class "Acquisition.lvclass">)  [unwired: 7 in]
          n649 = case shown="True" w1624 {
            tunnel: w1627 -> [w1694 w1709]
            tunnel: w1625 -> [w1693 w1708]
            tunnel: [w1694 w1706] -> w1648
            tunnel: [w1693 w1705] -> w1646
            frame False {
            }
            frame True {
              n650 = call-dynamic "Read Channel.vi"("error in (no error)"=w1708, "Acquisition in"=w1709) -> ("error out"=w1701:errorcluster, "Channel.lvclass"=w1700:refnum<class "Channel.lvclass">, "Acquisition out"=w1707:refnum<class "Acquisition.lvclass">)  [unwired: 7 in]
              n651 = call-dynamic "Read State Machine.vi"("error in (no error)"=w1701, "Device in"=w1700) -> ("error out"=w1702:errorcluster, "State Machine.lvclass"=w1704:refnum<class "State Machine.lvclass">, "Device out"=w1698:refnum<class "Channel.lvclass">)  [unwired: 7 in]
              n652 = call "Next State.vi"("error in (no error)"=w1702, "New_State"=50, "State Machine in"=w1704) -> ("error out"=w1695:errorcluster, "State Machine out"=w1696:refnum<class "State Machine.lvclass">)  [unwired: 7 in]
              n653 = call-dynamic "Write State Machine.vi"("error in (no error)"=w1695, "State Machine.lvclass"=w1696, "Device in"=w1698) -> ("error out"=w1697:errorcluster, "Device out"=w1699:refnum<class "Channel.lvclass">)  [unwired: 7 in]
              n654 = call-dynamic "Write Channel.vi"("error in (no error)"=w1697, "Channel.lvclass"=w1699, "Acquisition in"=w1707) -> ("error out"=w1705:errorcluster, "Acquisition out"=w1706:refnum<class "Acquisition.lvclass">)  [unwired: 7 in]
            }
          }
          n655 = call "Write AcquisitionB.vi"("error in (no error)"=w1646, "Acquisition.lvclass"=w1648, "S4ACS_GUI in"=w1647) -> ("error out"=w1642:errorcluster, "S4ACS_GUI out"=w1641:refnum<class "S4GUI.lvclass">)  [unwired: 7 in]
          n656 = call-dynamic "Read AcquisitionC.vi"("error in (no error)"=w1642, "S4ACS_GUI in"=w1641) -> ("error out"=w1621:errorcluster, "Acquisition.lvclass"=w1623:refnum<class "Acquisition.lvclass">, "S4ACS_GUI out"=w1644:refnum<class "S4GUI.lvclass">)  [unwired: 7 in]
          n657 = call "Read connection.vi"("error in (no error)"=w1621, "Server in"=w1623) -> ("error out"=w1620:errorcluster, "connection"=w1619:bool, "Server out"=w1622:refnum<class "Acquisition.lvclass">)  [unwired: 7 in]
          n658 = case shown="True" w1619 {
            tunnel: [w1676 w1684] -> w1645
            tunnel: [w1677 w1683] -> w1643
            tunnel: w1622 -> [w1677 w1681]
            tunnel: w1620 -> [w1676 w1680]
            frame False {
            }
            frame True {
              n659 = call-dynamic "Read Channel.vi"("error in (no error)"=w1680, "Acquisition in"=w1681) -> ("error out"=w1688:errorcluster, "Channel.lvclass"=w1689:refnum<class "Channel.lvclass">, "Acquisition out"=w1682:refnum<class "Acquisition.lvclass">)  [unwired: 7 in]
              n660 = call-dynamic "Read State Machine.vi"("error in (no error)"=w1688, "Device in"=w1689) -> ("error out"=w1687:errorcluster, "State Machine.lvclass"=w1685:refnum<class "State Machine.lvclass">, "Device out"=w1691:refnum<class "Channel.lvclass">)  [unwired: 7 in]
              n661 = call "Next State.vi"("error in (no error)"=w1687, "New_State"=50, "State Machine in"=w1685) -> ("error out"=w1679:errorcluster, "State Machine out"=w1678:refnum<class "State Machine.lvclass">)  [unwired: 7 in]
              n662 = call-dynamic "Write State Machine.vi"("error in (no error)"=w1679, "State Machine.lvclass"=w1678, "Device in"=w1691) -> ("error out"=w1692:errorcluster, "Device out"=w1690:refnum<class "Channel.lvclass">)  [unwired: 7 in]
              n663 = call-dynamic "Write Channel.vi"("error in (no error)"=w1692, "Channel.lvclass"=w1690, "Acquisition in"=w1682) -> ("error out"=w1684:errorcluster, "Acquisition out"=w1683:refnum<class "Acquisition.lvclass">)  [unwired: 7 in]
            }
          }
          n664 = call-dynamic "Write AcquisitionC.vi"("error in (no error)"=w1645, "Acquisition.lvclass"=w1643, "S4ACS_GUI in"=w1644) -> ("error out"=w1639:errorcluster, "S4ACS_GUI out"=w1638:refnum<class "S4GUI.lvclass">)  [unwired: 7 in]
          n665 = call-dynamic "Read AcquisitionD.vi"("error in (no error)"=w1639, "S4ACS_GUI in"=w1638) -> ("error out"=w1616:errorcluster, "Acquisition.lvclass"=w1618:refnum<class "Acquisition.lvclass">, "S4ACS_GUI out"=w1637:refnum<class "S4GUI.lvclass">)  [unwired: 7 in]
          n666 = call "Read connection.vi"("error in (no error)"=w1616, "Server in"=w1618) -> ("error out"=w1615:errorcluster, "connection"=w1614:bool, "Server out"=w1617:refnum<class "Acquisition.lvclass">)  [unwired: 7 in]
          n667 = case shown="True" w1614 {
            tunnel: w1615 -> [w1659 w1675]
            tunnel: [w1659 w1674] -> w1640
            tunnel: w1617 -> [w1660 w1665]
            tunnel: [w1660 w1663] -> w1636
            frame False {
            }
            frame True {
              n668 = call-dynamic "Read Channel.vi"("error in (no error)"=w1675, "Acquisition in"=w1665) -> ("error out"=w1670:errorcluster, "Channel.lvclass"=w1669:refnum<class "Channel.lvclass">, "Acquisition out"=w1664:refnum<class "Acquisition.lvclass">)  [unwired: 7 in]
              n669 = call-dynamic "Read State Machine.vi"("error in (no error)"=w1670, "Device in"=w1669) -> ("error out"=w1671:errorcluster, "State Machine.lvclass"=w1673:refnum<class "State Machine.lvclass">, "Device out"=w1667:refnum<class "Channel.lvclass">)  [unwired: 7 in]
              n670 = call "Next State.vi"("error in (no error)"=w1671, "New_State"=50, "State Machine in"=w1673) -> ("error out"=w1661:errorcluster, "State Machine out"=w1662:refnum<class "State Machine.lvclass">)  [unwired: 7 in]
              n671 = call-dynamic "Write State Machine.vi"("error in (no error)"=w1661, "State Machine.lvclass"=w1662, "Device in"=w1667) -> ("error out"=w1666:errorcluster, "Device out"=w1668:refnum<class "Channel.lvclass">)  [unwired: 7 in]
              n672 = call-dynamic "Write Channel.vi"("error in (no error)"=w1666, "Channel.lvclass"=w1668, "Acquisition in"=w1664) -> ("error out"=w1674:errorcluster, "Acquisition out"=w1663:refnum<class "Acquisition.lvclass">)  [unwired: 7 in]
            }
          }
          n673 = call-dynamic "Write AcquisitionD.vi"("error in (no error)"=w1640, "Acquisition.lvclass"=w1636, "S4ACS_GUI in"=w1637) -> ("error out"=w1635:errorcluster, "S4ACS_GUI out"=w1634:refnum<class "S4GUI.lvclass">)  [unwired: 7 in]
          n674 = Increment(x=w1653) -> (x+1=w1652:u32)
          n675 = Bundle By Name(cluster=w1634, "Obs_state"=w1652) -> (w1651:refnum<class "S4GUI.lvclass">)
        }
        frame 307 {
          # "Espera todos os canais chegarem ao estado ACTIVE\n(estados 54 e 55 de Channel:Run.vi)."
          n676 = call-dynamic "Read AcquisitionA.vi"("error in (no error)"=w1773, "S4ACS_GUI in"=w1774) -> ("error out"=w1750:errorcluster, "Acquisition.lvclass"=w1751:refnum<class "Acquisition.lvclass">, "S4ACS_GUI out"=w1776:refnum<class "S4GUI.lvclass">)  [unwired: 7 in]
          n677 = call "Read connection.vi"("error in (no error)"=w1750, "Server in"=w1751) -> ("error out"=w1752:errorcluster, "connection"=w1754:bool, "Server out"=w1753:refnum<class "Acquisition.lvclass">)  [unwired: 7 in]
          n678 = case shown="True" w1754 {
            tunnel: [w1840 w1856] -> w1777
            tunnel: [w1839 w1855] -> w1775
            tunnel: w1753 -> [w1840 w1845]
            tunnel: w1752 -> [w1839 w1844]
            tunnel: [TRUE w1843] -> w1730
            frame False {
            }
            frame True {
              n679 = call-dynamic "Read Channel.vi"("error in (no error)"=w1844, "Acquisition in"=w1845) -> ("error out"=w1854:errorcluster, "Channel.lvclass"=w1853:refnum<class "Channel.lvclass">, "Acquisition out"=w1857:refnum<class "Acquisition.lvclass">)  [unwired: 7 in]
              n680 = call-dynamic "Read State Machine.vi"("error in (no error)"=w1854, "Device in"=w1853) -> ("error out"=w1847:errorcluster, "State Machine.lvclass"=w1849:refnum<class "State Machine.lvclass">, "Device out"=w1851:refnum<class "Channel.lvclass">)  [unwired: 7 in]
              n681 = call-dynamic "Read State.vi"("error in (no error)"=w1847, "State Machine in"=w1849) -> ("error out"=w1846:errorcluster, "State"=w1842:i32, "State Machine out"=w1848:refnum<class "State Machine.lvclass">)  [unwired: 7 in]
              n682 = Greater?(x=w1842, y=53) -> (0:w1843:bool)
              n683 = call-dynamic "Write State Machine.vi"("error in (no error)"=w1846, "State Machine.lvclass"=w1848, "Device in"=w1851) -> ("error out"=w1850:errorcluster, "Device out"=w1852:refnum<class "Channel.lvclass">)  [unwired: 7 in]
              n684 = call-dynamic "Write Channel.vi"("error in (no error)"=w1850, "Channel.lvclass"=w1852, "Acquisition in"=w1857) -> ("error out"=w1855:errorcluster, "Acquisition out"=w1856:refnum<class "Acquisition.lvclass">)  [unwired: 7 in]
            }
          }
          n685 = call-dynamic "Write AcquisitionA.vi"("error in (no error)"=w1775, "Acquisition.lvclass"=w1777, "S4ACS_GUI in"=w1776) -> ("error out"=w1769:errorcluster, "S4ACS_GUI out"=w1770:refnum<class "S4GUI.lvclass">)  [unwired: 7 in]
          n686 = call "Read AcquisitionB.vi"("error in (no error)"=w1769, "S4ACS_GUI in"=w1770) -> ("error out"=w1747:errorcluster, "Acquisition.lvclass"=w1749:refnum<class "Acquisition.lvclass">, "S4ACS_GUI out"=w1767:refnum<class "S4GUI.lvclass">)  [unwired: 7 in]
          n687 = call "Read connection.vi"("error in (no error)"=w1747, "Server in"=w1749) -> ("error out"=w1746:errorcluster, "connection"=w1745:bool, "Server out"=w1748:refnum<class "Acquisition.lvclass">)  [unwired: 7 in]
          n688 = case shown="True" w1745 {
            tunnel: w1748 -> [w1820 w1837]
            tunnel: w1746 -> [w1819 w1836]
            tunnel: [w1820 w1834] -> w1768
            tunnel: [w1819 w1833] -> w1766
            tunnel: [TRUE w1822] -> w1729
            frame False {
            }
            frame True {
              n689 = call-dynamic "Read Channel.vi"("error in (no error)"=w1836, "Acquisition in"=w1837) -> ("error out"=w1832:errorcluster, "Channel.lvclass"=w1831:refnum<class "Channel.lvclass">, "Acquisition out"=w1835:refnum<class "Acquisition.lvclass">)  [unwired: 7 in]
              n690 = call-dynamic "Read State Machine.vi"("error in (no error)"=w1832, "Device in"=w1831) -> ("error out"=w1825:errorcluster, "State Machine.lvclass"=w1827:refnum<class "State Machine.lvclass">, "Device out"=w1829:refnum<class "Channel.lvclass">)  [unwired: 7 in]
              n691 = call-dynamic "Read State.vi"("error in (no error)"=w1825, "State Machine in"=w1827) -> ("error out"=w1824:errorcluster, "State"=w1821:i32, "State Machine out"=w1826:refnum<class "State Machine.lvclass">)  [unwired: 7 in]
              n692 = Greater?(x=w1821, y=53) -> (0:w1822:bool)
              n693 = call-dynamic "Write State Machine.vi"("error in (no error)"=w1824, "State Machine.lvclass"=w1826, "Device in"=w1829) -> ("error out"=w1828:errorcluster, "Device out"=w1830:refnum<class "Channel.lvclass">)  [unwired: 7 in]
              n694 = call-dynamic "Write Channel.vi"("error in (no error)"=w1828, "Channel.lvclass"=w1830, "Acquisition in"=w1835) -> ("error out"=w1833:errorcluster, "Acquisition out"=w1834:refnum<class "Acquisition.lvclass">)  [unwired: 7 in]
            }
          }
          n695 = call "Write AcquisitionB.vi"("error in (no error)"=w1766, "Acquisition.lvclass"=w1768, "S4ACS_GUI in"=w1767) -> ("error out"=w1762:errorcluster, "S4ACS_GUI out"=w1761:refnum<class "S4GUI.lvclass">)  [unwired: 7 in]
          n696 = call-dynamic "Read AcquisitionC.vi"("error in (no error)"=w1762, "S4ACS_GUI in"=w1761) -> ("error out"=w1742:errorcluster, "Acquisition.lvclass"=w1744:refnum<class "Acquisition.lvclass">, "S4ACS_GUI out"=w1764:refnum<class "S4GUI.lvclass">)  [unwired: 7 in]
          n697 = call "Read connection.vi"("error in (no error)"=w1742, "Server in"=w1744) -> ("error out"=w1741:errorcluster, "connection"=w1740:bool, "Server out"=w1743:refnum<class "Acquisition.lvclass">)  [unwired: 7 in]
          n698 = case shown="True" w1740 {
            tunnel: [w1799 w1810] -> w1765
            tunnel: [w1800 w1809] -> w1763
            tunnel: w1743 -> [w1800 w1805]
            tunnel: w1741 -> [w1799 w1804]
            tunnel: [TRUE w1801] -> w1728
            frame False {
            }
            frame True {
              n699 = call-dynamic "Read Channel.vi"("error in (no error)"=w1804, "Acquisition in"=w1805) -> ("error out"=w1811:errorcluster, "Channel.lvclass"=w1812:refnum<class "Channel.lvclass">, "Acquisition out"=w1808:refnum<class "Acquisition.lvclass">)  [unwired: 7 in]
              n700 = call-dynamic "Read State Machine.vi"("error in (no error)"=w1811, "Device in"=w1812) -> ("error out"=w1806:errorcluster, "State Machine.lvclass"=w1816:refnum<class "State Machine.lvclass">, "Device out"=w1814:refnum<class "Channel.lvclass">)  [unwired: 7 in]
              n701 = call-dynamic "Read State.vi"("error in (no error)"=w1806, "State Machine in"=w1816) -> ("error out"=w1807:errorcluster, "State"=w1802:i32, "State Machine out"=w1817:refnum<class "State Machine.lvclass">)  [unwired: 7 in]
              n702 = Greater?(x=w1802, y=53) -> (0:w1801:bool)
              n703 = call-dynamic "Write State Machine.vi"("error in (no error)"=w1807, "State Machine.lvclass"=w1817, "Device in"=w1814) -> ("error out"=w1815:errorcluster, "Device out"=w1813:refnum<class "Channel.lvclass">)  [unwired: 7 in]
              n704 = call-dynamic "Write Channel.vi"("error in (no error)"=w1815, "Channel.lvclass"=w1813, "Acquisition in"=w1808) -> ("error out"=w1810:errorcluster, "Acquisition out"=w1809:refnum<class "Acquisition.lvclass">)  [unwired: 7 in]
            }
          }
          n705 = call-dynamic "Write AcquisitionC.vi"("error in (no error)"=w1765, "Acquisition.lvclass"=w1763, "S4ACS_GUI in"=w1764) -> ("error out"=w1739:errorcluster, "S4ACS_GUI out"=w1757:refnum<class "S4GUI.lvclass">)  [unwired: 7 in]
          n706 = call-dynamic "Read AcquisitionD.vi"("error in (no error)"=w1739, "S4ACS_GUI in"=w1757) -> ("error out"=w1735:errorcluster, "Acquisition.lvclass"=w1738:refnum<class "Acquisition.lvclass">, "S4ACS_GUI out"=w1759:refnum<class "S4GUI.lvclass">)  [unwired: 7 in]
          n707 = call "Read connection.vi"("error in (no error)"=w1735, "Server in"=w1738) -> ("error out"=w1736:errorcluster, "connection"=w1734:bool, "Server out"=w1737:refnum<class "Acquisition.lvclass">)  [unwired: 7 in]
          n708 = case shown="True" w1734 {
            tunnel: [w1780 w1796] -> w1760
            tunnel: [w1779 w1795] -> w1758
            tunnel: [TRUE w1782] -> w1727
            tunnel: w1737 -> [w1780 w1785]
            tunnel: w1736 -> [w1779 w1784]
            frame False {
            }
            frame True {
              n709 = call-dynamic "Read Channel.vi"("error in (no error)"=w1784, "Acquisition in"=w1785) -> ("error out"=w1794:errorcluster, "Channel.lvclass"=w1793:refnum<class "Channel.lvclass">, "Acquisition out"=w1797:refnum<class "Acquisition.lvclass">)  [unwired: 7 in]
              n710 = call-dynamic "Read State Machine.vi"("error in (no error)"=w1794, "Device in"=w1793) -> ("error out"=w1787:errorcluster, "State Machine.lvclass"=w1789:refnum<class "State Machine.lvclass">, "Device out"=w1791:refnum<class "Channel.lvclass">)  [unwired: 7 in]
              n711 = call-dynamic "Read State.vi"("error in (no error)"=w1787, "State Machine in"=w1789) -> ("error out"=w1786:errorcluster, "State"=w1781:i32, "State Machine out"=w1788:refnum<class "State Machine.lvclass">)  [unwired: 7 in]
              n712 = Greater?(x=w1781, y=53) -> (0:w1782:bool)
              n713 = call-dynamic "Write State Machine.vi"("error in (no error)"=w1786, "State Machine.lvclass"=w1788, "Device in"=w1791) -> ("error out"=w1790:errorcluster, "Device out"=w1792:refnum<class "Channel.lvclass">)  [unwired: 7 in]
              n714 = call-dynamic "Write Channel.vi"("error in (no error)"=w1790, "Channel.lvclass"=w1792, "Acquisition in"=w1797) -> ("error out"=w1795:errorcluster, "Acquisition out"=w1796:refnum<class "Acquisition.lvclass">)  [unwired: 7 in]
            }
          }
          n715 = call-dynamic "Write AcquisitionD.vi"("error in (no error)"=w1758, "Acquisition.lvclass"=w1760, "S4ACS_GUI in"=w1759) -> ("error out"=w1755:errorcluster, "S4ACS_GUI out"=w1756:refnum<class "S4GUI.lvclass">)  [unwired: 7 in]
          n716 = Compound Arithmetic op=AND(w1730, w1729, w1728, w1727) -> (w1731:bool)
          n717 = Increment(x=w1733) -> (x+1=w1732:u32)
          n718 = Select(t=w1732, s=w1731, f=w1733) -> (s? t:f=w1771:u32)
          n719 = Bundle By Name(cluster=w1756, "Obs_state"=w1771) -> (w1772:refnum<class "S4GUI.lvclass">)
        }
        frame 308 {
          n720 = call-dynamic "Read Sync Box.lvclass.vi"("error in (no error)"=w1870, "SPARC4_AC in"=w1871) -> ("error out"=w1862:errorcluster, "Sync Box.lvclass"=w1864:refnum<class "Sync Box.lvclass">, "SPARC4_AC out"=w1859:refnum<class "S4GUI.lvclass">)  [unwired: 7 in]
          n721 = call "Read connection.vi"("error in (no error)"=w1862, "Server in"=w1864) -> ("error out"=w1861:errorcluster, "connection"=w1860:bool, "Server out"=w1863:refnum<class "Sync Box.lvclass">)  [unwired: 7 in]
          n722 = case shown="True" w1860 {
            tunnel: w1861 -> [w1878 w1899]
            tunnel: [w1879 w1897] -> w1873
            tunnel: [w1878 w1880] -> w1872
            tunnel: w1867 -> [w1877 w1888]
            tunnel: [w1875 w1887] -> w1866
            tunnel: w1863 -> [w1879 w1886]
            tunnel: w1859 -> [w1874 w1883]
            tunnel: [w1874 w1881] -> w1858
            frame False {
              n723 = Increment(x=w1877) -> (x+1=w1876:u32)
              n724 = Increment(x=w1876) -> (x+1=w1875:u32)
            }
            frame True {
              # "Envia comando FIRE para o SyncBox"
              n725 = call-dynamic "Read Trigger.lvclass.vi"("error in (no error)"=w1899, "Sync Box in"=w1886) -> ("error out"=w1893:errorcluster, "Trigger.lvclass"=w1892:refnum<class "Trigger.lvclass">, "Sync Box out"=w1898:refnum<class "Sync Box.lvclass">)  [unwired: 7 in]
              n726 = call-dynamic "Read State Machine.vi"("error in (no error)"=w1893, "Device in"=w1892) -> ("error out"=w1894:errorcluster, "State Machine.lvclass"=w1896:refnum<class "State Machine.lvclass">, "Device out"=w1890:refnum<class "Trigger.lvclass">)  [unwired: 7 in]
              n727 = call "Next State.vi"("error in (no error)"=w1894, "New_State"=40, "State Machine in"=w1896) -> ("error out"=w1884:errorcluster, "State Machine out"=w1885:refnum<class "State Machine.lvclass">)  [unwired: 7 in]
              n728 = call-dynamic "Write State Machine.vi"("error in (no error)"=w1884, "State Machine.lvclass"=w1885, "Device in"=w1890) -> ("error out"=w1889:errorcluster, "Device out"=w1891:refnum<class "Trigger.lvclass">)  [unwired: 7 in]
              n729 = Increment(x=w1888) -> (x+1=w1887:u32)
              n730 = call-dynamic "Write Trigger.lvclass.vi"("error in (no error)"=w1889, "Trigger.lvclass"=w1891, "Sync Box in"=w1898) -> ("error out"=w1882:errorcluster, "Sync Box out"=w1897:refnum<class "Sync Box.lvclass">)  [unwired: 7 in]
              n731 = disable-structure shown="Enabled" {
                disable-tunnel: w1883 -> [w1903 w2011]
                disable-tunnel: w1882 -> [w1902 w2010]
                disable-tunnel: [w1901 w2011] -> w1881
                disable-tunnel: [w1900 w2010] -> w1880
                frame Disabled {
                  n732 = call-dynamic "Read AcquisitionA.vi"("error in (no error)"=w1902, "S4ACS_GUI in"=w1903) -> ("error out"=w1920:errorcluster, "Acquisition.lvclass"=w1923:refnum<class "Acquisition.lvclass">, "S4ACS_GUI out"=w1940:refnum<class "S4GUI.lvclass">)  [unwired: 7 in]
                  n733 = call "Read connection.vi"("error in (no error)"=w1920, "Server in"=w1923) -> ("error out"=w1919:errorcluster, "connection"=w1921:bool, "Server out"=w1922:refnum<class "Acquisition.lvclass">)  [unwired: 7 in]
                  n734 = case shown="True" w1921 {
                    tunnel: w1922 -> [w1994 w2009]
                    tunnel: w1919 -> [w1993 w2008]
                    tunnel: [w1994 w2006] -> w1941
                    tunnel: [w1993 w2005] -> w1939
                    frame False {
                    }
                    frame True {
                      # "Envia comando TRIGGER_DONE  para o Acquisition"
                      n735 = call-dynamic "Read Channel.vi"("error in (no error)"=w2008, "Acquisition in"=w2009) -> ("error out"=w2001:errorcluster, "Channel.lvclass"=w2000:refnum<class "Channel.lvclass">, "Acquisition out"=w2007:refnum<class "Acquisition.lvclass">)  [unwired: 7 in]
                      n736 = call-dynamic "Read State Machine.vi"("error in (no error)"=w2001, "Device in"=w2000) -> ("error out"=w2002:errorcluster, "State Machine.lvclass"=w2004:refnum<class "State Machine.lvclass">, "Device out"=w1998:refnum<class "Channel.lvclass">)  [unwired: 7 in]
                      n737 = call "Next State.vi"("error in (no error)"=w2002, "New_State"=40, "State Machine in"=w2004) -> ("error out"=w1995:errorcluster, "State Machine out"=w1996:refnum<class "State Machine.lvclass">)  [unwired: 7 in]
                      n738 = call-dynamic "Write State Machine.vi"("error in (no error)"=w1995, "State Machine.lvclass"=w1996, "Device in"=w1998) -> ("error out"=w1997:errorcluster, "Device out"=w1999:refnum<class "Channel.lvclass">)  [unwired: 7 in]
                      n739 = call-dynamic "Write Channel.vi"("error in (no error)"=w1997, "Channel.lvclass"=w1999, "Acquisition in"=w2007) -> ("error out"=w2005:errorcluster, "Acquisition out"=w2006:refnum<class "Acquisition.lvclass">)  [unwired: 7 in]
                    }
                  }
                  n740 = call-dynamic "Write AcquisitionA.vi"("error in (no error)"=w1939, "Acquisition.lvclass"=w1941, "S4ACS_GUI in"=w1940) -> ("error out"=w1937:errorcluster, "S4ACS_GUI out"=w1938:refnum<class "S4GUI.lvclass">)  [unwired: 7 in]
                  n741 = call "Read AcquisitionB.vi"("error in (no error)"=w1937, "S4ACS_GUI in"=w1938) -> ("error out"=w1916:errorcluster, "Acquisition.lvclass"=w1918:refnum<class "Acquisition.lvclass">, "S4ACS_GUI out"=w1935:refnum<class "S4GUI.lvclass">)  [unwired: 7 in]
                  n742 = call "Read connection.vi"("error in (no error)"=w1916, "Server in"=w1918) -> ("error out"=w1915:errorcluster, "connection"=w1914:bool, "Server out"=w1917:refnum<class "Acquisition.lvclass">)  [unwired: 7 in]
                  n743 = case shown="True" w1914 {
                    tunnel: w1917 -> [w1977 w1992]
                    tunnel: w1915 -> [w1976 w1991]
                    tunnel: [w1977 w1989] -> w1936
                    tunnel: [w1976 w1988] -> w1934
                    frame False {
                    }
                    frame True {
                      # "Envia comando TRIGGER_DONE  para o Acquisition"
                      n744 = call-dynamic "Read Channel.vi"("error in (no error)"=w1991, "Acquisition in"=w1992) -> ("error out"=w1984:errorcluster, "Channel.lvclass"=w1983:refnum<class "Channel.lvclass">, "Acquisition out"=w1990:refnum<class "Acquisition.lvclass">)  [unwired: 7 in]
                      n745 = call-dynamic "Read State Machine.vi"("error in (no error)"=w1984, "Device in"=w1983) -> ("error out"=w1985:errorcluster, "State Machine.lvclass"=w1987:refnum<class "State Machine.lvclass">, "Device out"=w1981:refnum<class "Channel.lvclass">)  [unwired: 7 in]
                      n746 = call "Next State.vi"("error in (no error)"=w1985, "New_State"=40, "State Machine in"=w1987) -> ("error out"=w1978:errorcluster, "State Machine out"=w1979:refnum<class "State Machine.lvclass">)  [unwired: 7 in]
                      n747 = call-dynamic "Write State Machine.vi"("error in (no error)"=w1978, "State Machine.lvclass"=w1979, "Device in"=w1981) -> ("error out"=w1980:errorcluster, "Device out"=w1982:refnum<class "Channel.lvclass">)  [unwired: 7 in]
                      n748 = call-dynamic "Write Channel.vi"("error in (no error)"=w1980, "Channel.lvclass"=w1982, "Acquisition in"=w1990) -> ("error out"=w1988:errorcluster, "Acquisition out"=w1989:refnum<class "Acquisition.lvclass">)  [unwired: 7 in]
                    }
                  }
                  n749 = call "Write AcquisitionB.vi"("error in (no error)"=w1934, "Acquisition.lvclass"=w1936, "S4ACS_GUI in"=w1935) -> ("error out"=w1930:errorcluster, "S4ACS_GUI out"=w1929:refnum<class "S4GUI.lvclass">)  [unwired: 7 in]
                  n750 = call-dynamic "Read AcquisitionC.vi"("error in (no error)"=w1930, "S4ACS_GUI in"=w1929) -> ("error out"=w1911:errorcluster, "Acquisition.lvclass"=w1913:refnum<class "Acquisition.lvclass">, "S4ACS_GUI out"=w1932:refnum<class "S4GUI.lvclass">)  [unwired: 7 in]
                  n751 = call "Read connection.vi"("error in (no error)"=w1911, "Server in"=w1913) -> ("error out"=w1910:errorcluster, "connection"=w1909:bool, "Server out"=w1912:refnum<class "Acquisition.lvclass">)  [unwired: 7 in]
                  n752 = case shown="True" w1909 {
                    tunnel: [w1959 w1967] -> w1933
                    tunnel: [w1960 w1966] -> w1931
                    tunnel: w1912 -> [w1960 w1964]
                    tunnel: w1910 -> [w1959 w1963]
                    frame False {
                    }
                    frame True {
                      # "Envia comando TRIGGER_DONE  para o Acquisition"
                      n753 = call-dynamic "Read Channel.vi"("error in (no error)"=w1963, "Acquisition in"=w1964) -> ("error out"=w1971:errorcluster, "Channel.lvclass"=w1972:refnum<class "Channel.lvclass">, "Acquisition out"=w1965:refnum<class "Acquisition.lvclass">)  [unwired: 7 in]
                      n754 = call-dynamic "Read State Machine.vi"("error in (no error)"=w1971, "Device in"=w1972) -> ("error out"=w1970:errorcluster, "State Machine.lvclass"=w1968:refnum<class "State Machine.lvclass">, "Device out"=w1974:refnum<class "Channel.lvclass">)  [unwired: 7 in]
                      n755 = call "Next State.vi"("error in (no error)"=w1970, "New_State"=40, "State Machine in"=w1968) -> ("error out"=w1962:errorcluster, "State Machine out"=w1961:refnum<class "State Machine.lvclass">)  [unwired: 7 in]
                      n756 = call-dynamic "Write State Machine.vi"("error in (no error)"=w1962, "State Machine.lvclass"=w1961, "Device in"=w1974) -> ("error out"=w1975:errorcluster, "Device out"=w1973:refnum<class "Channel.lvclass">)  [unwired: 7 in]
                      n757 = call-dynamic "Write Channel.vi"("error in (no error)"=w1975, "Channel.lvclass"=w1973, "Acquisition in"=w1965) -> ("error out"=w1967:errorcluster, "Acquisition out"=w1966:refnum<class "Acquisition.lvclass">)  [unwired: 7 in]
                    }
                  }
                  n758 = call-dynamic "Write AcquisitionC.vi"("error in (no error)"=w1933, "Acquisition.lvclass"=w1931, "S4ACS_GUI in"=w1932) -> ("error out"=w1927:errorcluster, "S4ACS_GUI out"=w1926:refnum<class "S4GUI.lvclass">)  [unwired: 7 in]
                  n759 = call-dynamic "Read AcquisitionD.vi"("error in (no error)"=w1927, "S4ACS_GUI in"=w1926) -> ("error out"=w1906:errorcluster, "Acquisition.lvclass"=w1908:refnum<class "Acquisition.lvclass">, "S4ACS_GUI out"=w1925:refnum<class "S4GUI.lvclass">)  [unwired: 7 in]
                  n760 = call "Read connection.vi"("error in (no error)"=w1906, "Server in"=w1908) -> ("error out"=w1905:errorcluster, "connection"=w1904:bool, "Server out"=w1907:refnum<class "Acquisition.lvclass">)  [unwired: 7 in]
                  n761 = case shown="True" w1904 {
                    tunnel: w1905 -> [w1942 w1958]
                    tunnel: [w1942 w1957] -> w1928
                    tunnel: w1907 -> [w1943 w1948]
                    tunnel: [w1943 w1946] -> w1924
                    frame False {
                    }
                    frame True {
                      # "Envia comando TRIGGER_DONE  para o Acquisition"
                      n762 = call-dynamic "Read Channel.vi"("error in (no error)"=w1958, "Acquisition in"=w1948) -> ("error out"=w1953:errorcluster, "Channel.lvclass"=w1952:refnum<class "Channel.lvclass">, "Acquisition out"=w1947:refnum<class "Acquisition.lvclass">)  [unwired: 7 in]
                      n763 = call-dynamic "Read State Machine.vi"("error in (no error)"=w1953, "Device in"=w1952) -> ("error out"=w1954:errorcluster, "State Machine.lvclass"=w1956:refnum<class "State Machine.lvclass">, "Device out"=w1950:refnum<class "Channel.lvclass">)  [unwired: 7 in]
                      n764 = call "Next State.vi"("error in (no error)"=w1954, "New_State"=40, "State Machine in"=w1956) -> ("error out"=w1944:errorcluster, "State Machine out"=w1945:refnum<class "State Machine.lvclass">)  [unwired: 7 in]
                      n765 = call-dynamic "Write State Machine.vi"("error in (no error)"=w1944, "State Machine.lvclass"=w1945, "Device in"=w1950) -> ("error out"=w1949:errorcluster, "Device out"=w1951:refnum<class "Channel.lvclass">)  [unwired: 7 in]
                      n766 = call-dynamic "Write Channel.vi"("error in (no error)"=w1949, "Channel.lvclass"=w1951, "Acquisition in"=w1947) -> ("error out"=w1957:errorcluster, "Acquisition out"=w1946:refnum<class "Acquisition.lvclass">)  [unwired: 7 in]
                    }
                  }
                  n767 = call-dynamic "Write AcquisitionD.vi"("error in (no error)"=w1928, "Acquisition.lvclass"=w1924, "S4ACS_GUI in"=w1925) -> ("error out"=w1900:errorcluster, "S4ACS_GUI out"=w1901:refnum<class "S4GUI.lvclass">)  [unwired: 7 in]
                }
                frame Enabled {
                }
              }
            }
          }
          n768 = call-dynamic "Write Sync Box.lvclass.vi"("error in (no error)"=w1872, "Sync Box.lvclass"=w1873, "SPARC4_AC in"=w1858) -> ("error out"=w1869:errorcluster, "SPARC4_AC out"=w1868:refnum<class "S4GUI.lvclass">)  [unwired: 7 in]
          n769 = Bundle By Name(cluster=w1868, "Obs_state"=w1866) -> (w1865:refnum<class "S4GUI.lvclass">)
        }
        frame 309 {
          # "OV20230426: Se houver apenas 1\nposição da lâmina, desvia para 327\npara monitorar CyclesDone em vez\nde SequesDone. A partir de 327, o \nprocedimento é identico ao da \nfotometria."
          # "Espera terminar a execução do comando atual no SyncBox e nos \nAcquistion antes de ir ao proximo passo da Observação."
          n770 = call-dynamic "VerifWavePlate.vi"("error in (no error)"=w2020, "S4GUI in"=w2022) -> ("error out"=w2019:errorcluster, "One Position"=w2016:bool, "S4GUI out"=w2021:refnum<class "S4GUI.lvclass">)  [unwired: 7 in]
          n771 = Increment(x=w2024) -> (x+1=w2018:u32)
          n772 = call-dynamic "Read Sync Box.lvclass.vi"("error in (no error)"=w2019, "SPARC4_AC in"=w2021) -> ("error out"=w2040:errorcluster, "Sync Box.lvclass"=w2041:refnum<class "Sync Box.lvclass">, "SPARC4_AC out"=w2037:refnum<class "S4GUI.lvclass">)  [unwired: 7 in]
          n773 = Select(t=u32 327, s=w2016, f=w2018) -> (s? t:f=w2017:u32)
          n774 = call-dynamic "Read Trigger.lvclass.vi"("error in (no error)"=w2040, "Sync Box in"=w2041) -> ("error out"=w2035:errorcluster, "Trigger.lvclass"=w2034:refnum<class "Trigger.lvclass">, "Sync Box out"=w2039:refnum<class "Sync Box.lvclass">)  [unwired: 7 in]
          n775 = call-dynamic "Read State Machine.vi"("error in (no error)"=w2035, "Device in"=w2034) -> ("error out"=w2027:errorcluster, "State Machine.lvclass"=w2029:refnum<class "State Machine.lvclass">, "Device out"=w2032:refnum<class "Trigger.lvclass">)  [unwired: 7 in]
          n776 = call-dynamic "Read State.vi"("error in (no error)"=w2027, "State Machine in"=w2029) -> ("error out"=w2026:errorcluster, "State"=w2014:i32, "State Machine out"=w2028:refnum<class "State Machine.lvclass">)  [unwired: 7 in]
          n777 = call-dynamic "Write State Machine.vi"("error in (no error)"=w2026, "State Machine.lvclass"=w2028, "Device in"=w2032) -> ("error out"=w2031:errorcluster, "Device out"=w2033:refnum<class "Trigger.lvclass">)  [unwired: 7 in]
          n778 = call-dynamic "Write Trigger.lvclass.vi"("error in (no error)"=w2031, "Trigger.lvclass"=w2033, "Sync Box in"=w2039) -> ("error out"=w2036:errorcluster, "Sync Box out"=w2038:refnum<class "Sync Box.lvclass">)  [unwired: 7 in]
          n779 = call-dynamic "Write Sync Box.lvclass.vi"("error in (no error)"=w2036, "Sync Box.lvclass"=w2038, "SPARC4_AC in"=w2037) -> ("error out"=w2012:errorcluster, "SPARC4_AC out"=w2013:refnum<class "S4GUI.lvclass">)  [unwired: 7 in]
          n780 = Equal To 0?(x=w2014) -> (x = 0?=w2023:bool)
          n781 = Select(t=w2017, s=w2023, f=w2024) -> (s? t:f=w2025:u32)
          n782 = Bundle By Name(cluster=w2013, "Obs_state"=w2025) -> (w2030:refnum<class "S4GUI.lvclass">)
        }
        frame 310 {
          # "Exemplo:\nSET #CYCLES 3\nSET #SEQ 4\ntotal de sequencias: 3 x 4 = 12\n\nseq.        CYCLES_DONE           SEQS_DONE\n1a.                     0                                 0\n2a.                     0                                 1 \n3a.                     0                                 2 \n4a.                     0                                 3 \n\n5a.                     1                                 4->0 \n6a.                     1                                 1 \n7a.                     1                                 2 \n8a.                     1                                 3 \n\n9a.                     2                                 4->0 \n10a.                   2                                 1 \n11a.                   2                                 2 \n12a.                   2                                 3 \n\nfim                    3                                 4"
          # "Espera terminar a execução do comando atual \nantes de ir ao proximo passo da Observação."
          n783 = Unbundle By Name(w2062) -> ("sequesDone"=w2051:u32)
          n784 = call-dynamic "Read AcquisitionA.vi"("error in (no error)"=w2101, "S4ACS_GUI in"=w2062) -> ("error out"=w2081:errorcluster, "Acquisition.lvclass"=w2082:refnum<class "Acquisition.lvclass">, "S4ACS_GUI out"=w2103:refnum<class "S4GUI.lvclass">)  [unwired: 7 in]
          n785 = call "Read connection.vi"("error in (no error)"=w2081, "Server in"=w2082) -> ("error out"=w2080:errorcluster, "connection"=w2079:bool, "Server out"=w2078:refnum<class "Acquisition.lvclass">)  [unwired: 7 in]
          n786 = case shown="True" w2079 {
            tunnel: w2080 -> [w2174 w2190]
            tunnel: [w2175 w2188] -> w2104
            tunnel: [w2174 w2187] -> w2102
            tunnel: [u32 0 ("State") w2184] -> w2057
            tunnel: w2078 -> [w2175 w2183]
            tunnel: w2051 -> [_ w2182]
            tunnel: [TRUE w2181] -> w2061
            tunnel: [u32 0 ("CubesDone") w2180] -> w2046
            frame False {
            }
            frame True {
              # "SEQS_DONE = 0,1,2,...,n,0,1,..."
              n787 = call-dynamic "Read Channel.vi"("error in (no error)"=w2190, "Acquisition in"=w2183) -> ("error out"=w2177:errorcluster, "Channel.lvclass"=w2179:refnum<class "Channel.lvclass">, "Acquisition out"=w2189:refnum<class "Acquisition.lvclass">)  [unwired: 7 in]
              n788 = call-dynamic "Read CyclesDone.vi"("error in (no error)"=w2177, "Channel in"=w2179) -> ("error out"=w2176:errorcluster, "CyclesDone"=w2180:u32, "Channel out"=w2178:refnum<class "Channel.lvclass">)  [unwired: 7 in]
              n789 = call-dynamic "Read SequesDone.vi"("error in (no error)"=w2176, "Channel in"=w2178) -> ("error out"=w2185:errorcluster, "SequesDone"=w2184:u32, "Channel out"=w2186:refnum<class "Channel.lvclass">)  [unwired: 7 in]
              n790 = Not Equal?(x=w2184, y=w2182) -> (x != y?=w2181:bool)
              n791 = call-dynamic "Write Channel.vi"("error in (no error)"=w2185, "Channel.lvclass"=w2186, "Acquisition in"=w2189) -> ("error out"=w2187:errorcluster, "Acquisition out"=w2188:refnum<class "Acquisition.lvclass">)  [unwired: 7 in]
            }
          }
          n792 = call-dynamic "Write AcquisitionA.vi"("error in (no error)"=w2102, "Acquisition.lvclass"=w2104, "S4ACS_GUI in"=w2103) -> ("error out"=w2098:errorcluster, "S4ACS_GUI out"=w2097:refnum<class "S4GUI.lvclass">)  [unwired: 7 in]
          n793 = call "Read AcquisitionB.vi"("error in (no error)"=w2098, "S4ACS_GUI in"=w2097) -> ("error out"=w2073:errorcluster, "Acquisition.lvclass"=w2077:refnum<class "Acquisition.lvclass">, "S4ACS_GUI out"=w2099:refnum<class "S4GUI.lvclass">)  [unwired: 7 in]
          n794 = call "Read connection.vi"("error in (no error)"=w2073, "Server in"=w2077) -> ("error out"=w2074:errorcluster, "connection"=w2075:bool, "Server out"=w2076:refnum<class "Acquisition.lvclass">)  [unwired: 7 in]
          n795 = case shown="True" w2075 {
            tunnel: w2074 -> [w2154 w2170]
            tunnel: w2076 -> [w2155 w2169]
            tunnel: [u32 0 ("State") w2163] -> w2056
            tunnel: [w2154 w2168] -> w2096
            tunnel: [w2155 w2167] -> w2095
            tunnel: w2051 -> [_ w2162]
            tunnel: [TRUE w2161] -> w2052
            tunnel: [u32 0 ("CubesDone") w2156] -> w2045
            frame False {
            }
            frame True {
              n796 = call-dynamic "Read Channel.vi"("error in (no error)"=w2170, "Acquisition in"=w2169) -> ("error out"=w2158:errorcluster, "Channel.lvclass"=w2160:refnum<class "Channel.lvclass">, "Acquisition out"=w2164:refnum<class "Acquisition.lvclass">)  [unwired: 7 in]
              n797 = call-dynamic "Read CyclesDone.vi"("error in (no error)"=w2158, "Channel in"=w2160) -> ("error out"=w2157:errorcluster, "CyclesDone"=w2156:u32, "Channel out"=w2159:refnum<class "Channel.lvclass">)  [unwired: 7 in]
              n798 = call-dynamic "Read SequesDone.vi"("error in (no error)"=w2157, "Channel in"=w2159) -> ("error out"=w2166:errorcluster, "SequesDone"=w2163:u32, "Channel out"=w2165:refnum<class "Channel.lvclass">)  [unwired: 7 in]
              n799 = Not Equal?(x=w2163, y=w2162) -> (x != y?=w2161:bool)
              n800 = call-dynamic "Write Channel.vi"("error in (no error)"=w2166, "Channel.lvclass"=w2165, "Acquisition in"=w2164) -> ("error out"=w2168:errorcluster, "Acquisition out"=w2167:refnum<class "Acquisition.lvclass">)  [unwired: 7 in]
            }
          }
          n801 = Max & Min(x=w2046, y=w2045) -> (max(x,y)=w2048:u32)  [unwired: 1 out]
          n802 = Max & Min(x=w2057, y=w2056) -> (max(x,y)=w2059:u32)  [unwired: 1 out]
          n803 = call "Write AcquisitionB.vi"("error in (no error)"=w2096, "Acquisition.lvclass"=w2095, "S4ACS_GUI in"=w2099) -> ("error out"=w2088:errorcluster, "S4ACS_GUI out"=w2087:refnum<class "S4GUI.lvclass">)  [unwired: 7 in]
          n804 = call-dynamic "Read AcquisitionC.vi"("error in (no error)"=w2088, "S4ACS_GUI in"=w2087) -> ("error out"=w2069:errorcluster, "Acquisition.lvclass"=w2072:refnum<class "Acquisition.lvclass">, "S4ACS_GUI out"=w2090:refnum<class "S4GUI.lvclass">)  [unwired: 7 in]
          n805 = call "Read connection.vi"("error in (no error)"=w2069, "Server in"=w2072) -> ("error out"=w2068:errorcluster, "connection"=w2070:bool, "Server out"=w2071:refnum<class "Acquisition.lvclass">)  [unwired: 7 in]
          n806 = case shown="True" w2070 {
            tunnel: [w2134 w2150] -> w2091
            tunnel: [w2135 w2149] -> w2089
            tunnel: w2068 -> [w2134 w2146]
            tunnel: w2071 -> [w2135 w2147]
            tunnel: [u32 0 ("State") w2145] -> w2055
            tunnel: w2051 -> [_ w2144]
            tunnel: [TRUE w2143] -> w2050
            tunnel: [u32 0 ("CubesDone") w2136] -> w2044
            frame False {
            }
            frame True {
              n807 = call-dynamic "Read Channel.vi"("error in (no error)"=w2146, "Acquisition in"=w2147) -> ("error out"=w2138:errorcluster, "Channel.lvclass"=w2140:refnum<class "Channel.lvclass">, "Acquisition out"=w2148:refnum<class "Acquisition.lvclass">)  [unwired: 7 in]
              n808 = call-dynamic "Read CyclesDone.vi"("error in (no error)"=w2138, "Channel in"=w2140) -> ("error out"=w2137:errorcluster, "CyclesDone"=w2136:u32, "Channel out"=w2139:refnum<class "Channel.lvclass">)  [unwired: 7 in]
              n809 = call-dynamic "Read SequesDone.vi"("error in (no error)"=w2137, "Channel in"=w2139) -> ("error out"=w2142:errorcluster, "SequesDone"=w2145:u32, "Channel out"=w2141:refnum<class "Channel.lvclass">)  [unwired: 7 in]
              n810 = Not Equal?(x=w2145, y=w2144) -> (x != y?=w2143:bool)
              n811 = call-dynamic "Write Channel.vi"("error in (no error)"=w2142, "Channel.lvclass"=w2141, "Acquisition in"=w2148) -> ("error out"=w2150:errorcluster, "Acquisition out"=w2149:refnum<class "Acquisition.lvclass">)  [unwired: 7 in]
            }
          }
          n812 = call-dynamic "Write AcquisitionC.vi"("error in (no error)"=w2091, "Acquisition.lvclass"=w2089, "S4ACS_GUI in"=w2090) -> ("error out"=w2085:errorcluster, "S4ACS_GUI out"=w2086:refnum<class "S4GUI.lvclass">)  [unwired: 7 in]
          n813 = call-dynamic "Read AcquisitionD.vi"("error in (no error)"=w2085, "S4ACS_GUI in"=w2086) -> ("error out"=w2064:errorcluster, "Acquisition.lvclass"=w2067:refnum<class "Acquisition.lvclass">, "S4ACS_GUI out"=w2092:refnum<class "S4GUI.lvclass">)  [unwired: 7 in]
          n814 = call "Read connection.vi"("error in (no error)"=w2064, "Server in"=w2067) -> ("error out"=w2063:errorcluster, "connection"=w2065:bool, "Server out"=w2066:refnum<class "Acquisition.lvclass">)  [unwired: 7 in]
          n815 = case shown="True" w2065 {
            tunnel: [w2115 w2130] -> w2094
            tunnel: [w2114 w2129] -> w2093
            tunnel: w2066 -> [w2115 w2128]
            tunnel: w2063 -> [w2114 w2127]
            tunnel: [u32 0 ("State") w2125] -> w2054
            tunnel: w2051 -> [_ w2124]
            tunnel: [TRUE w2123] -> w2049
            tunnel: [u32 0 ("CubesDone") w2116] -> w2043
            frame False {
            }
            frame True {
              n816 = call-dynamic "Read Channel.vi"("error in (no error)"=w2127, "Acquisition in"=w2128) -> ("error out"=w2118:errorcluster, "Channel.lvclass"=w2120:refnum<class "Channel.lvclass">, "Acquisition out"=w2126:refnum<class "Acquisition.lvclass">)  [unwired: 7 in]
              n817 = call-dynamic "Read CyclesDone.vi"("error in (no error)"=w2118, "Channel in"=w2120) -> ("error out"=w2117:errorcluster, "CyclesDone"=w2116:u32, "Channel out"=w2119:refnum<class "Channel.lvclass">)  [unwired: 7 in]
              n818 = call-dynamic "Read SequesDone.vi"("error in (no error)"=w2117, "Channel in"=w2119) -> ("error out"=w2122:errorcluster, "SequesDone"=w2125:u32, "Channel out"=w2121:refnum<class "Channel.lvclass">)  [unwired: 7 in]
              n819 = Not Equal?(x=w2125, y=w2124) -> (x != y?=w2123:bool)
              n820 = call-dynamic "Write Channel.vi"("error in (no error)"=w2122, "Channel.lvclass"=w2121, "Acquisition in"=w2126) -> ("error out"=w2129:errorcluster, "Acquisition out"=w2130:refnum<class "Acquisition.lvclass">)  [unwired: 7 in]
            }
          }
          n821 = Max & Min(x=w2044, y=w2043) -> (max(x,y)=w2047:u32)  [unwired: 1 out]
          n822 = Max & Min(x=w2055, y=w2054) -> (max(x,y)=w2058:u32)  [unwired: 1 out]
          n823 = Compound Arithmetic op=AND(w2061, w2052, w2050, w2049) -> (w2060:bool)
          n824 = Max & Min(x=w2059, y=w2058) -> (max(x,y)=w2053:u32)  [unwired: 1 out]
          n825 = Max & Min(x=w2048, y=w2047) -> (max(x,y)=w2042:u32)  [unwired: 1 out]
          n826 = call-dynamic "Write AcquisitionD.vi"("error in (no error)"=w2093, "Acquisition.lvclass"=w2094, "S4ACS_GUI in"=w2092) -> ("error out"=w2083:errorcluster, "S4ACS_GUI out"=w2084:refnum<class "S4GUI.lvclass">)  [unwired: 7 in]
          n827 = case shown="True" w2060 {
            tunnel: w2084 -> [w2105 w2110]
            tunnel: [w2105 w2109] -> w2100
            tunnel: w2053 -> [_ w2108]
            tunnel: w2042 -> [_ w2106]
            frame False {
            }
            frame True {
              n828 = Bundle By Name(cluster=w2110, "Obs_state"=u32 301, "sequesDone"=w2108, "cyclesDone"=w2106) -> (w2109:refnum<class "S4GUI.lvclass">)
            }
          }
        }
        frame 311 {
          n829 = disable-structure shown="Enabled" {
            disable-tunnel: w2194 -> [w2208 w2221]
            disable-tunnel: w2193 -> [w2207 w2219]
            disable-tunnel: [w2206 w2219] -> w2192
            disable-tunnel: [w2204 w2220] -> w2191
            frame Disabled {
              n830 = call-dynamic "Read ciclos.vi"("error in (no error)"=w2207, "S4ACS_GUI in"=w2208) -> ("error out"=w2196:errorcluster, "ciclos"=w2201:u32, "S4ACS_GUI out"=w2209:refnum<class "S4GUI.lvclass">)  [unwired: 7 in]
              n831 = Decrement(x=w2201) -> (x-1=w2195:u32)
              n832 = Greater Than 0?(x=w2195) -> (x > 0?=w2202:bool)
              n833 = case shown="False" w2202 {
                selector: w2202 -> [w2211 w2213]
                tunnel: w2195 -> [_ w2212]
                tunnel: [w2211 w2213] -> w2200
                tunnel: [u32 0 w2212] -> w2197
                frame False {
                }
                frame True {
                }
              }
              n834 = Select(t=u32 323, s=w2200, f=u32 0) -> (s? t:f=w2203:u32)
              n835 = call-dynamic "Write ciclos.vi"("error in (no error)"=w2196, "ciclos"=w2197, "S4ACS_GUI in"=w2209) -> ("error out"=w2206:errorcluster, "S4ACS_GUI out"=w2205:refnum<class "S4GUI.lvclass">)  [unwired: 7 in]
              n836 = Bundle By Name(cluster=w2205, "Obs_state"=w2203) -> (w2204:refnum<class "S4GUI.lvclass">)
            }
            frame Enabled {
              n837 = Unbundle By Name(w2221) -> ("TotalCiclos"=w2223:u32, "cyclesDone"=w2222:u32)
              n838 = Subtract(x=w2223, y=w2222) -> (x-y=w2218:u32)
              n839 = Greater Than 0?(x=w2218) -> (x > 0?=w2217:bool)
              n840 = Select(t=u32 301, s=w2217, f=u32 0) -> (s? t:f=w2216:u32)
              n841 = Bundle By Name(cluster=w2221, "Obs_state"=w2216) -> (w2220:refnum<class "S4GUI.lvclass">)
            }
          }
        }
        frame 312 {
          # "Espera terminar a execução do comando atual \nantes de ir ao proximo passo da Observação."
          n842 = call-dynamic "Read AcquisitionA.vi"("error in (no error)"=w2271, "S4ACS_GUI in"=w2272) -> ("error out"=w2240:errorcluster, "Acquisition.lvclass"=w2241:refnum<class "Acquisition.lvclass">, "S4ACS_GUI out"=w2274:refnum<class "S4GUI.lvclass">)  [unwired: 7 in]
          n843 = call "Read connection.vi"("error in (no error)"=w2240, "Server in"=w2241) -> ("error out"=w2242:errorcluster, "connection"=w2244:bool, "Server out"=w2243:refnum<class "Acquisition.lvclass">)  [unwired: 7 in]
          n844 = case shown="True" w2244 {
            tunnel: [w2332 w2346] -> w2275
            tunnel: [w2331 w2345] -> w2273
            tunnel: [0 ("State") w2335] -> w2265
            tunnel: w2243 -> [w2332 w2334]
            tunnel: w2242 -> [w2331 w2333]
            frame False {
            }
            frame True {
              n845 = call-dynamic "Read Channel.vi"("error in (no error)"=w2333, "Acquisition in"=w2334) -> ("error out"=w2344:errorcluster, "Channel.lvclass"=w2343:refnum<class "Channel.lvclass">, "Acquisition out"=w2347:refnum<class "Acquisition.lvclass">)  [unwired: 7 in]
              n846 = call-dynamic "Read State Machine.vi"("error in (no error)"=w2344, "Device in"=w2343) -> ("error out"=w2337:errorcluster, "State Machine.lvclass"=w2339:refnum<class "State Machine.lvclass">, "Device out"=w2341:refnum<class "Channel.lvclass">)  [unwired: 7 in]
              n847 = call-dynamic "Read State.vi"("error in (no error)"=w2337, "State Machine in"=w2339) -> ("error out"=w2336:errorcluster, "State"=w2335:i32, "State Machine out"=w2338:refnum<class "State Machine.lvclass">)  [unwired: 7 in]
              n848 = call-dynamic "Write State Machine.vi"("error in (no error)"=w2336, "State Machine.lvclass"=w2338, "Device in"=w2341) -> ("error out"=w2340:errorcluster, "Device out"=w2342:refnum<class "Channel.lvclass">)  [unwired: 7 in]
              n849 = call-dynamic "Write Channel.vi"("error in (no error)"=w2340, "Channel.lvclass"=w2342, "Acquisition in"=w2347) -> ("error out"=w2345:errorcluster, "Acquisition out"=w2346:refnum<class "Acquisition.lvclass">)  [unwired: 7 in]
            }
          }
          n850 = call-dynamic "Write AcquisitionA.vi"("error in (no error)"=w2273, "Acquisition.lvclass"=w2275, "S4ACS_GUI in"=w2274) -> ("error out"=w2266:errorcluster, "S4ACS_GUI out"=w2267:refnum<class "S4GUI.lvclass">)  [unwired: 7 in]
          n851 = call "Read AcquisitionB.vi"("error in (no error)"=w2266, "S4ACS_GUI in"=w2267) -> ("error out"=w2237:errorcluster, "Acquisition.lvclass"=w2239:refnum<class "Acquisition.lvclass">, "S4ACS_GUI out"=w2260:refnum<class "S4GUI.lvclass">)  [unwired: 7 in]
          n852 = call "Read connection.vi"("error in (no error)"=w2237, "Server in"=w2239) -> ("error out"=w2236:errorcluster, "connection"=w2235:bool, "Server out"=w2238:refnum<class "Acquisition.lvclass">)  [unwired: 7 in]
          n853 = case shown="True" w2235 {
            tunnel: w2238 -> [w2314 w2329]
            tunnel: w2236 -> [w2313 w2328]
            tunnel: [w2314 w2326] -> w2261
            tunnel: [w2313 w2325] -> w2259
            tunnel: [0 ("State") w2315] -> w2258
            frame False {
            }
            frame True {
              n854 = call-dynamic "Read Channel.vi"("error in (no error)"=w2328, "Acquisition in"=w2329) -> ("error out"=w2324:errorcluster, "Channel.lvclass"=w2323:refnum<class "Channel.lvclass">, "Acquisition out"=w2327:refnum<class "Acquisition.lvclass">)  [unwired: 7 in]
              n855 = call-dynamic "Read State Machine.vi"("error in (no error)"=w2324, "Device in"=w2323) -> ("error out"=w2317:errorcluster, "State Machine.lvclass"=w2319:refnum<class "State Machine.lvclass">, "Device out"=w2321:refnum<class "Channel.lvclass">)  [unwired: 7 in]
              n856 = call-dynamic "Read State.vi"("error in (no error)"=w2317, "State Machine in"=w2319) -> ("error out"=w2316:errorcluster, "State"=w2315:i32, "State Machine out"=w2318:refnum<class "State Machine.lvclass">)  [unwired: 7 in]
              n857 = call-dynamic "Write State Machine.vi"("error in (no error)"=w2316, "State Machine.lvclass"=w2318, "Device in"=w2321) -> ("error out"=w2320:errorcluster, "Device out"=w2322:refnum<class "Channel.lvclass">)  [unwired: 7 in]
              n858 = call-dynamic "Write Channel.vi"("error in (no error)"=w2320, "Channel.lvclass"=w2322, "Acquisition in"=w2327) -> ("error out"=w2325:errorcluster, "Acquisition out"=w2326:refnum<class "Acquisition.lvclass">)  [unwired: 7 in]
            }
          }
          n859 = call "Write AcquisitionB.vi"("error in (no error)"=w2259, "Acquisition.lvclass"=w2261, "S4ACS_GUI in"=w2260) -> ("error out"=w2254:errorcluster, "S4ACS_GUI out"=w2253:refnum<class "S4GUI.lvclass">)  [unwired: 7 in]
          n860 = call-dynamic "Read AcquisitionC.vi"("error in (no error)"=w2254, "S4ACS_GUI in"=w2253) -> ("error out"=w2232:errorcluster, "Acquisition.lvclass"=w2234:refnum<class "Acquisition.lvclass">, "S4ACS_GUI out"=w2256:refnum<class "S4GUI.lvclass">)  [unwired: 7 in]
          n861 = call "Read connection.vi"("error in (no error)"=w2232, "Server in"=w2234) -> ("error out"=w2231:errorcluster, "connection"=w2230:bool, "Server out"=w2233:refnum<class "Acquisition.lvclass">)  [unwired: 7 in]
          n862 = case shown="True" w2230 {
            tunnel: [w2294 w2304] -> w2257
            tunnel: [w2295 w2303] -> w2255
            tunnel: [0 ("State") w2299] -> w2252
            tunnel: w2233 -> [w2295 w2298]
            tunnel: w2231 -> [w2294 w2297]
            frame False {
            }
            frame True {
              n863 = call-dynamic "Read Channel.vi"("error in (no error)"=w2297, "Acquisition in"=w2298) -> ("error out"=w2305:errorcluster, "Channel.lvclass"=w2306:refnum<class "Channel.lvclass">, "Acquisition out"=w2302:refnum<class "Acquisition.lvclass">)  [unwired: 7 in]
              n864 = call-dynamic "Read State Machine.vi"("error in (no error)"=w2305, "Device in"=w2306) -> ("error out"=w2300:errorcluster, "State Machine.lvclass"=w2310:refnum<class "State Machine.lvclass">, "Device out"=w2308:refnum<class "Channel.lvclass">)  [unwired: 7 in]
              n865 = call-dynamic "Read State.vi"("error in (no error)"=w2300, "State Machine in"=w2310) -> ("error out"=w2301:errorcluster, "State"=w2299:i32, "State Machine out"=w2311:refnum<class "State Machine.lvclass">)  [unwired: 7 in]
              n866 = call-dynamic "Write State Machine.vi"("error in (no error)"=w2301, "State Machine.lvclass"=w2311, "Device in"=w2308) -> ("error out"=w2309:errorcluster, "Device out"=w2307:refnum<class "Channel.lvclass">)  [unwired: 7 in]
              n867 = call-dynamic "Write Channel.vi"("error in (no error)"=w2309, "Channel.lvclass"=w2307, "Acquisition in"=w2302) -> ("error out"=w2304:errorcluster, "Acquisition out"=w2303:refnum<class "Acquisition.lvclass">)  [unwired: 7 in]
            }
          }
          n868 = call-dynamic "Write AcquisitionC.vi"("error in (no error)"=w2257, "Acquisition.lvclass"=w2255, "S4ACS_GUI in"=w2256) -> ("error out"=w2229:errorcluster, "S4ACS_GUI out"=w2248:refnum<class "S4GUI.lvclass">)  [unwired: 7 in]
          n869 = call-dynamic "Read AcquisitionD.vi"("error in (no error)"=w2229, "S4ACS_GUI in"=w2248) -> ("error out"=w2225:errorcluster, "Acquisition.lvclass"=w2228:refnum<class "Acquisition.lvclass">, "S4ACS_GUI out"=w2250:refnum<class "S4GUI.lvclass">)  [unwired: 7 in]
          n870 = call "Read connection.vi"("error in (no error)"=w2225, "Server in"=w2228) -> ("error out"=w2226:errorcluster, "connection"=w2224:bool, "Server out"=w2227:refnum<class "Acquisition.lvclass">)  [unwired: 7 in]
          n871 = case shown="True" w2224 {
            tunnel: [w2278 w2292] -> w2251
            tunnel: [w2277 w2291] -> w2249
            tunnel: [0 ("State") w2281] -> w2247
            tunnel: w2227 -> [w2278 w2280]
            tunnel: w2226 -> [w2277 w2279]
            frame False {
            }
            frame True {
              n872 = call-dynamic "Read Channel.vi"("error in (no error)"=w2279, "Acquisition in"=w2280) -> ("error out"=w2290:errorcluster, "Channel.lvclass"=w2289:refnum<class "Channel.lvclass">, "Acquisition out"=w2293:refnum<class "Acquisition.lvclass">)  [unwired: 7 in]
              n873 = call-dynamic "Read State Machine.vi"("error in (no error)"=w2290, "Device in"=w2289) -> ("error out"=w2283:errorcluster, "State Machine.lvclass"=w2285:refnum<class "State Machine.lvclass">, "Device out"=w2287:refnum<class "Channel.lvclass">)  [unwired: 7 in]
              n874 = call-dynamic "Read State.vi"("error in (no error)"=w2283, "State Machine in"=w2285) -> ("error out"=w2282:errorcluster, "State"=w2281:i32, "State Machine out"=w2284:refnum<class "State Machine.lvclass">)  [unwired: 7 in]
              n875 = call-dynamic "Write State Machine.vi"("error in (no error)"=w2282, "State Machine.lvclass"=w2284, "Device in"=w2287) -> ("error out"=w2286:errorcluster, "Device out"=w2288:refnum<class "Channel.lvclass">)  [unwired: 7 in]
              n876 = call-dynamic "Write Channel.vi"("error in (no error)"=w2286, "Channel.lvclass"=w2288, "Acquisition in"=w2293) -> ("error out"=w2291:errorcluster, "Acquisition out"=w2292:refnum<class "Acquisition.lvclass">)  [unwired: 7 in]
            }
          }
          n877 = call-dynamic "Write AcquisitionD.vi"("error in (no error)"=w2249, "Acquisition.lvclass"=w2251, "S4ACS_GUI in"=w2250) -> ("error out"=w2245:errorcluster, "S4ACS_GUI out"=w2246:refnum<class "S4GUI.lvclass">)  [unwired: 7 in]
          n878 = Compound Arithmetic op=ADD(w2265, w2258, w2252, w2247) -> (w2264:i32)
          n879 = Equal To 0?(x=w2264) -> (x = 0?=w2269:bool)
          n880 = Select(t=u32 301, s=w2269, f=w2263) -> (s? t:f=w2268:u32)
          n881 = Bundle By Name(cluster=w2246, "Obs_state"=w2268) -> (w2270:refnum<class "S4GUI.lvclass">)
        }
        frame 313 {
          n882 = call-dynamic "Read ciclos.vi"("error in (no error)"=w2360, "S4ACS_GUI in"=w2361) -> ("error out"=w2349:errorcluster, "ciclos"=w2354:u32, "S4ACS_GUI out"=w2362:refnum<class "S4GUI.lvclass">)  [unwired: 7 in]
          n883 = Decrement(x=w2354) -> (x-1=w2348:u32)
          n884 = Greater Than 0?(x=w2348) -> (x > 0?=w2355:bool)
          n885 = case shown="False" w2355 {
            selector: w2355 -> [w2364 w2366]
            tunnel: w2348 -> [_ w2365]
            tunnel: [w2364 w2366] -> w2353
            tunnel: [u32 0 w2365] -> w2350
            frame False {
            }
            frame True {
            }
          }
          n886 = Select(t=u32 301, s=w2353, f=u32 0) -> (s? t:f=w2356:u32)
          n887 = call-dynamic "Write ciclos.vi"("error in (no error)"=w2349, "ciclos"=w2350, "S4ACS_GUI in"=w2362) -> ("error out"=w2359:errorcluster, "S4ACS_GUI out"=w2358:refnum<class "S4GUI.lvclass">)  [unwired: 7 in]
          n888 = Bundle By Name(cluster=w2358, "Obs_state"=w2356) -> (w2357:refnum<class "S4GUI.lvclass">)
        }
        frame 323 {
          n889 = call-dynamic "Read AcquisitionA.vi"("error in (no error)"=w2369, "S4ACS_GUI in"=w2370) -> ("error out"=w2387:errorcluster, "Acquisition.lvclass"=w2390:refnum<class "Acquisition.lvclass">, "S4ACS_GUI out"=w2407:refnum<class "S4GUI.lvclass">)  [unwired: 7 in]
          n890 = call "Read connection.vi"("error in (no error)"=w2387, "Server in"=w2390) -> ("error out"=w2386:errorcluster, "connection"=w2388:bool, "Server out"=w2389:refnum<class "Acquisition.lvclass">)  [unwired: 7 in]
          n891 = case shown="True" w2388 {
            tunnel: w2389 -> [w2464 w2479]
            tunnel: w2386 -> [w2463 w2478]
            tunnel: [w2464 w2476] -> w2408
            tunnel: [w2463 w2475] -> w2406
            frame False {
            }
            frame True {
              n892 = call-dynamic "Read Channel.vi"("error in (no error)"=w2478, "Acquisition in"=w2479) -> ("error out"=w2471:errorcluster, "Channel.lvclass"=w2470:refnum<class "Channel.lvclass">, "Acquisition out"=w2477:refnum<class "Acquisition.lvclass">)  [unwired: 7 in]
              n893 = call-dynamic "Read State Machine.vi"("error in (no error)"=w2471, "Device in"=w2470) -> ("error out"=w2472:errorcluster, "State Machine.lvclass"=w2474:refnum<class "State Machine.lvclass">, "Device out"=w2468:refnum<class "Channel.lvclass">)  [unwired: 7 in]
              n894 = call "Next State.vi"("error in (no error)"=w2472, "New_State"=50, "State Machine in"=w2474) -> ("error out"=w2465:errorcluster, "State Machine out"=w2466:refnum<class "State Machine.lvclass">)  [unwired: 7 in]
              n895 = call-dynamic "Write State Machine.vi"("error in (no error)"=w2465, "State Machine.lvclass"=w2466, "Device in"=w2468) -> ("error out"=w2467:errorcluster, "Device out"=w2469:refnum<class "Channel.lvclass">)  [unwired: 7 in]
              n896 = call-dynamic "Write Channel.vi"("error in (no error)"=w2467, "Channel.lvclass"=w2469, "Acquisition in"=w2477) -> ("error out"=w2475:errorcluster, "Acquisition out"=w2476:refnum<class "Acquisition.lvclass">)  [unwired: 7 in]
            }
          }
          n897 = call-dynamic "Write AcquisitionA.vi"("error in (no error)"=w2406, "Acquisition.lvclass"=w2408, "S4ACS_GUI in"=w2407) -> ("error out"=w2404:errorcluster, "S4ACS_GUI out"=w2405:refnum<class "S4GUI.lvclass">)  [unwired: 7 in]
          n898 = call "Read AcquisitionB.vi"("error in (no error)"=w2404, "S4ACS_GUI in"=w2405) -> ("error out"=w2383:errorcluster, "Acquisition.lvclass"=w2385:refnum<class "Acquisition.lvclass">, "S4ACS_GUI out"=w2402:refnum<class "S4GUI.lvclass">)  [unwired: 7 in]
          n899 = call "Read connection.vi"("error in (no error)"=w2383, "Server in"=w2385) -> ("error out"=w2382:errorcluster, "connection"=w2381:bool, "Server out"=w2384:refnum<class "Acquisition.lvclass">)  [unwired: 7 in]
          n900 = case shown="True" w2381 {
            tunnel: w2384 -> [w2447 w2462]
            tunnel: w2382 -> [w2446 w2461]
            tunnel: [w2447 w2459] -> w2403
            tunnel: [w2446 w2458] -> w2401
            frame False {
            }
            frame True {
              n901 = call-dynamic "Read Channel.vi"("error in (no error)"=w2461, "Acquisition in"=w2462) -> ("error out"=w2454:errorcluster, "Channel.lvclass"=w2453:refnum<class "Channel.lvclass">, "Acquisition out"=w2460:refnum<class "Acquisition.lvclass">)  [unwired: 7 in]
              n902 = call-dynamic "Read State Machine.vi"("error in (no error)"=w2454, "Device in"=w2453) -> ("error out"=w2455:errorcluster, "State Machine.lvclass"=w2457:refnum<class "State Machine.lvclass">, "Device out"=w2451:refnum<class "Channel.lvclass">)  [unwired: 7 in]
              n903 = call "Next State.vi"("error in (no error)"=w2455, "New_State"=50, "State Machine in"=w2457) -> ("error out"=w2448:errorcluster, "State Machine out"=w2449:refnum<class "State Machine.lvclass">)  [unwired: 7 in]
              n904 = call-dynamic "Write State Machine.vi"("error in (no error)"=w2448, "State Machine.lvclass"=w2449, "Device in"=w2451) -> ("error out"=w2450:errorcluster, "Device out"=w2452:refnum<class "Channel.lvclass">)  [unwired: 7 in]
              n905 = call-dynamic "Write Channel.vi"("error in (no error)"=w2450, "Channel.lvclass"=w2452, "Acquisition in"=w2460) -> ("error out"=w2458:errorcluster, "Acquisition out"=w2459:refnum<class "Acquisition.lvclass">)  [unwired: 7 in]
            }
          }
          n906 = call "Write AcquisitionB.vi"("error in (no error)"=w2401, "Acquisition.lvclass"=w2403, "S4ACS_GUI in"=w2402) -> ("error out"=w2397:errorcluster, "S4ACS_GUI out"=w2396:refnum<class "S4GUI.lvclass">)  [unwired: 7 in]
          n907 = call-dynamic "Read AcquisitionC.vi"("error in (no error)"=w2397, "S4ACS_GUI in"=w2396) -> ("error out"=w2378:errorcluster, "Acquisition.lvclass"=w2380:refnum<class "Acquisition.lvclass">, "S4ACS_GUI out"=w2399:refnum<class "S4GUI.lvclass">)  [unwired: 7 in]
          n908 = call "Read connection.vi"("error in (no error)"=w2378, "Server in"=w2380) -> ("error out"=w2377:errorcluster, "connection"=w2376:bool, "Server out"=w2379:refnum<class "Acquisition.lvclass">)  [unwired: 7 in]
          n909 = case shown="True" w2376 {
            tunnel: [w2429 w2437] -> w2400
            tunnel: [w2430 w2436] -> w2398
            tunnel: w2379 -> [w2430 w2434]
            tunnel: w2377 -> [w2429 w2433]
            frame False {
            }
            frame True {
              n910 = call-dynamic "Read Channel.vi"("error in (no error)"=w2433, "Acquisition in"=w2434) -> ("error out"=w2441:errorcluster, "Channel.lvclass"=w2442:refnum<class "Channel.lvclass">, "Acquisition out"=w2435:refnum<class "Acquisition.lvclass">)  [unwired: 7 in]
              n911 = call-dynamic "Read State Machine.vi"("error in (no error)"=w2441, "Device in"=w2442) -> ("error out"=w2440:errorcluster, "State Machine.lvclass"=w2438:refnum<class "State Machine.lvclass">, "Device out"=w2444:refnum<class "Channel.lvclass">)  [unwired: 7 in]
              n912 = call "Next State.vi"("error in (no error)"=w2440, "New_State"=50, "State Machine in"=w2438) -> ("error out"=w2431:errorcluster, "State Machine out"=w2432:refnum<class "State Machine.lvclass">)  [unwired: 7 in]
              n913 = call-dynamic "Write State Machine.vi"("error in (no error)"=w2431, "State Machine.lvclass"=w2432, "Device in"=w2444) -> ("error out"=w2445:errorcluster, "Device out"=w2443:refnum<class "Channel.lvclass">)  [unwired: 7 in]
              n914 = call-dynamic "Write Channel.vi"("error in (no error)"=w2445, "Channel.lvclass"=w2443, "Acquisition in"=w2435) -> ("error out"=w2437:errorcluster, "Acquisition out"=w2436:refnum<class "Acquisition.lvclass">)  [unwired: 7 in]
            }
          }
          n915 = call-dynamic "Write AcquisitionC.vi"("error in (no error)"=w2400, "Acquisition.lvclass"=w2398, "S4ACS_GUI in"=w2399) -> ("error out"=w2394:errorcluster, "S4ACS_GUI out"=w2393:refnum<class "S4GUI.lvclass">)  [unwired: 7 in]
          n916 = call-dynamic "Read AcquisitionD.vi"("error in (no error)"=w2394, "S4ACS_GUI in"=w2393) -> ("error out"=w2373:errorcluster, "Acquisition.lvclass"=w2375:refnum<class "Acquisition.lvclass">, "S4ACS_GUI out"=w2392:refnum<class "S4GUI.lvclass">)  [unwired: 7 in]
          n917 = call "Read connection.vi"("error in (no error)"=w2373, "Server in"=w2375) -> ("error out"=w2372:errorcluster, "connection"=w2371:bool, "Server out"=w2374:refnum<class "Acquisition.lvclass">)  [unwired: 7 in]
          n918 = case shown="True" w2371 {
            tunnel: w2372 -> [w2412 w2428]
            tunnel: [w2412 w2427] -> w2395
            tunnel: w2374 -> [w2413 w2418]
            tunnel: [w2413 w2416] -> w2391
            frame False {
            }
            frame True {
              n919 = call-dynamic "Read Channel.vi"("error in (no error)"=w2428, "Acquisition in"=w2418) -> ("error out"=w2423:errorcluster, "Channel.lvclass"=w2422:refnum<class "Channel.lvclass">, "Acquisition out"=w2417:refnum<class "Acquisition.lvclass">)  [unwired: 7 in]
              n920 = call-dynamic "Read State Machine.vi"("error in (no error)"=w2423, "Device in"=w2422) -> ("error out"=w2424:errorcluster, "State Machine.lvclass"=w2426:refnum<class "State Machine.lvclass">, "Device out"=w2420:refnum<class "Channel.lvclass">)  [unwired: 7 in]
              n921 = call "Next State.vi"("error in (no error)"=w2424, "New_State"=50, "State Machine in"=w2426) -> ("error out"=w2414:errorcluster, "State Machine out"=w2415:refnum<class "State Machine.lvclass">)  [unwired: 7 in]
              n922 = call-dynamic "Write State Machine.vi"("error in (no error)"=w2414, "State Machine.lvclass"=w2415, "Device in"=w2420) -> ("error out"=w2419:errorcluster, "Device out"=w2421:refnum<class "Channel.lvclass">)  [unwired: 7 in]
              n923 = call-dynamic "Write Channel.vi"("error in (no error)"=w2419, "Channel.lvclass"=w2421, "Acquisition in"=w2417) -> ("error out"=w2427:errorcluster, "Acquisition out"=w2416:refnum<class "Acquisition.lvclass">)  [unwired: 7 in]
            }
          }
          n924 = call-dynamic "Write AcquisitionD.vi"("error in (no error)"=w2395, "Acquisition.lvclass"=w2391, "S4ACS_GUI in"=w2392) -> ("error out"=w2367:errorcluster, "S4ACS_GUI out"=w2368:refnum<class "S4GUI.lvclass">)  [unwired: 7 in]
          n925 = Increment(x=w2411) -> (x+1=w2410:u32)
          n926 = Bundle By Name(cluster=w2368, "Obs_state"=w2410) -> (w2409:refnum<class "S4GUI.lvclass">)
        }
        frame 324 {
          # "Espera terminar a execução do comando atual \nantes de ir ao proximo passo da Observação."
          n927 = call-dynamic "Read AcquisitionA.vi"("error in (no error)"=w2526, "S4ACS_GUI in"=w2527) -> ("error out"=w2503:errorcluster, "Acquisition.lvclass"=w2504:refnum<class "Acquisition.lvclass">, "S4ACS_GUI out"=w2529:refnum<class "S4GUI.lvclass">)  [unwired: 7 in]
          n928 = call "Read connection.vi"("error in (no error)"=w2503, "Server in"=w2504) -> ("error out"=w2502:errorcluster, "connection"=w2501:bool, "Server out"=w2500:refnum<class "Acquisition.lvclass">)  [unwired: 7 in]
          n929 = case shown="True" w2501 {
            tunnel: w2502 -> [w2592 w2610]
            tunnel: [w2593 w2608] -> w2530
            tunnel: [w2592 w2607] -> w2528
            tunnel: [TRUE w2594] -> w2482
            tunnel: w2500 -> [w2593 w2597]
            frame False {
            }
            frame True {
              n930 = call-dynamic "Read Channel.vi"("error in (no error)"=w2610, "Acquisition in"=w2597) -> ("error out"=w2606:errorcluster, "Channel.lvclass"=w2605:refnum<class "Channel.lvclass">, "Acquisition out"=w2609:refnum<class "Acquisition.lvclass">)  [unwired: 7 in]
              n931 = call-dynamic "Read State Machine.vi"("error in (no error)"=w2606, "Device in"=w2605) -> ("error out"=w2599:errorcluster, "State Machine.lvclass"=w2601:refnum<class "State Machine.lvclass">, "Device out"=w2603:refnum<class "Channel.lvclass">)  [unwired: 7 in]
              n932 = call-dynamic "Read State.vi"("error in (no error)"=w2599, "State Machine in"=w2601) -> ("error out"=w2598:errorcluster, "State"=w2595:i32, "State Machine out"=w2600:refnum<class "State Machine.lvclass">)  [unwired: 7 in]
              n933 = Greater?(x=w2595, y=53 ("x")) -> (0:w2594:bool)
              n934 = call-dynamic "Write State Machine.vi"("error in (no error)"=w2598, "State Machine.lvclass"=w2600, "Device in"=w2603) -> ("error out"=w2602:errorcluster, "Device out"=w2604:refnum<class "Channel.lvclass">)  [unwired: 7 in]
              n935 = call-dynamic "Write Channel.vi"("error in (no error)"=w2602, "Channel.lvclass"=w2604, "Acquisition in"=w2609) -> ("error out"=w2607:errorcluster, "Acquisition out"=w2608:refnum<class "Acquisition.lvclass">)  [unwired: 7 in]
            }
          }
          n936 = call-dynamic "Write AcquisitionA.vi"("error in (no error)"=w2528, "Acquisition.lvclass"=w2530, "S4ACS_GUI in"=w2529) -> ("error out"=w2520:errorcluster, "S4ACS_GUI out"=w2519:refnum<class "S4GUI.lvclass">)  [unwired: 7 in]
          n937 = call "Read AcquisitionB.vi"("error in (no error)"=w2520, "S4ACS_GUI in"=w2519) -> ("error out"=w2495:errorcluster, "Acquisition.lvclass"=w2499:refnum<class "Acquisition.lvclass">, "S4ACS_GUI out"=w2521:refnum<class "S4GUI.lvclass">)  [unwired: 7 in]
          n938 = call "Read connection.vi"("error in (no error)"=w2495, "Server in"=w2499) -> ("error out"=w2496:errorcluster, "connection"=w2497:bool, "Server out"=w2498:refnum<class "Acquisition.lvclass">)  [unwired: 7 in]
          n939 = case shown="True" w2497 {
            tunnel: w2496 -> [w2572 w2580]
            tunnel: w2498 -> [w2573 w2579]
            tunnel: [TRUE w2574] -> w2484
            tunnel: [w2572 w2578] -> w2518
            tunnel: [w2573 w2577] -> w2517
            frame False {
            }
            frame True {
              n940 = call-dynamic "Read Channel.vi"("error in (no error)"=w2580, "Acquisition in"=w2579) -> ("error out"=w2582:errorcluster, "Channel.lvclass"=w2583:refnum<class "Channel.lvclass">, "Acquisition out"=w2581:refnum<class "Acquisition.lvclass">)  [unwired: 7 in]
              n941 = call-dynamic "Read State Machine.vi"("error in (no error)"=w2582, "Device in"=w2583) -> ("error out"=w2589:errorcluster, "State Machine.lvclass"=w2587:refnum<class "State Machine.lvclass">, "Device out"=w2585:refnum<class "Channel.lvclass">)  [unwired: 7 in]
              n942 = call-dynamic "Read State.vi"("error in (no error)"=w2589, "State Machine in"=w2587) -> ("error out"=w2590:errorcluster, "State"=w2576:i32, "State Machine out"=w2588:refnum<class "State Machine.lvclass">)  [unwired: 7 in]
              n943 = Greater?(x=w2576, y=53 ("x")) -> (0:w2574:bool)
              n944 = call-dynamic "Write State Machine.vi"("error in (no error)"=w2590, "State Machine.lvclass"=w2588, "Device in"=w2585) -> ("error out"=w2586:errorcluster, "Device out"=w2584:refnum<class "Channel.lvclass">)  [unwired: 7 in]
              n945 = call-dynamic "Write Channel.vi"("error in (no error)"=w2586, "Channel.lvclass"=w2584, "Acquisition in"=w2581) -> ("error out"=w2578:errorcluster, "Acquisition out"=w2577:refnum<class "Acquisition.lvclass">)  [unwired: 7 in]
            }
          }
          n946 = call "Write AcquisitionB.vi"("error in (no error)"=w2518, "Acquisition.lvclass"=w2517, "S4ACS_GUI in"=w2521) -> ("error out"=w2510:errorcluster, "S4ACS_GUI out"=w2509:refnum<class "S4GUI.lvclass">)  [unwired: 7 in]
          n947 = call-dynamic "Read AcquisitionC.vi"("error in (no error)"=w2510, "S4ACS_GUI in"=w2509) -> ("error out"=w2491:errorcluster, "Acquisition.lvclass"=w2494:refnum<class "Acquisition.lvclass">, "S4ACS_GUI out"=w2512:refnum<class "S4GUI.lvclass">)  [unwired: 7 in]
          n948 = call "Read connection.vi"("error in (no error)"=w2491, "Server in"=w2494) -> ("error out"=w2490:errorcluster, "connection"=w2492:bool, "Server out"=w2493:refnum<class "Acquisition.lvclass">)  [unwired: 7 in]
          n949 = case shown="True" w2492 {
            tunnel: [w2552 w2561] -> w2513
            tunnel: [w2553 w2560] -> w2511
            tunnel: w2490 -> [w2552 w2557]
            tunnel: w2493 -> [w2553 w2558]
            tunnel: [TRUE w2554] -> w2483
            frame False {
            }
            frame True {
              n950 = call-dynamic "Read Channel.vi"("error in (no error)"=w2557, "Acquisition in"=w2558) -> ("error out"=w2562:errorcluster, "Channel.lvclass"=w2563:refnum<class "Channel.lvclass">, "Acquisition out"=w2559:refnum<class "Acquisition.lvclass">)  [unwired: 7 in]
              n951 = call-dynamic "Read State Machine.vi"("error in (no error)"=w2562, "Device in"=w2563) -> ("error out"=w2569:errorcluster, "State Machine.lvclass"=w2567:refnum<class "State Machine.lvclass">, "Device out"=w2565:refnum<class "Channel.lvclass">)  [unwired: 7 in]
              n952 = call-dynamic "Read State.vi"("error in (no error)"=w2569, "State Machine in"=w2567) -> ("error out"=w2570:errorcluster, "State"=w2555:i32, "State Machine out"=w2568:refnum<class "State Machine.lvclass">)  [unwired: 7 in]
              n953 = Greater?(x=w2555, y=53 ("x")) -> (0:w2554:bool)
              n954 = call-dynamic "Write State Machine.vi"("error in (no error)"=w2570, "State Machine.lvclass"=w2568, "Device in"=w2565) -> ("error out"=w2566:errorcluster, "Device out"=w2564:refnum<class "Channel.lvclass">)  [unwired: 7 in]
              n955 = call-dynamic "Write Channel.vi"("error in (no error)"=w2566, "Channel.lvclass"=w2564, "Acquisition in"=w2559) -> ("error out"=w2561:errorcluster, "Acquisition out"=w2560:refnum<class "Acquisition.lvclass">)  [unwired: 7 in]
            }
          }
          n956 = call-dynamic "Write AcquisitionC.vi"("error in (no error)"=w2513, "Acquisition.lvclass"=w2511, "S4ACS_GUI in"=w2512) -> ("error out"=w2507:errorcluster, "S4ACS_GUI out"=w2508:refnum<class "S4GUI.lvclass">)  [unwired: 7 in]
          n957 = call-dynamic "Read AcquisitionD.vi"("error in (no error)"=w2507, "S4ACS_GUI in"=w2508) -> ("error out"=w2486:errorcluster, "Acquisition.lvclass"=w2489:refnum<class "Acquisition.lvclass">, "S4ACS_GUI out"=w2514:refnum<class "S4GUI.lvclass">)  [unwired: 7 in]
          n958 = call "Read connection.vi"("error in (no error)"=w2486, "Server in"=w2489) -> ("error out"=w2485:errorcluster, "connection"=w2487:bool, "Server out"=w2488:refnum<class "Acquisition.lvclass">)  [unwired: 7 in]
          n959 = case shown="True" w2487 {
            tunnel: [w2533 w2550] -> w2516
            tunnel: [w2532 w2549] -> w2515
            tunnel: w2488 -> [w2533 w2548]
            tunnel: w2485 -> [w2532 w2547]
            tunnel: [TRUE w2534] -> w2481
            frame False {
            }
            frame True {
              n960 = call-dynamic "Read Channel.vi"("error in (no error)"=w2547, "Acquisition in"=w2548) -> ("error out"=w2545:errorcluster, "Channel.lvclass"=w2544:refnum<class "Channel.lvclass">, "Acquisition out"=w2546:refnum<class "Acquisition.lvclass">)  [unwired: 7 in]
              n961 = call-dynamic "Read State Machine.vi"("error in (no error)"=w2545, "Device in"=w2544) -> ("error out"=w2538:errorcluster, "State Machine.lvclass"=w2540:refnum<class "State Machine.lvclass">, "Device out"=w2542:refnum<class "Channel.lvclass">)  [unwired: 7 in]
              n962 = call-dynamic "Read State.vi"("error in (no error)"=w2538, "State Machine in"=w2540) -> ("error out"=w2537:errorcluster, "State"=w2535:i32, "State Machine out"=w2539:refnum<class "State Machine.lvclass">)  [unwired: 7 in]
              n963 = Greater?(x=w2535, y=53 ("x")) -> (0:w2534:bool)
              n964 = call-dynamic "Write State Machine.vi"("error in (no error)"=w2537, "State Machine.lvclass"=w2539, "Device in"=w2542) -> ("error out"=w2541:errorcluster, "Device out"=w2543:refnum<class "Channel.lvclass">)  [unwired: 7 in]
              n965 = call-dynamic "Write Channel.vi"("error in (no error)"=w2541, "Channel.lvclass"=w2543, "Acquisition in"=w2546) -> ("error out"=w2549:errorcluster, "Acquisition out"=w2550:refnum<class "Acquisition.lvclass">)  [unwired: 7 in]
            }
          }
          n966 = call-dynamic "Write AcquisitionD.vi"("error in (no error)"=w2515, "Acquisition.lvclass"=w2516, "S4ACS_GUI in"=w2514) -> ("error out"=w2505:errorcluster, "S4ACS_GUI out"=w2506:refnum<class "S4GUI.lvclass">)  [unwired: 7 in]
          n967 = Compound Arithmetic op=AND(w2482, w2484, w2483, w2481) -> (w2480:bool)
          n968 = Increment(x=w2523) -> (x+1=w2522:u32)
          n969 = Select(t=w2522, s=w2480, f=w2523) -> (s? t:f=w2524:u32)
          n970 = Bundle By Name(cluster=w2506, "Obs_state"=w2524) -> (w2525:refnum<class "S4GUI.lvclass">)
        }
        frame 325 {
          n971 = call-dynamic "Read Sync Box.lvclass.vi"("error in (no error)"=w2623, "SPARC4_AC in"=w2624) -> ("error out"=w2615:errorcluster, "Sync Box.lvclass"=w2617:refnum<class "Sync Box.lvclass">, "SPARC4_AC out"=w2612:refnum<class "S4GUI.lvclass">)  [unwired: 7 in]
          n972 = call "Read connection.vi"("error in (no error)"=w2615, "Server in"=w2617) -> ("error out"=w2614:errorcluster, "connection"=w2613:bool, "Server out"=w2616:refnum<class "Sync Box.lvclass">)  [unwired: 7 in]
          n973 = case shown="True" w2613 {
            tunnel: w2614 -> [w2631 w2652]
            tunnel: [w2632 w2650] -> w2626
            tunnel: [w2631 w2633] -> w2625
            tunnel: w2620 -> [w2630 w2641]
            tunnel: [w2628 w2640] -> w2619
            tunnel: w2616 -> [w2632 w2639]
            tunnel: w2612 -> [w2627 w2636]
            tunnel: [w2627 w2634] -> w2611
            frame False {
              n974 = Increment(x=w2630) -> (x+1=w2629:u32)
              n975 = Increment(x=w2629) -> (x+1=w2628:u32)
            }
            frame True {
              # "Envia comando FIRE para o SyncBox"
              n976 = call-dynamic "Read Trigger.lvclass.vi"("error in (no error)"=w2652, "Sync Box in"=w2639) -> ("error out"=w2646:errorcluster, "Trigger.lvclass"=w2645:refnum<class "Trigger.lvclass">, "Sync Box out"=w2651:refnum<class "Sync Box.lvclass">)  [unwired: 7 in]
              n977 = call-dynamic "Read State Machine.vi"("error in (no error)"=w2646, "Device in"=w2645) -> ("error out"=w2647:errorcluster, "State Machine.lvclass"=w2649:refnum<class "State Machine.lvclass">, "Device out"=w2643:refnum<class "Trigger.lvclass">)  [unwired: 7 in]
              n978 = call "Next State.vi"("error in (no error)"=w2647, "New_State"=40, "State Machine in"=w2649) -> ("error out"=w2637:errorcluster, "State Machine out"=w2638:refnum<class "State Machine.lvclass">)  [unwired: 7 in]
              n979 = call-dynamic "Write State Machine.vi"("error in (no error)"=w2637, "State Machine.lvclass"=w2638, "Device in"=w2643) -> ("error out"=w2642:errorcluster, "Device out"=w2644:refnum<class "Trigger.lvclass">)  [unwired: 7 in]
              n980 = Increment(x=w2641) -> (x+1=w2640:u32)
              n981 = call-dynamic "Write Trigger.lvclass.vi"("error in (no error)"=w2642, "Trigger.lvclass"=w2644, "Sync Box in"=w2651) -> ("error out"=w2635:errorcluster, "Sync Box out"=w2650:refnum<class "Sync Box.lvclass">)  [unwired: 7 in]
              n982 = disable-structure shown="Enabled" {
                disable-tunnel: w2636 -> [w2656 w2764]
                disable-tunnel: w2635 -> [w2655 w2763]
                disable-tunnel: [w2654 w2764] -> w2634
                disable-tunnel: [w2653 w2763] -> w2633
                frame Disabled {
                  n983 = call-dynamic "Read AcquisitionA.vi"("error in (no error)"=w2655, "S4ACS_GUI in"=w2656) -> ("error out"=w2673:errorcluster, "Acquisition.lvclass"=w2676:refnum<class "Acquisition.lvclass">, "S4ACS_GUI out"=w2693:refnum<class "S4GUI.lvclass">)  [unwired: 7 in]
                  n984 = call "Read connection.vi"("error in (no error)"=w2673, "Server in"=w2676) -> ("error out"=w2672:errorcluster, "connection"=w2674:bool, "Server out"=w2675:refnum<class "Acquisition.lvclass">)  [unwired: 7 in]
                  n985 = case shown="True" w2674 {
                    tunnel: w2675 -> [w2747 w2762]
                    tunnel: w2672 -> [w2746 w2761]
                    tunnel: [w2747 w2759] -> w2694
                    tunnel: [w2746 w2758] -> w2692
                    frame False {
                    }
                    frame True {
                      # "Envia comando TRIGGER_DONE  para o Acquisition"
                      n986 = call-dynamic "Read Channel.vi"("error in (no error)"=w2761, "Acquisition in"=w2762) -> ("error out"=w2754:errorcluster, "Channel.lvclass"=w2753:refnum<class "Channel.lvclass">, "Acquisition out"=w2760:refnum<class "Acquisition.lvclass">)  [unwired: 7 in]
                      n987 = call-dynamic "Read State Machine.vi"("error in (no error)"=w2754, "Device in"=w2753) -> ("error out"=w2755:errorcluster, "State Machine.lvclass"=w2757:refnum<class "State Machine.lvclass">, "Device out"=w2751:refnum<class "Channel.lvclass">)  [unwired: 7 in]
                      n988 = call "Next State.vi"("error in (no error)"=w2755, "New_State"=40, "State Machine in"=w2757) -> ("error out"=w2748:errorcluster, "State Machine out"=w2749:refnum<class "State Machine.lvclass">)  [unwired: 7 in]
                      n989 = call-dynamic "Write State Machine.vi"("error in (no error)"=w2748, "State Machine.lvclass"=w2749, "Device in"=w2751) -> ("error out"=w2750:errorcluster, "Device out"=w2752:refnum<class "Channel.lvclass">)  [unwired: 7 in]
                      n990 = call-dynamic "Write Channel.vi"("error in (no error)"=w2750, "Channel.lvclass"=w2752, "Acquisition in"=w2760) -> ("error out"=w2758:errorcluster, "Acquisition out"=w2759:refnum<class "Acquisition.lvclass">)  [unwired: 7 in]
                    }
                  }
                  n991 = call-dynamic "Write AcquisitionA.vi"("error in (no error)"=w2692, "Acquisition.lvclass"=w2694, "S4ACS_GUI in"=w2693) -> ("error out"=w2690:errorcluster, "S4ACS_GUI out"=w2691:refnum<class "S4GUI.lvclass">)  [unwired: 7 in]
                  n992 = call "Read AcquisitionB.vi"("error in (no error)"=w2690, "S4ACS_GUI in"=w2691) -> ("error out"=w2669:errorcluster, "Acquisition.lvclass"=w2671:refnum<class "Acquisition.lvclass">, "S4ACS_GUI out"=w2688:refnum<class "S4GUI.lvclass">)  [unwired: 7 in]
                  n993 = call "Read connection.vi"("error in (no error)"=w2669, "Server in"=w2671) -> ("error out"=w2668:errorcluster, "connection"=w2667:bool, "Server out"=w2670:refnum<class "Acquisition.lvclass">)  [unwired: 7 in]
                  n994 = case shown="True" w2667 {
                    tunnel: w2670 -> [w2730 w2745]
                    tunnel: w2668 -> [w2729 w2744]
                    tunnel: [w2730 w2742] -> w2689
                    tunnel: [w2729 w2741] -> w2687
                    frame False {
                    }
                    frame True {
                      # "Envia comando TRIGGER_DONE  para o Acquisition"
                      n995 = call-dynamic "Read Channel.vi"("error in (no error)"=w2744, "Acquisition in"=w2745) -> ("error out"=w2737:errorcluster, "Channel.lvclass"=w2736:refnum<class "Channel.lvclass">, "Acquisition out"=w2743:refnum<class "Acquisition.lvclass">)  [unwired: 7 in]
                      n996 = call-dynamic "Read State Machine.vi"("error in (no error)"=w2737, "Device in"=w2736) -> ("error out"=w2738:errorcluster, "State Machine.lvclass"=w2740:refnum<class "State Machine.lvclass">, "Device out"=w2734:refnum<class "Channel.lvclass">)  [unwired: 7 in]
                      n997 = call "Next State.vi"("error in (no error)"=w2738, "New_State"=40, "State Machine in"=w2740) -> ("error out"=w2731:errorcluster, "State Machine out"=w2732:refnum<class "State Machine.lvclass">)  [unwired: 7 in]
                      n998 = call-dynamic "Write State Machine.vi"("error in (no error)"=w2731, "State Machine.lvclass"=w2732, "Device in"=w2734) -> ("error out"=w2733:errorcluster, "Device out"=w2735:refnum<class "Channel.lvclass">)  [unwired: 7 in]
                      n999 = call-dynamic "Write Channel.vi"("error in (no error)"=w2733, "Channel.lvclass"=w2735, "Acquisition in"=w2743) -> ("error out"=w2741:errorcluster, "Acquisition out"=w2742:refnum<class "Acquisition.lvclass">)  [unwired: 7 in]
                    }
                  }
                  n1000 = call "Write AcquisitionB.vi"("error in (no error)"=w2687, "Acquisition.lvclass"=w2689, "S4ACS_GUI in"=w2688) -> ("error out"=w2683:errorcluster, "S4ACS_GUI out"=w2682:refnum<class "S4GUI.lvclass">)  [unwired: 7 in]
                  n1001 = call-dynamic "Read AcquisitionC.vi"("error in (no error)"=w2683, "S4ACS_GUI in"=w2682) -> ("error out"=w2664:errorcluster, "Acquisition.lvclass"=w2666:refnum<class "Acquisition.lvclass">, "S4ACS_GUI out"=w2685:refnum<class "S4GUI.lvclass">)  [unwired: 7 in]
                  n1002 = call "Read connection.vi"("error in (no error)"=w2664, "Server in"=w2666) -> ("error out"=w2663:errorcluster, "connection"=w2662:bool, "Server out"=w2665:refnum<class "Acquisition.lvclass">)  [unwired: 7 in]
                  n1003 = case shown="True" w2662 {
                    tunnel: [w2712 w2720] -> w2686
                    tunnel: [w2713 w2719] -> w2684
                    tunnel: w2665 -> [w2713 w2717]
                    tunnel: w2663 -> [w2712 w2716]
                    frame False {
                    }
                    frame True {
                      # "Envia comando TRIGGER_DONE  para o Acquisition"
                      n1004 = call-dynamic "Read Channel.vi"("error in (no error)"=w2716, "Acquisition in"=w2717) -> ("error out"=w2724:errorcluster, "Channel.lvclass"=w2725:refnum<class "Channel.lvclass">, "Acquisition out"=w2718:refnum<class "Acquisition.lvclass">)  [unwired: 7 in]
                      n1005 = call-dynamic "Read State Machine.vi"("error in (no error)"=w2724, "Device in"=w2725) -> ("error out"=w2723:errorcluster, "State Machine.lvclass"=w2721:refnum<class "State Machine.lvclass">, "Device out"=w2727:refnum<class "Channel.lvclass">)  [unwired: 7 in]
                      n1006 = call "Next State.vi"("error in (no error)"=w2723, "New_State"=40, "State Machine in"=w2721) -> ("error out"=w2715:errorcluster, "State Machine out"=w2714:refnum<class "State Machine.lvclass">)  [unwired: 7 in]
                      n1007 = call-dynamic "Write State Machine.vi"("error in (no error)"=w2715, "State Machine.lvclass"=w2714, "Device in"=w2727) -> ("error out"=w2728:errorcluster, "Device out"=w2726:refnum<class "Channel.lvclass">)  [unwired: 7 in]
                      n1008 = call-dynamic "Write Channel.vi"("error in (no error)"=w2728, "Channel.lvclass"=w2726, "Acquisition in"=w2718) -> ("error out"=w2720:errorcluster, "Acquisition out"=w2719:refnum<class "Acquisition.lvclass">)  [unwired: 7 in]
                    }
                  }
                  n1009 = call-dynamic "Write AcquisitionC.vi"("error in (no error)"=w2686, "Acquisition.lvclass"=w2684, "S4ACS_GUI in"=w2685) -> ("error out"=w2680:errorcluster, "S4ACS_GUI out"=w2679:refnum<class "S4GUI.lvclass">)  [unwired: 7 in]
                  n1010 = call-dynamic "Read AcquisitionD.vi"("error in (no error)"=w2680, "S4ACS_GUI in"=w2679) -> ("error out"=w2659:errorcluster, "Acquisition.lvclass"=w2661:refnum<class "Acquisition.lvclass">, "S4ACS_GUI out"=w2678:refnum<class "S4GUI.lvclass">)  [unwired: 7 in]
                  n1011 = call "Read connection.vi"("error in (no error)"=w2659, "Server in"=w2661) -> ("error out"=w2658:errorcluster, "connection"=w2657:bool, "Server out"=w2660:refnum<class "Acquisition.lvclass">)  [unwired: 7 in]
                  n1012 = case shown="True" w2657 {
                    tunnel: w2658 -> [w2695 w2711]
                    tunnel: [w2695 w2710] -> w2681
                    tunnel: w2660 -> [w2696 w2701]
                    tunnel: [w2696 w2699] -> w2677
                    frame False {
                    }
                    frame True {
                      # "Envia comando TRIGGER_DONE  para o Acquisition"
                      n1013 = call-dynamic "Read Channel.vi"("error in (no error)"=w2711, "Acquisition in"=w2701) -> ("error out"=w2706:errorcluster, "Channel.lvclass"=w2705:refnum<class "Channel.lvclass">, "Acquisition out"=w2700:refnum<class "Acquisition.lvclass">)  [unwired: 7 in]
                      n1014 = call-dynamic "Read State Machine.vi"("error in (no error)"=w2706, "Device in"=w2705) -> ("error out"=w2707:errorcluster, "State Machine.lvclass"=w2709:refnum<class "State Machine.lvclass">, "Device out"=w2703:refnum<class "Channel.lvclass">)  [unwired: 7 in]
                      n1015 = call "Next State.vi"("error in (no error)"=w2707, "New_State"=40, "State Machine in"=w2709) -> ("error out"=w2697:errorcluster, "State Machine out"=w2698:refnum<class "State Machine.lvclass">)  [unwired: 7 in]
                      n1016 = call-dynamic "Write State Machine.vi"("error in (no error)"=w2697, "State Machine.lvclass"=w2698, "Device in"=w2703) -> ("error out"=w2702:errorcluster, "Device out"=w2704:refnum<class "Channel.lvclass">)  [unwired: 7 in]
                      n1017 = call-dynamic "Write Channel.vi"("error in (no error)"=w2702, "Channel.lvclass"=w2704, "Acquisition in"=w2700) -> ("error out"=w2710:errorcluster, "Acquisition out"=w2699:refnum<class "Acquisition.lvclass">)  [unwired: 7 in]
                    }
                  }
                  n1018 = call-dynamic "Write AcquisitionD.vi"("error in (no error)"=w2681, "Acquisition.lvclass"=w2677, "S4ACS_GUI in"=w2678) -> ("error out"=w2653:errorcluster, "S4ACS_GUI out"=w2654:refnum<class "S4GUI.lvclass">)  [unwired: 7 in]
                }
                frame Enabled {
                }
              }
            }
          }
          n1019 = call-dynamic "Write Sync Box.lvclass.vi"("error in (no error)"=w2625, "Sync Box.lvclass"=w2626, "SPARC4_AC in"=w2611) -> ("error out"=w2622:errorcluster, "SPARC4_AC out"=w2621:refnum<class "S4GUI.lvclass">)  [unwired: 7 in]
          n1020 = Bundle By Name(cluster=w2621, "Obs_state"=w2619) -> (w2618:refnum<class "S4GUI.lvclass">)
        }
        frame 326 {
          # "Espera terminar a execução do comando atual no SyncBox e nos \nAcquistion antes de ir ao proximo passo da Observação."
          n1021 = call-dynamic "Read Sync Box.lvclass.vi"("error in (no error)"=w2782, "SPARC4_AC in"=w2783) -> ("error out"=w2788:errorcluster, "Sync Box.lvclass"=w2789:refnum<class "Sync Box.lvclass">, "SPARC4_AC out"=w2785:refnum<class "S4GUI.lvclass">)  [unwired: 7 in]
          n1022 = call-dynamic "Read Trigger.lvclass.vi"("error in (no error)"=w2788, "Sync Box in"=w2789) -> ("error out"=w2781:errorcluster, "Trigger.lvclass"=w2780:refnum<class "Trigger.lvclass">, "Sync Box out"=w2787:refnum<class "Sync Box.lvclass">)  [unwired: 7 in]
          n1023 = call-dynamic "Read State Machine.vi"("error in (no error)"=w2781, "Device in"=w2780) -> ("error out"=w2773:errorcluster, "State Machine.lvclass"=w2775:refnum<class "State Machine.lvclass">, "Device out"=w2778:refnum<class "Trigger.lvclass">)  [unwired: 7 in]
          n1024 = call-dynamic "Read State.vi"("error in (no error)"=w2773, "State Machine in"=w2775) -> ("error out"=w2772:errorcluster, "State"=w2767:i32, "State Machine out"=w2774:refnum<class "State Machine.lvclass">)  [unwired: 7 in]
          n1025 = call-dynamic "Write State Machine.vi"("error in (no error)"=w2772, "State Machine.lvclass"=w2774, "Device in"=w2778) -> ("error out"=w2777:errorcluster, "Device out"=w2779:refnum<class "Trigger.lvclass">)  [unwired: 7 in]
          n1026 = call-dynamic "Write Trigger.lvclass.vi"("error in (no error)"=w2777, "Trigger.lvclass"=w2779, "Sync Box in"=w2787) -> ("error out"=w2784:errorcluster, "Sync Box out"=w2786:refnum<class "Sync Box.lvclass">)  [unwired: 7 in]
          n1027 = call-dynamic "Write Sync Box.lvclass.vi"("error in (no error)"=w2784, "Sync Box.lvclass"=w2786, "SPARC4_AC in"=w2785) -> ("error out"=w2765:errorcluster, "SPARC4_AC out"=w2766:refnum<class "S4GUI.lvclass">)  [unwired: 7 in]
          n1028 = Increment(x=w2770) -> (x+1=w2769:u32)
          n1029 = Equal To 0?(x=w2767) -> (x = 0?=w2768:bool)
          n1030 = Select(t=w2769, s=w2768, f=w2770) -> (s? t:f=w2771:u32)
          n1031 = Bundle By Name(cluster=w2766, "Obs_state"=w2771) -> (w2776:refnum<class "S4GUI.lvclass">)
        }
        frame 327 {
          # "Espera terminar a execução do comando atual \nantes de ir ao proximo passo da Observação."
          n1032 = Unbundle By Name(w2803) -> ("cyclesDone"=w2792:u32)
          n1033 = call-dynamic "Read AcquisitionA.vi"("error in (no error)"=w2843, "S4ACS_GUI in"=w2803) -> ("error out"=w2822:errorcluster, "Acquisition.lvclass"=w2823:refnum<class "Acquisition.lvclass">, "S4ACS_GUI out"=w2845:refnum<class "S4GUI.lvclass">)  [unwired: 7 in]
          n1034 = call "Read connection.vi"("error in (no error)"=w2822, "Server in"=w2823) -> ("error out"=w2821:errorcluster, "connection"=w2820:bool, "Server out"=w2819:refnum<class "Acquisition.lvclass">)  [unwired: 7 in]
          n1035 = case shown="True" w2820 {
            tunnel: w2821 -> [w2914 w2927]
            tunnel: [w2915 w2925] -> w2846
            tunnel: [w2914 w2924] -> w2844
            tunnel: [0 ("State") w2919] -> w2798
            tunnel: w2819 -> [w2915 w2918]
            tunnel: w2792 -> [_ w2917]
            tunnel: [TRUE w2916] -> w2802
            frame False {
            }
            frame True {
              n1036 = call-dynamic "Read Channel.vi"("error in (no error)"=w2927, "Acquisition in"=w2918) -> ("error out"=w2923:errorcluster, "Channel.lvclass"=w2922:refnum<class "Channel.lvclass">, "Acquisition out"=w2926:refnum<class "Acquisition.lvclass">)  [unwired: 7 in]
              n1037 = call-dynamic "Read CyclesDone.vi"("error in (no error)"=w2923, "Channel in"=w2922) -> ("error out"=w2920:errorcluster, "CyclesDone"=w2919:u32, "Channel out"=w2921:refnum<class "Channel.lvclass">)  [unwired: 7 in]
              n1038 = Greater?(x=w2919, y=w2917) -> (0:w2916:bool)
              n1039 = call-dynamic "Write Channel.vi"("error in (no error)"=w2920, "Channel.lvclass"=w2921, "Acquisition in"=w2926) -> ("error out"=w2924:errorcluster, "Acquisition out"=w2925:refnum<class "Acquisition.lvclass">)  [unwired: 7 in]
            }
          }
          n1040 = call-dynamic "Write AcquisitionA.vi"("error in (no error)"=w2844, "Acquisition.lvclass"=w2846, "S4ACS_GUI in"=w2845) -> ("error out"=w2839:errorcluster, "S4ACS_GUI out"=w2838:refnum<class "S4GUI.lvclass">)  [unwired: 7 in]
          n1041 = call "Read AcquisitionB.vi"("error in (no error)"=w2839, "S4ACS_GUI in"=w2838) -> ("error out"=w2814:errorcluster, "Acquisition.lvclass"=w2818:refnum<class "Acquisition.lvclass">, "S4ACS_GUI out"=w2840:refnum<class "S4GUI.lvclass">)  [unwired: 7 in]
          n1042 = call "Read connection.vi"("error in (no error)"=w2814, "Server in"=w2818) -> ("error out"=w2815:errorcluster, "connection"=w2816:bool, "Server out"=w2817:refnum<class "Acquisition.lvclass">)  [unwired: 7 in]
          n1043 = case shown="True" w2816 {
            tunnel: w2815 -> [w2898 w2911]
            tunnel: w2817 -> [w2899 w2910]
            tunnel: [0 ("State") w2902] -> w2797
            tunnel: [w2898 w2909] -> w2837
            tunnel: [w2899 w2908] -> w2836
            tunnel: w2792 -> [_ w2901]
            tunnel: [TRUE w2900] -> w2793
            frame False {
            }
            frame True {
              n1044 = call-dynamic "Read Channel.vi"("error in (no error)"=w2911, "Acquisition in"=w2910) -> ("error out"=w2906:errorcluster, "Channel.lvclass"=w2907:refnum<class "Channel.lvclass">, "Acquisition out"=w2903:refnum<class "Acquisition.lvclass">)  [unwired: 7 in]
              n1045 = call-dynamic "Read CyclesDone.vi"("error in (no error)"=w2906, "Channel in"=w2907) -> ("error out"=w2905:errorcluster, "CyclesDone"=w2902:u32, "Channel out"=w2904:refnum<class "Channel.lvclass">)  [unwired: 7 in]
              n1046 = Greater?(x=w2902, y=w2901) -> (0:w2900:bool)
              n1047 = call-dynamic "Write Channel.vi"("error in (no error)"=w2905, "Channel.lvclass"=w2904, "Acquisition in"=w2903) -> ("error out"=w2909:errorcluster, "Acquisition out"=w2908:refnum<class "Acquisition.lvclass">)  [unwired: 7 in]
            }
          }
          n1048 = Max & Min(x=w2798, y=w2797) -> (max(x,y)=w2800:u32)  [unwired: 1 out]
          n1049 = call "Write AcquisitionB.vi"("error in (no error)"=w2837, "Acquisition.lvclass"=w2836, "S4ACS_GUI in"=w2840) -> ("error out"=w2829:errorcluster, "S4ACS_GUI out"=w2828:refnum<class "S4GUI.lvclass">)  [unwired: 7 in]
          n1050 = call-dynamic "Read AcquisitionC.vi"("error in (no error)"=w2829, "S4ACS_GUI in"=w2828) -> ("error out"=w2810:errorcluster, "Acquisition.lvclass"=w2813:refnum<class "Acquisition.lvclass">, "S4ACS_GUI out"=w2831:refnum<class "S4GUI.lvclass">)  [unwired: 7 in]
          n1051 = call "Read connection.vi"("error in (no error)"=w2810, "Server in"=w2813) -> ("error out"=w2809:errorcluster, "connection"=w2811:bool, "Server out"=w2812:refnum<class "Acquisition.lvclass">)  [unwired: 7 in]
          n1052 = case shown="True" w2811 {
            tunnel: [w2882 w2895] -> w2832
            tunnel: [w2883 w2894] -> w2830
            tunnel: w2809 -> [w2882 w2891]
            tunnel: w2812 -> [w2883 w2892]
            tunnel: [0 ("State") w2890] -> w2796
            tunnel: w2792 -> [_ w2889]
            tunnel: [TRUE w2888] -> w2791
            frame False {
            }
            frame True {
              n1053 = call-dynamic "Read Channel.vi"("error in (no error)"=w2891, "Acquisition in"=w2892) -> ("error out"=w2887:errorcluster, "Channel.lvclass"=w2885:refnum<class "Channel.lvclass">, "Acquisition out"=w2893:refnum<class "Acquisition.lvclass">)  [unwired: 7 in]
              n1054 = call-dynamic "Read CyclesDone.vi"("error in (no error)"=w2887, "Channel in"=w2885) -> ("error out"=w2886:errorcluster, "CyclesDone"=w2890:u32, "Channel out"=w2884:refnum<class "Channel.lvclass">)  [unwired: 7 in]
              n1055 = Greater?(x=w2890, y=w2889) -> (0:w2888:bool)
              n1056 = call-dynamic "Write Channel.vi"("error in (no error)"=w2886, "Channel.lvclass"=w2884, "Acquisition in"=w2893) -> ("error out"=w2895:errorcluster, "Acquisition out"=w2894:refnum<class "Acquisition.lvclass">)  [unwired: 7 in]
            }
          }
          n1057 = call-dynamic "Write AcquisitionC.vi"("error in (no error)"=w2832, "Acquisition.lvclass"=w2830, "S4ACS_GUI in"=w2831) -> ("error out"=w2826:errorcluster, "S4ACS_GUI out"=w2827:refnum<class "S4GUI.lvclass">)  [unwired: 7 in]
          n1058 = call-dynamic "Read AcquisitionD.vi"("error in (no error)"=w2826, "S4ACS_GUI in"=w2827) -> ("error out"=w2805:errorcluster, "Acquisition.lvclass"=w2808:refnum<class "Acquisition.lvclass">, "S4ACS_GUI out"=w2833:refnum<class "S4GUI.lvclass">)  [unwired: 7 in]
          n1059 = call "Read connection.vi"("error in (no error)"=w2805, "Server in"=w2808) -> ("error out"=w2804:errorcluster, "connection"=w2806:bool, "Server out"=w2807:refnum<class "Acquisition.lvclass">)  [unwired: 7 in]
          n1060 = case shown="True" w2806 {
            tunnel: [w2867 w2879] -> w2835
            tunnel: [w2866 w2878] -> w2834
            tunnel: w2807 -> [w2867 w2877]
            tunnel: w2804 -> [w2866 w2876]
            tunnel: [0 ("State") w2874] -> w2795
            tunnel: w2792 -> [_ w2873]
            tunnel: [TRUE w2872] -> w2790
            frame False {
            }
            frame True {
              n1061 = call-dynamic "Read Channel.vi"("error in (no error)"=w2876, "Acquisition in"=w2877) -> ("error out"=w2871:errorcluster, "Channel.lvclass"=w2869:refnum<class "Channel.lvclass">, "Acquisition out"=w2875:refnum<class "Acquisition.lvclass">)  [unwired: 7 in]
              n1062 = call-dynamic "Read CyclesDone.vi"("error in (no error)"=w2871, "Channel in"=w2869) -> ("error out"=w2870:errorcluster, "CyclesDone"=w2874:u32, "Channel out"=w2868:refnum<class "Channel.lvclass">)  [unwired: 7 in]
              n1063 = Greater?(x=w2874, y=w2873) -> (0:w2872:bool)
              n1064 = call-dynamic "Write Channel.vi"("error in (no error)"=w2870, "Channel.lvclass"=w2868, "Acquisition in"=w2875) -> ("error out"=w2878:errorcluster, "Acquisition out"=w2879:refnum<class "Acquisition.lvclass">)  [unwired: 7 in]
            }
          }
          n1065 = Max & Min(x=w2796, y=w2795) -> (max(x,y)=w2799:u32)  [unwired: 1 out]
          n1066 = Max & Min(x=w2800, y=w2799) -> (max(x,y)=w2794:u32)  [unwired: 1 out]
          n1067 = call-dynamic "Write AcquisitionD.vi"("error in (no error)"=w2834, "Acquisition.lvclass"=w2835, "S4ACS_GUI in"=w2833) -> ("error out"=w2824:errorcluster, "S4ACS_GUI out"=w2825:refnum<class "S4GUI.lvclass">)  [unwired: 7 in]
          n1068 = Compound Arithmetic op=AND(w2802, w2793, w2791, w2790) -> (w2801:bool)
          n1069 = disable-structure shown="Enabled" {
            disable-tunnel: [w2852 w2855] -> w2842
            disable-tunnel: w2841 -> [w2850 w2854]
            disable-tunnel: w2825 -> [w2848 w2856]
            disable-tunnel: w2801 -> [w2847 w2857]
            disable-tunnel: w2794 -> [_ w2853]
            frame Disabled {
              n1070 = Increment(x=w2850) -> (x+1=w2849:u32)
              n1071 = Select(t=w2849, s=w2847, f=w2850) -> (s? t:f=w2851:u32)
              n1072 = Bundle By Name(cluster=w2848, "Obs_state"=w2851) -> (w2852:refnum<class "S4GUI.lvclass">)
            }
            frame Enabled {
              n1073 = case shown="True" w2857 {
                tunnel: w2856 -> [w2858 w2863]
                tunnel: [w2858 w2862] -> w2855
                tunnel: w2854 -> [_ w2860]
                tunnel: w2853 -> [_ w2859]
                frame False {
                }
                frame True {
                  n1074 = Increment(x=w2860) -> (x+1=w2861:u32)
                  n1075 = Bundle By Name(cluster=w2863, "Obs_state"=w2861, "cyclesDone"=w2859) -> (w2862:refnum<class "S4GUI.lvclass">)
                }
              }
            }
          }
        }
        frame 328 {
          n1076 = disable-structure shown="Enabled" {
            disable-tunnel: w2931 -> [w2945 w2958]
            disable-tunnel: w2930 -> [w2944 w2956]
            disable-tunnel: [w2943 w2956] -> w2929
            disable-tunnel: [w2941 w2957] -> w2928
            frame Disabled {
              n1077 = call-dynamic "Read ciclos.vi"("error in (no error)"=w2944, "S4ACS_GUI in"=w2945) -> ("error out"=w2933:errorcluster, "ciclos"=w2938:u32, "S4ACS_GUI out"=w2946:refnum<class "S4GUI.lvclass">)  [unwired: 7 in]
              n1078 = Decrement(x=w2938) -> (x-1=w2932:u32)
              n1079 = Greater Than 0?(x=w2932) -> (x > 0?=w2939:bool)
              n1080 = case shown="False" w2939 {
                selector: w2939 -> [w2948 w2950]
                tunnel: w2932 -> [_ w2949]
                tunnel: [w2948 w2950] -> w2937
                tunnel: [u32 0 w2949] -> w2934
                frame False {
                }
                frame True {
                }
              }
              n1081 = Select(t=u32 323, s=w2937, f=u32 0) -> (s? t:f=w2940:u32)
              n1082 = call-dynamic "Write ciclos.vi"("error in (no error)"=w2933, "ciclos"=w2934, "S4ACS_GUI in"=w2946) -> ("error out"=w2943:errorcluster, "S4ACS_GUI out"=w2942:refnum<class "S4GUI.lvclass">)  [unwired: 7 in]
              n1083 = Bundle By Name(cluster=w2942, "Obs_state"=w2940) -> (w2941:refnum<class "S4GUI.lvclass">)
            }
            frame Enabled {
              n1084 = Unbundle By Name(w2958) -> ("TotalCiclos"=w2960:u32, "cyclesDone"=w2959:u32)
              n1085 = Subtract(x=w2960, y=w2959) -> (x-y=w2955:u32)
              n1086 = Greater Than 0?(x=w2955) -> (x > 0?=w2954:bool)
              n1087 = Select(t=u32 325, s=w2954, f=u32 0) -> (s? t:f=w2953:u32)
              n1088 = Bundle By Name(cluster=w2958, "ciclos"=w2955, "Obs_state"=w2953) -> (w2957:refnum<class "S4GUI.lvclass">)
            }
          }
        }
        frame 400 {
          # "Estado de \"Pause\": fica parado aqui até o botão START seja pressionado."
        }
      }
    }
    frame Error {
    }
  }
  "error out" <- w3
  "S4ACS_GUI out" <- w1
